vi "Run.vi"(8 "error in (no error)":errorcluster, 11 "Channel in":refnum<class "Channel.lvclass">) -> (0 "error out":errorcluster, 3 "Channel out":refnum<class "Channel.lvclass">)   [LabVIEW 2018, in "Channel.lvclass"]
uses:
  Channel.lvclass
  C:/Users/devstaff/sparc4/s4gui/Versao ZeroMQ REQ-REP/SPARC4_GUI -v1.0.0/Device/Device.lvclass
  Channel.lvclass/Channel.ctl
  Interface/Interface.lvclass/Interface.ctl
  Device/Device.lvclass/Device.ctl
  StateMachine/State Machine.lvclass
  Interface/Interface.lvclass
  Device/Device.lvclass
panel:
  out "resp RESUME":string
  out "resp PAUSE":string
  out "x = y?":T1
  out "resp ABORT":string
  out "resp STOP":string
  out "resposta do STATUS":string
  out "resp INIT":string
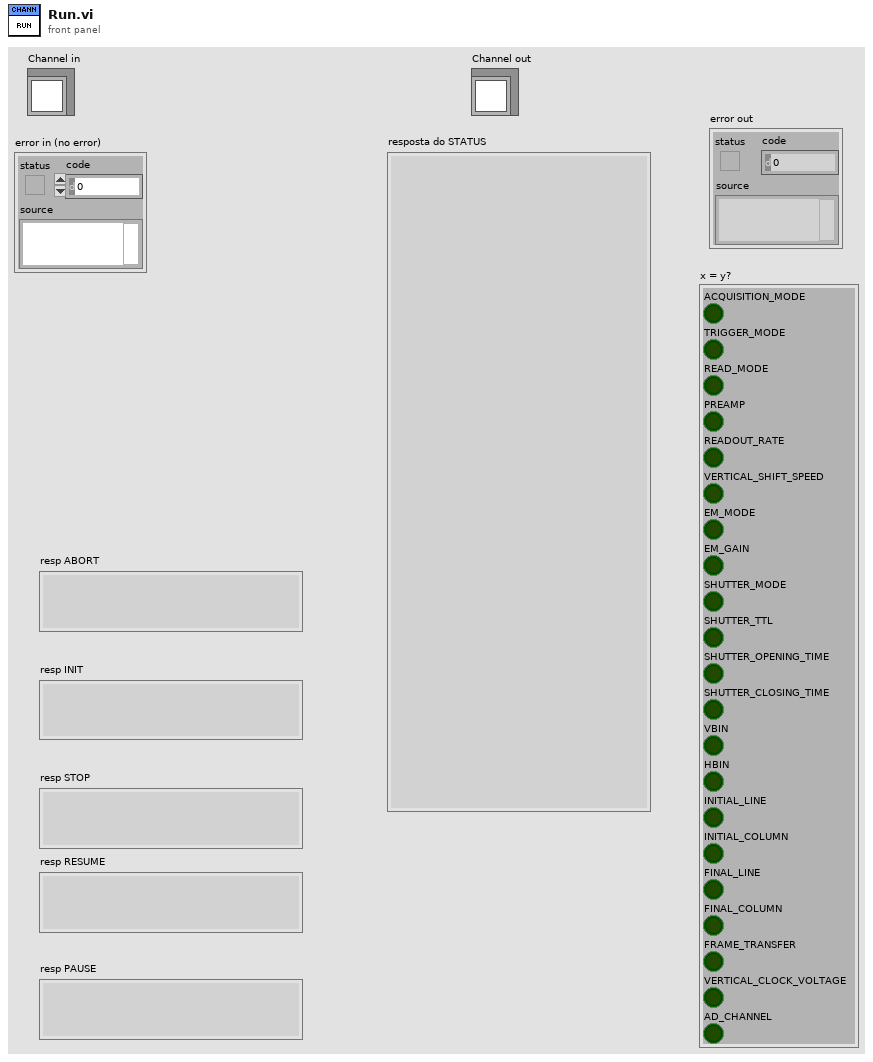
[diagram p1: front panel]
types:
  T1 = cluster{"ACQUISITION_MODE":bool, "TRIGGER_MODE":bool, "READ_MODE":bool, "PREAMP":bool, "READOUT_RATE":bool, "VERTICAL_SHIFT_SPEED":bool, "EM_MODE":bool, "EM_GAIN":bool, "SHUTTER_MODE":bool, "SHUTTER_TTL":bool, "SHUTTER_OPENING_TIME":bool, "SHUTTER_CLOSING_TIME":bool, "VBIN":bool, "HBIN":bool, "INITIAL_LINE":bool, "INITIAL_COLUMN":bool, "FINAL_LINE":bool, "FINAL_COLUMN":bool, "FRAME_TRANSFER":bool, "VERTICAL_CLOCK_VOLTAGE":bool, "AD_CHANNEL":bool}
  T2 = cluster{"TEMP":dbl, "EXPTIME":dbl, "#FRAMES":u32, "#CYCLES":u32, "#SEQS":u32, "WAVEPLATE_POS":u32, "COOLER_POWER_STATUS":dbl, "suffix":string}
  T3 = cluster{"ACQUISITION_MODE":u8, "TRIGGER_MODE":u8, "READ_MODE":u8, "PREAMP":u8, "READOUT_RATE":u8, "VERTICAL_SHIFT_SPEED":u8, "EM_MODE":u8, "EM_GAIN":u16, "SHUTTER_MODE":u8, "SHUTTER_TTL":u8, "SHUTTER_OPENING_TIME":u16, "SHUTTER_CLOSING_TIME":u16, "VBIN":u16, "HBIN":u16, "INITIAL_LINE":u16, "INITIAL_COLUMN":u16, "FINAL_LINE":u16, "FINAL_COLUMN":u16, "FRAME_TRANSFER":bool, "VERTICAL_CLOCK_VOLTAGE":u8, "AD_CHANNEL":u32}
  T4 = cluster{"Image Name":string, "Image Path":string, "#FRAMES":u32, "EXPTIME":dbl, "PREAMP":u8, "READOUT_RATE":u8, "VERTICAL_SHIFT_SPEED":u8, "ACQUISITION_MODE":u8, "READ_MODE":u8, "EM_MODE":u8, "EM_GAIN":u16, "SHUTTER_MODE":u8, "SHUTTER_TTL":u8, "SHUTTER_OPENNING_TIME":u16, "SHUTTER_CLOSING_TIME":u16, "VBIN":u16, "HBIN":u16, "INITIAL_LINE":u16, "INITIAL_COLUMN":u16, "FINAL_LINE":u16, "FINAL_COLUMN":u16, "Cooler ON/OFF":u16, "Set temperature":i8, "Exposições realizadas":u16, "Kinetic Serie Length":u32, "Number of Accumulations":u32, "Kinetic Cycle Time":u32, "FRAME_TRANSFER":bool, "VERTICAL_CLOCK_VOLTAGE":u8, "TRIGGER_MODE":u8, "Number of exp":u32, "AD_CHANNEL":u32}
  T5 = cluster{"OBSERVER":string, "OBJECT":string, "CTRLINTE":string, "PROJID":string, "SYNCMODE":string, "INSTMODE":string, "FILTER":string, "OBSTYPE":string, "CHANNEL 1":bool, "CHANNEL 2":bool, "CHANNEL 3":bool, "CHANNEL 4":bool, "TCSMODE":bool, "COMMENT":string, "broker":string, "GUIVRSN":string, "timestamp":string}
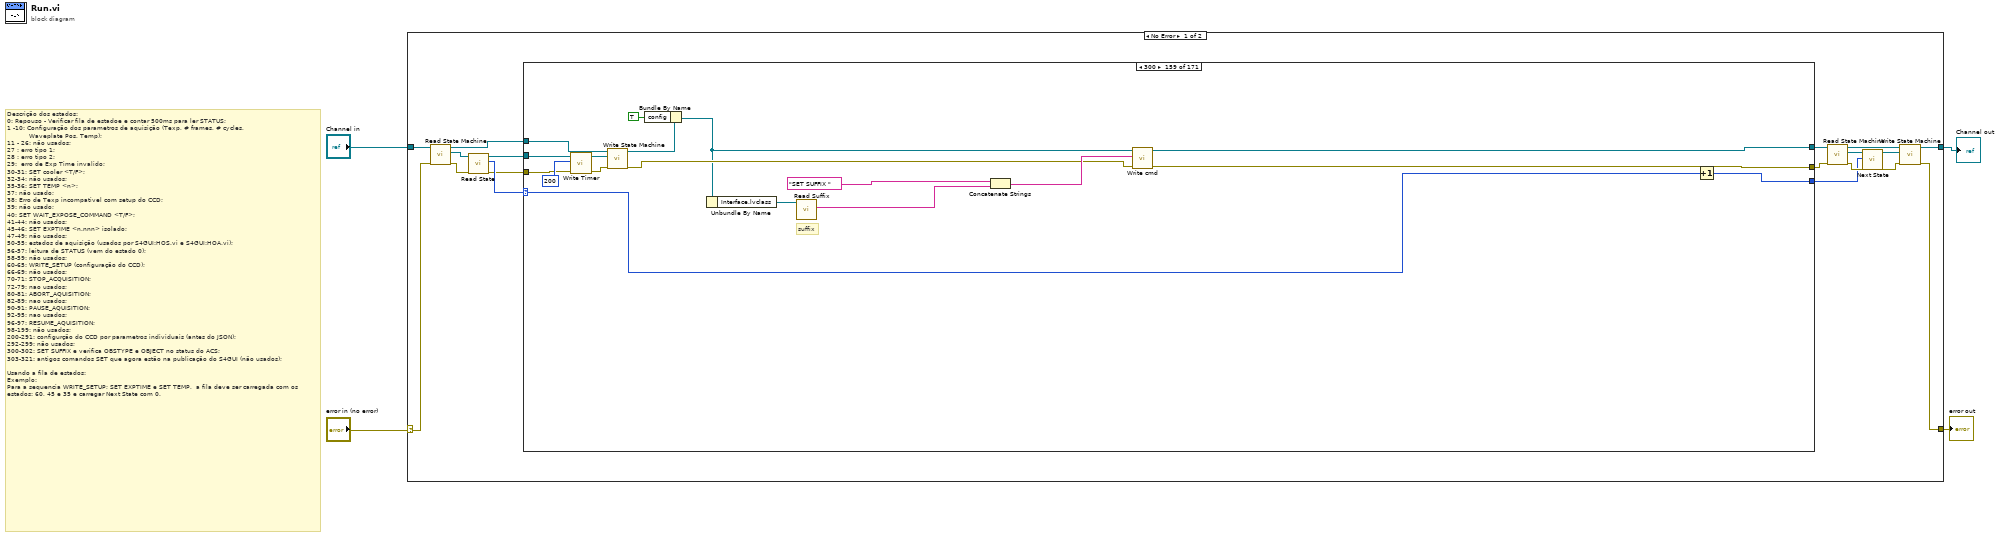
[diagram p0: block diagram]
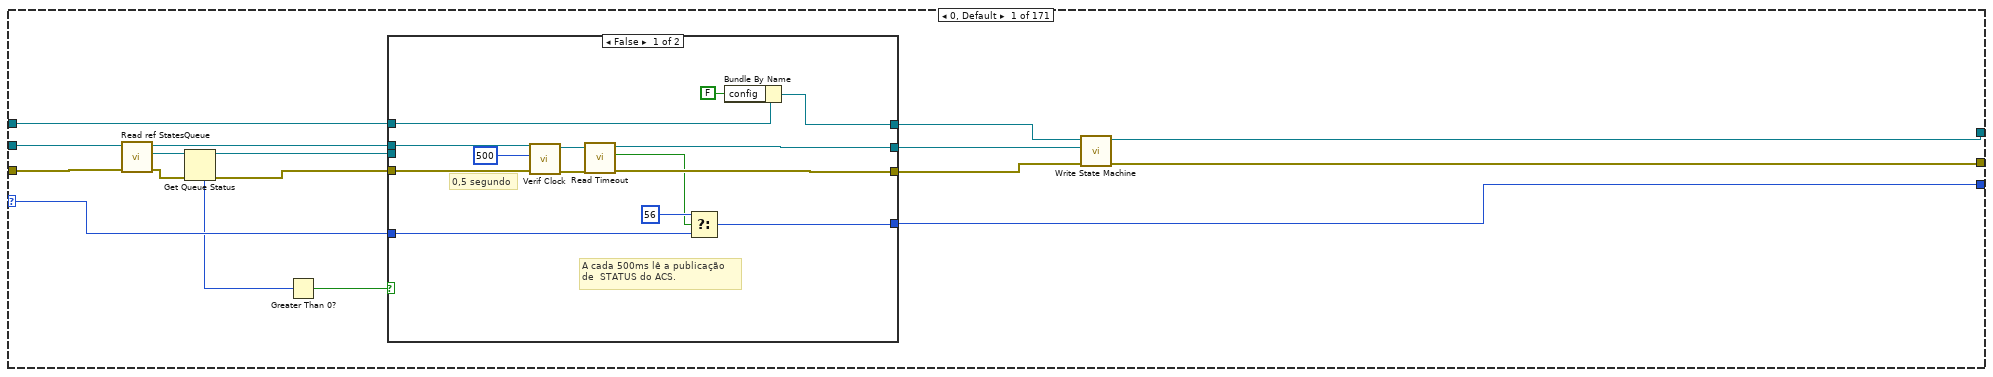
[diagram p2: hidden frame]
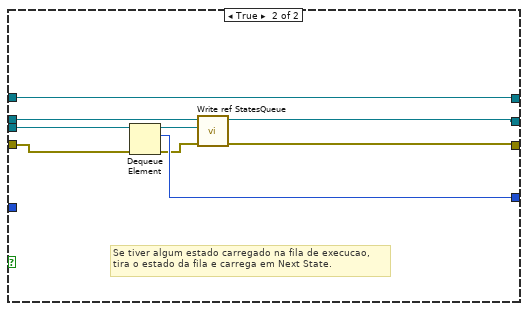
[diagram p3: hidden frame]
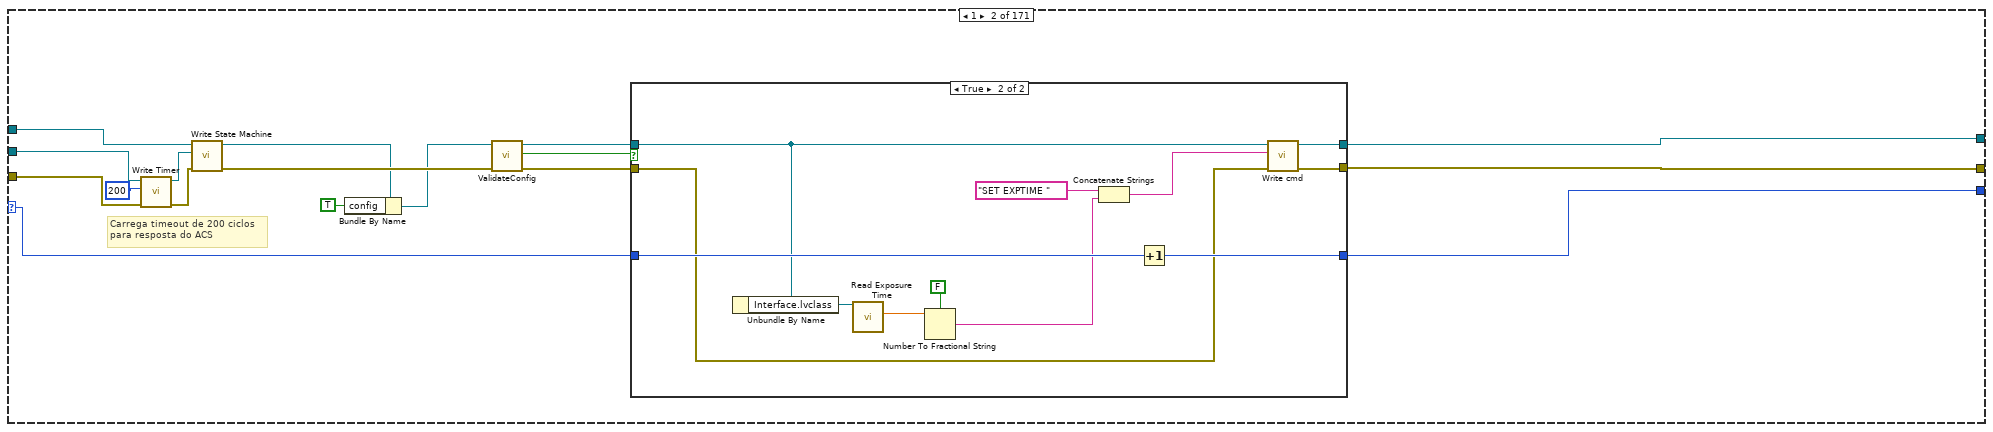
[diagram p4: hidden frame]
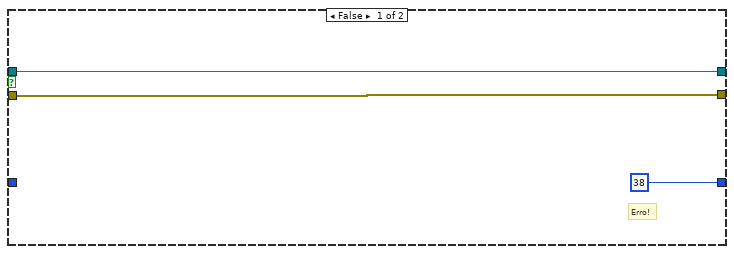
[diagram p5: hidden frame]
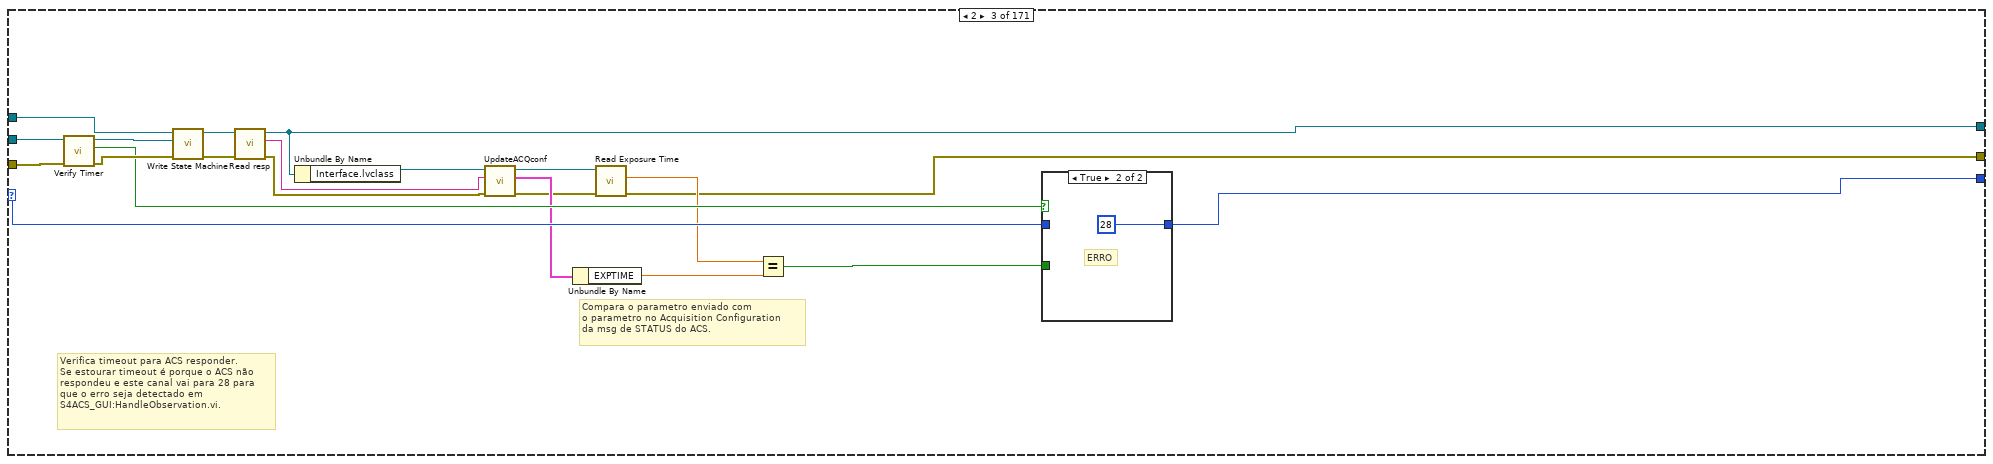
[diagram p6: hidden frame]
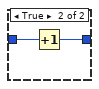
[diagram p8: hidden frame]
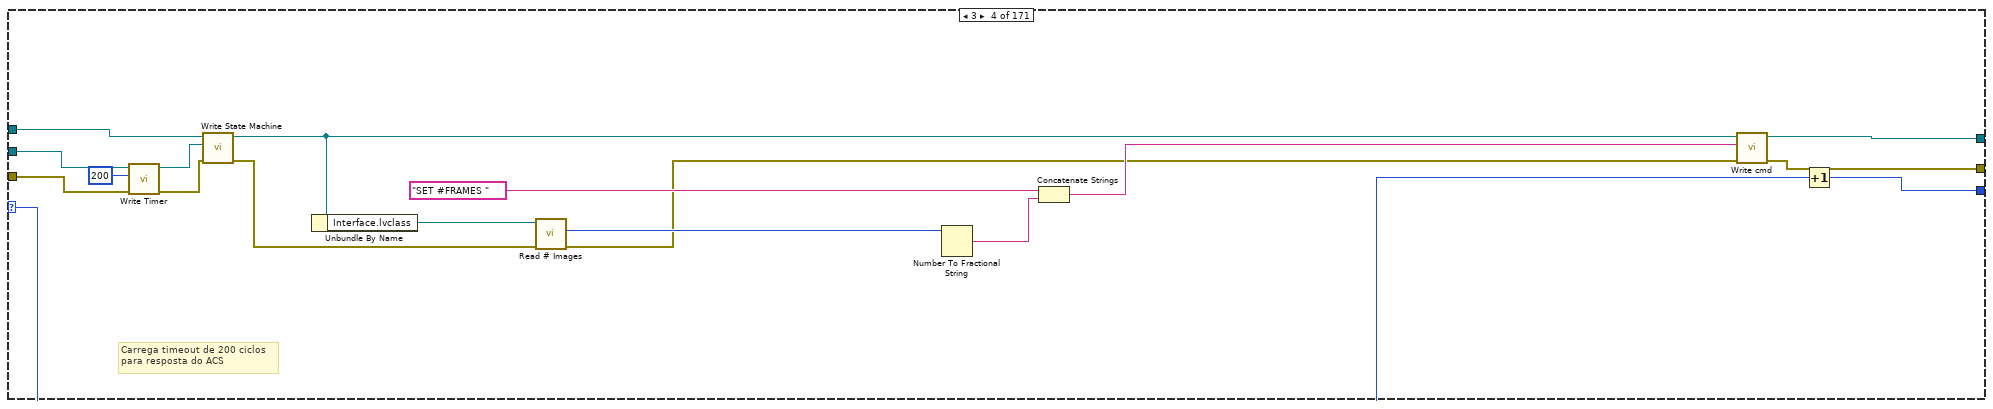
[diagram p9: hidden frame]
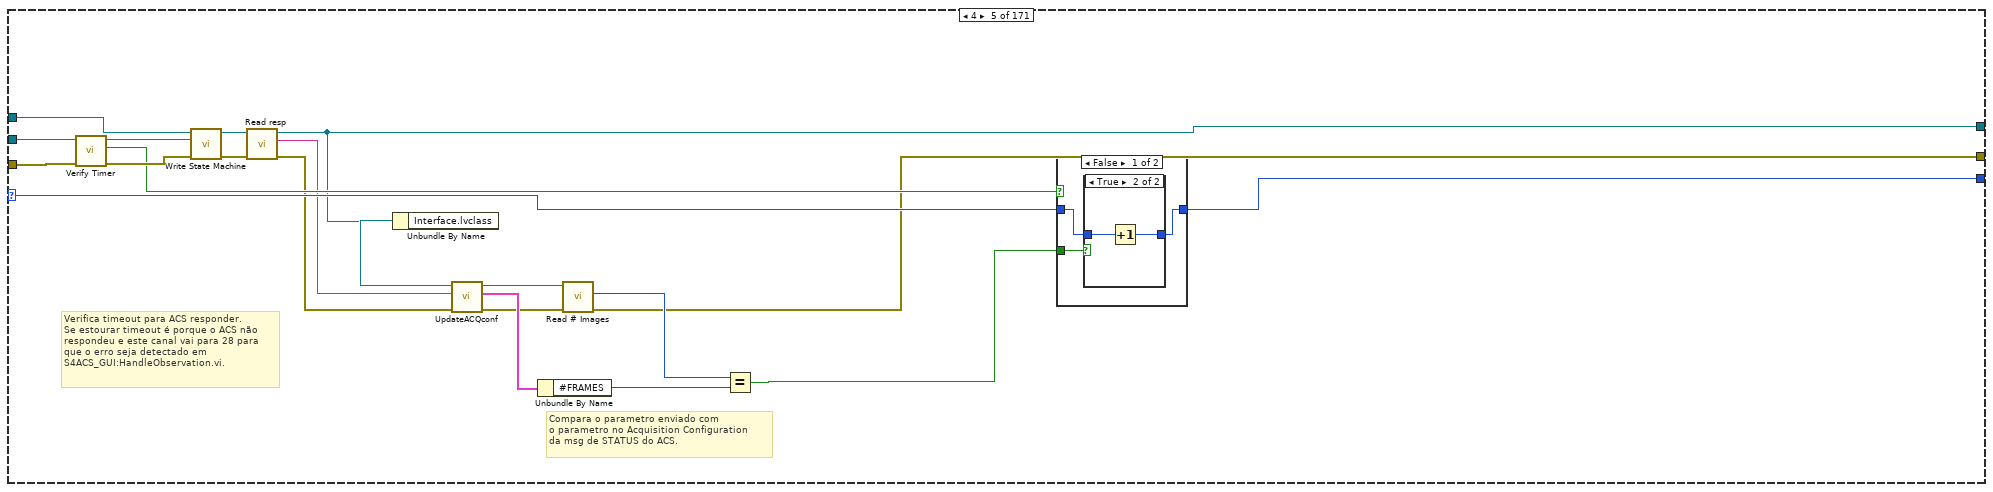
[diagram p10: hidden frame]
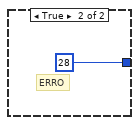
[diagram p12: hidden frame]
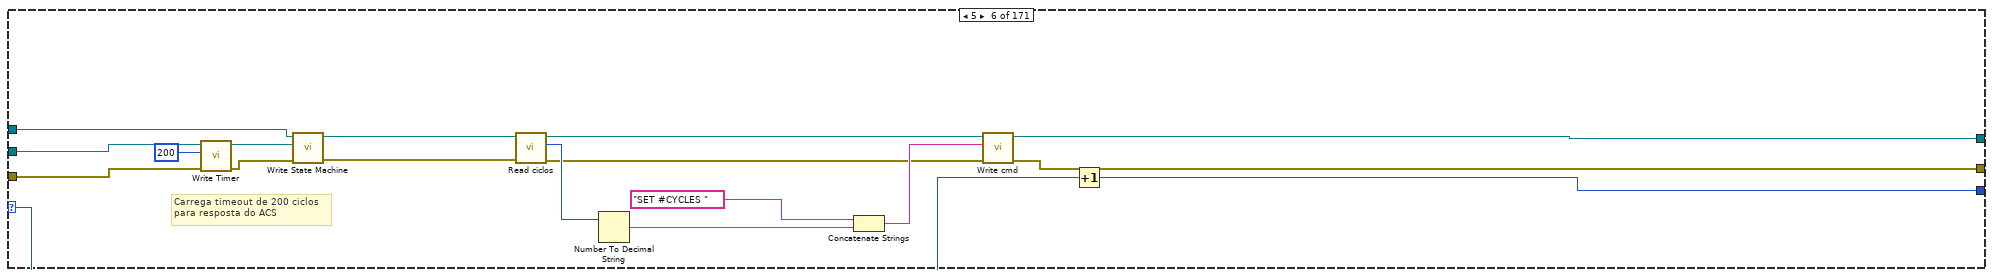
[diagram p13: hidden frame]
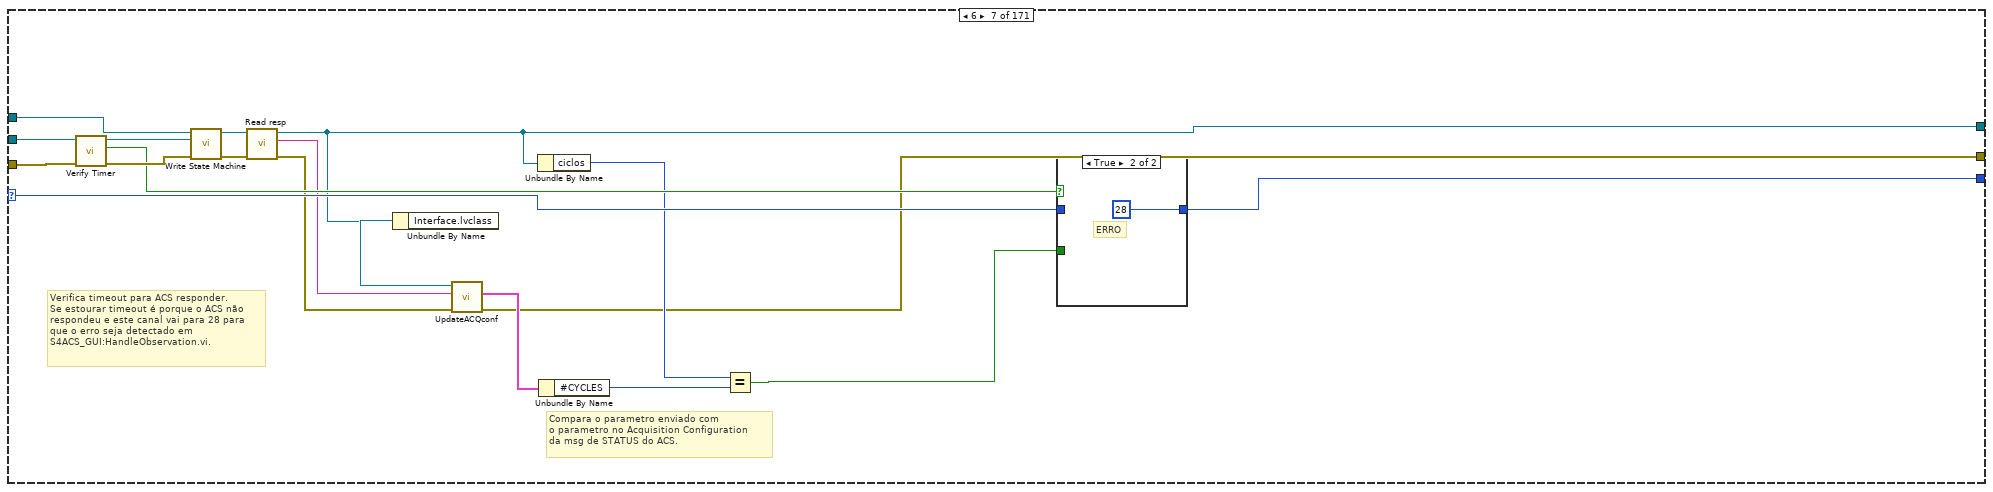
[diagram p14: hidden frame]
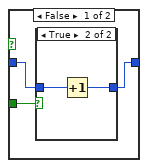
[diagram p15: hidden frame]
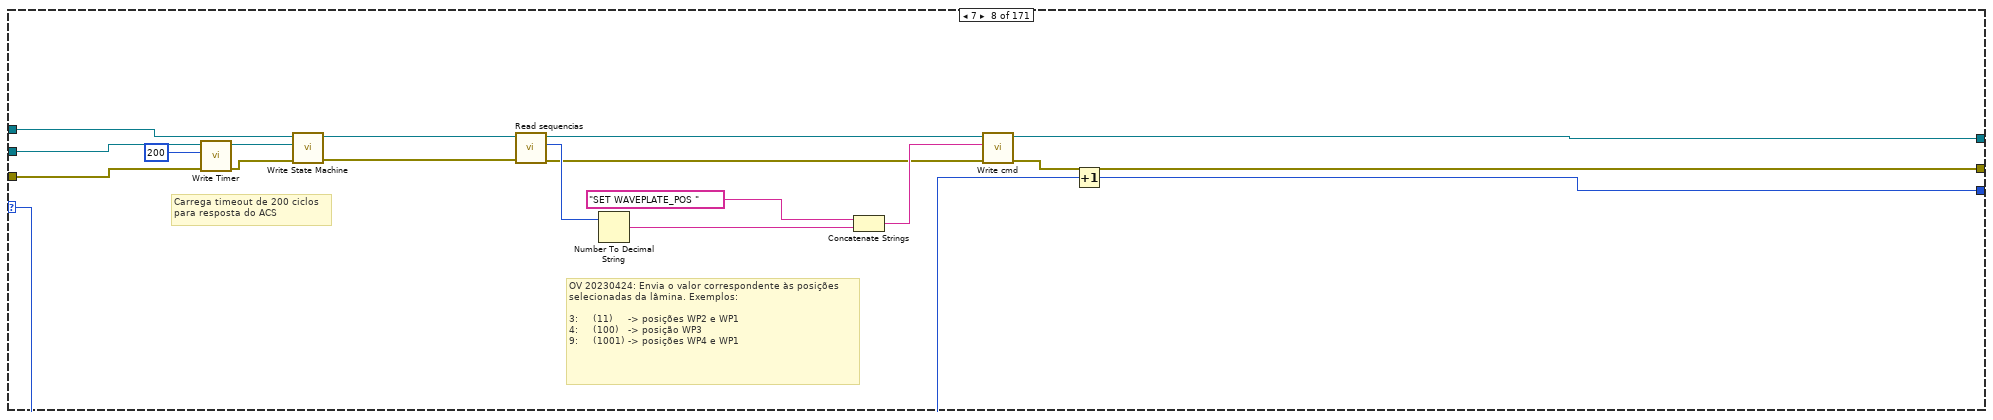
[diagram p17: hidden frame]
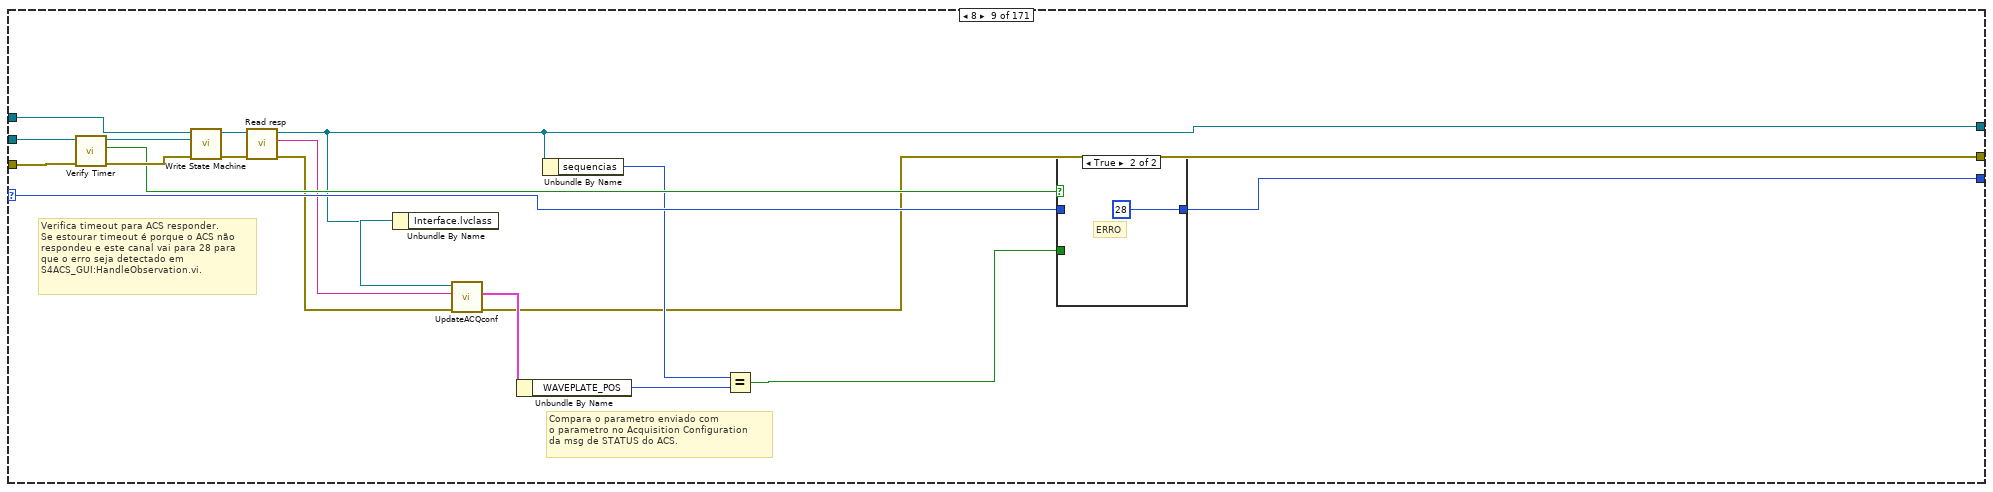
[diagram p18: hidden frame]
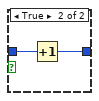
[diagram p20: hidden frame]
diagram:
  # "Descrição dos estados:\n0: Repouso - Verificar fila de estadoe e contar 500ms para ler STATUS;\n1 -10: Configuração dos parametros de aquisição (Texp, # frames, # cycles,\n           Waveplate Pos, Temp);\n11 - 26: não usados;\n27 : erro tipo 1;\n28 : erro tipo 2;\n29:  erro de Exp Time invalido;\n30-31: SET cooler <T/F>;\n32-34: não usados;\n35-36: SET TEMP <n>;\n37: não usado;\n38: Erro de Texp incompativel com setup do CCD;\n39: não usado;\n40: SET WAIT_EXPOSE_COMMAND <T/F>;\n41-44: não usados;\n45-46: SET EXPTIME <n.nnn> isolado;\n47-49: não usados;\n50-55: estados de aquisição (usados por S4GUI:HOS.vi e S4GUI:HOA.vi);\n56-57: leitura de STATUS (vem do estado 0);\n58-59: não usados;\n60-65: WRITE_SETUP (configuração do CCD);\n66-69: não usados;\n70-71: STOP_ACQUISITION;\n72-79: nao usados;\n80-81: ABORT_AQUISITION;\n82-89: nao usados;\n90-91: PAUSE_AQUISITION;\n92-95: nao usados;\n96-97: RESUME_AQUISITION;\n98-199: não usados;\n200-291: configurção do CCD por parametros individuais (antes do JSON);\n292-299: não usados;\n300-302: SET SUFFIX e verifica OBSTYPE e OBJECT no status do ACS;\n303-321: antigos comandos SET que agora estão na publicação do S4GUI (não usados);\n\nUsando a fila de estados:\nExemplo:\nPara a sequencia WRITE_SETUP; SET EXPTIME e SET TEMP,  a fila deve ser carregada com os \nestados: 60, 45 e 35 e carregar Next State com 0."
  n1 = case shown="No Error" "error in (no error)" {
    selector: "error in (no error)" -> [w21 w2964]
    tunnel: [w6 w2964] -> w3
    tunnel: [w11 w2963] -> w1
    tunnel: "Channel in" -> [w22 w2963]
    frame No Error {
      n2 = call-dynamic "Read State Machine.vi"("error in (no error)"=w21, "Device in"=w22) -> ("error out"=w18:errorcluster, "State Machine.lvclass"=w20:refnum<class "State Machine.lvclass">, "Device out"=w16:refnum<class "Channel.lvclass">)  [unwired: 7 in]
      n3 = call-dynamic "Read State.vi"("error in (no error)"=w18, "State Machine in"=w20) -> ("error out"=w17:errorcluster, "State"=w19:i32, "State Machine out"=w5:refnum<class "State Machine.lvclass">)  [unwired: 7 in]
      n4 = case shown="300" w19 {
        selector: w19 -> [w39 w76 w108 w125 w153 w177 w197 w221 w241 w265 w294 w308 w320 w350 w364 w389 w392 w395 w412 w440 w459 w472 w518 w547 _ w578 _ w619 w653 w679 w708 w719 w780 w801 w875 w915 w983 _ _ w1091 w1122 w1143 w1181 w1194 w1210 w1276 w1310 w1343 w1349 w1363 w1371 w1386 _ w1411 _ w1430 w1441 w1461 w1481 w1501 w1521 w1541 w1561 w1581 w1601 _ w1621 w1629 w1642 w1655 w1671 w1679 w1692 w1706 w1718 w1726 w1739 w1752 w1764 w1772 w1785 w1798 w1810 w1818 w1831 w1844 w1856 w1864 w1877 w1890 w1902 w1910 w1923 w1936 w1948 w1956 w1969 w1982 w1994 w2002 w2015 w2028 w2044 w2052 w2065 w2078 w2090 w2098 w2111 w2124 w2136 w2144 w2157 w2170 w2182 w2190 w2203 w2216 w2228 w2236 w2249 w2262 w2274 w2282 w2295 w2308 w2320 w2328 w2341 w2354 w2366 w2374 w2387 w2400 w2412 w2420 w2433 w2446 w2458 w2466 w2479 w2492 w2504 w2512 w2525 w2538 w2554 w2562 w2575 w2588 w2600 w2610 w2623 w2636 w2650 w2658 w2671 w2684 w2704 w2737 w2758 w2780 w2793 w2822 w2828 w2854 w2866 w2891 w2903 w2928 w2940]
        tunnel: w17 -> [w32 w75 w112 w127 w156 w179 w200 w223 w244 w262 w293 w310 w322 w352 w366 w391 w394 w397 w404 w439 w454 w466 w516 w546 w571 w580 w594 w618 w657 w676 w701 w717 w741 w798 w840 w908 w957 w1017 w1056 w1098 w1110 w1139 w1176 w1188 w1224 w1273 w1305 w1336 w1353 w1366 w1375 w1388 w1402 w1413 w1427 w1434 w1445 w1456 w1476 w1496 w1516 w1536 w1556 w1576 w1596 w1614 w1627 w1636 w1646 w1658 w1677 w1686 w1696 w1709 w1724 w1733 w1743 w1755 w1770 w1779 w1789 w1801 w1816 w1825 w1835 w1847 w1862 w1871 w1881 w1893 w1908 w1917 w1927 w1939 w1954 w1963 w1973 w1985 w2000 w2009 w2019 w2031 w2050 w2059 w2069 w2081 w2096 w2105 w2115 w2127 w2142 w2151 w2161 w2173 w2188 w2197 w2207 w2219 w2234 w2243 w2253 w2265 w2280 w2289 w2299 w2311 w2326 w2335 w2345 w2357 w2372 w2381 w2391 w2403 w2418 w2427 w2437 w2449 w2464 w2473 w2483 w2495 w2510 w2519 w2529 w2541 w2560 w2569 w2579 w2591 w2606 w2617 w2627 w2639 w2656 w2665 w2675 w2687 w2697 w2741 w2765 w2774 w2799 w2816 w2834 w2856 w2868 w2893 w2905 w2930 w2942]
        tunnel: [w35 w78 w95 w139 w141 w185 w187 w229 w231 w273 w276 w316 w329 w358 w373 w391 w394 w397 w416 w420 w461 w474 w526 w529 w576 w580 w598 w621 w640 w671 w695 w721 w772 w786 w850 w903 w958 w1029 w1067 w1097 w1123 w1144 w1173 w1196 w1211 w1278 w1292 w1324 w1350 w1359 w1372 w1383 w1400 w1408 w1422 w1433 w1442 w1456 w1476 w1496 w1516 w1536 w1556 w1576 w1596 w1614 w1626 w1630 w1645 w1656 w1676 w1680 w1695 w1707 w1723 w1727 w1742 w1753 w1769 w1773 w1788 w1799 w1815 w1819 w1834 w1845 w1861 w1865 w1880 w1891 w1907 w1911 w1926 w1937 w1953 w1957 w1972 w1983 w1999 w2003 w2018 w2029 w2049 w2053 w2068 w2079 w2095 w2099 w2114 w2125 w2141 w2145 w2160 w2171 w2187 w2191 w2206 w2217 w2233 w2237 w2252 w2263 w2279 w2283 w2298 w2309 w2325 w2329 w2344 w2355 w2371 w2375 w2390 w2401 w2417 w2421 w2436 w2447 w2463 w2467 w2482 w2493 w2509 w2513 w2528 w2539 w2559 w2563 w2578 w2589 w2605 w2611 w2626 w2637 w2655 w2659 w2674 w2685 w2708 w2723 w2761 w2783 w2802 w2824 w2837 w2862 w2875 w2899 w2912 w2936 w2949] -> w7
        tunnel: w16 -> [w24 w73 w115 w128 w160 w180 w204 w224 w248 w261 w292 w311 w326 w353 w370 w390 w393 w396 w407 w438 w456 w469 w515 w545 w574 w579 w595 w616 w660 w670 w707 w718 w754 w794 w849 w910 w951 w1028 w1066 w1092 w1114 w1137 w1177 w1189 w1225 w1272 w1308 w1337 w1354 w1365 w1376 w1380 w1403 w1405 w1428 w1432 w1446 w1454 w1474 w1494 w1514 w1534 w1554 w1574 w1594 w1616 w1625 w1637 w1644 w1659 w1675 w1687 w1694 w1710 w1722 w1734 w1741 w1756 w1768 w1780 w1787 w1802 w1814 w1826 w1833 w1848 w1860 w1872 w1879 w1894 w1906 w1918 w1925 w1940 w1952 w1964 w1971 w1986 w1998 w2010 w2017 w2032 w2048 w2060 w2067 w2082 w2094 w2106 w2113 w2128 w2140 w2152 w2159 w2174 w2186 w2198 w2205 w2220 w2232 w2244 w2251 w2266 w2278 w2290 w2297 w2312 w2324 w2336 w2343 w2358 w2370 w2382 w2389 w2404 w2416 w2428 w2435 w2450 w2462 w2474 w2481 w2496 w2508 w2520 w2527 w2542 w2558 w2570 w2577 w2592 w2604 w2618 w2625 w2640 w2654 w2666 w2673 w2688 w2698 w2744 w2764 w2776 w2800 w2818 w2835 w2857 w2872 w2894 w2909 w2931 w2946]
        tunnel: [w38 w79 w104 w140 w144 w186 w189 w230 w233 w266 w278 w317 w330 w359 w374 w390 w393 w396 w417 w421 w462 w477 w519 w531 w577 w579 w584 w622 w649 w672 w696 w722 w779 w787 w874 w904 w982 w1030 w1068 w1099 w1124 w1145 w1174 w1197 w1221 w1279 w1290 w1330 w1351 w1358 w1373 w1382 w1401 w1407 w1426 w1435 w1438 w1458 w1478 w1498 w1518 w1538 w1558 w1578 w1598 w1616 w1628 w1631 w1647 w1654 w1678 w1681 w1697 w1705 w1725 w1728 w1744 w1751 w1771 w1774 w1790 w1797 w1817 w1820 w1836 w1843 w1863 w1866 w1882 w1889 w1909 w1912 w1928 w1935 w1955 w1958 w1974 w1981 w2001 w2004 w2020 w2027 w2051 w2054 w2070 w2077 w2097 w2100 w2116 w2123 w2143 w2146 w2162 w2169 w2189 w2192 w2208 w2215 w2235 w2238 w2254 w2261 w2281 w2284 w2300 w2307 w2327 w2330 w2346 w2353 w2373 w2376 w2392 w2399 w2419 w2422 w2438 w2445 w2465 w2468 w2484 w2491 w2511 w2514 w2530 w2537 w2561 w2564 w2580 w2587 w2607 w2612 w2628 w2635 w2657 w2660 w2676 w2683 w2709 w2734 w2760 w2784 w2803 w2825 w2838 w2863 w2876 w2900 w2913 w2937 w2950] -> w14
        tunnel: [w34 w77 w107 w134 w152 w184 w196 w228 w240 w267 w295 w315 w321 w357 w362 w389 w392 w395 w413 w441 w460 w473 w520 w548 31 ("State") w578 w591 w620 w652 w677 w709 w720 w781 w802 w876 w916 w984 0 ("State") 54 ("State") w1090 w1125 w1142 w1182 w1195 w1209 w1277 w1311 w1344 w1352 w1364 w1374 w1387 0 ("State") w1412 0 ("State") w1431 w1443 w1453 w1473 w1493 w1513 w1533 w1553 w1573 w1593 u8 0 ("State") w1622 w1632 w1643 w1657 w1672 w1682 w1693 w1708 w1719 w1729 w1740 w1754 w1765 w1775 w1786 w1800 w1811 w1821 w1832 w1846 w1857 w1867 w1878 w1892 w1903 w1913 w1924 w1938 w1949 w1959 w1970 w1984 w1995 w2005 w2016 w2030 w2045 w2055 w2066 w2080 w2091 w2101 w2112 w2126 w2137 w2147 w2158 w2172 w2183 w2193 w2204 w2218 w2229 w2239 w2250 w2264 w2275 w2285 w2296 w2310 w2321 w2331 w2342 w2356 w2367 w2377 w2388 w2402 w2413 w2423 w2434 w2448 w2459 w2469 w2480 w2494 w2505 w2515 w2526 w2540 w2555 w2565 w2576 w2590 w2601 w2613 w2624 w2638 w2651 w2661 w2672 w2686 w2705 w2736 w2759 w2781 w2791 w2823 w2826 w2861 w2867 w2898 w2904 w2935 w2938] -> w8
        tunnel: w5 -> [w33 w74 w114 w129 w161 w178 w205 w222 w249 w263 w290 w309 w323 w351 w367 _ _ _ w406 w436 w455 w470 w514 w543 w573 _ w596 w617 w659 w675 w705 _ w744 w799 w842 w912 w956 w1018 w1057 w1094 w1115 w1140 w1178 w1191 w1226 w1274 w1309 w1338 _ _ _ _ _ _ _ _ _ _ _ _ _ _ _ _ _ _ _ _ _ _ _ _ _ _ _ _ _ _ _ _ _ _ _ _ _ _ _ _ _ _ _ _ _ _ _ _ _ _ _ _ _ _ _ _ _ _ _ _ _ _ _ _ _ _ _ _ _ _ _ _ _ _ _ _ _ _ _ _ _ _ _ _ _ _ _ _ _ _ _ _ _ _ _ _ _ _ _ _ _ _ _ _ _ _ _ _ _ _ w2700 w2743 w2766 w2772 w2797 w2815 w2832 w2855 w2869 w2892 w2906 w2929 w2943]
        frame 0, Default {
          n5 = call-dynamic "Read ref StatesQueue.vi"("error in (no error)"=w32, "State Machine in"=w33) -> ("error out"=w27:errorcluster, "ref StatesQueue"=w30:refnum<queue>, "State Machine out"=w31:refnum<class "State Machine.lvclass">)  [unwired: 7 in]
          n6 = Get Queue Status(queue=w30, error in (no error)=w27) -> (queue out=w25:refnum<queue>, error out=w26:errorcluster, # elements in queue=w29:i32)  [unwired: 1 in, 5 out]
          n7 = Greater Than 0?(x=w29) -> (x > 0?=w28:bool)
          n8 = case shown="False" w28 {
            tunnel: w39 -> [w49 _]
            tunnel: w31 -> [w48 w59]
            tunnel: w26 -> [w47 w61]
            tunnel: [w46 w55] -> w37
            tunnel: [w45 w56] -> w36
            tunnel: [w43 w60] -> w34
            tunnel: w25 -> [_ w62]
            tunnel: [w41 w54] -> w23
            tunnel: w24 -> [w42 w54]
            frame False {
              # "A cada 500ms lê a publicação \nde  STATUS do ACS."
              # "0,5 segundo"
              n9 = call-dynamic "Verif Clock.vi"("error in (no error)"=w47, "period (ms)"=u32 500 ("period"), "State Machine in"=w48) -> ("error out"=w52:errorcluster, "State Machine out"=w51:refnum<class "State Machine.lvclass">)  [unwired: 6 in, 1 out]
              n10 = call-dynamic "Read Timeout.vi"("error in (no error)"=w52, "State Machine in"=w51) -> ("error out"=w46:errorcluster, "Timeout"=w44:bool, "State Machine out"=w45:refnum<class "State Machine.lvclass">)  [unwired: 7 in]
              n11 = Select(t=56 ("State"), s=w44, f=w49) -> (s? t:f=w43:i32)
              n12 = Bundle By Name(cluster=w42, "config"=FALSE) -> (w41:refnum<class "Channel.lvclass">)
            }
            frame True {
              # "Se tiver algum estado carregado na fila de execucao,\ntira o estado da fila e carrega em Next State."
              n13 = Dequeue Element(queue=w62, error in (no error)=w61) -> (queue out=w58:refnum<queue>, element=w60:u32, error out=w57:errorcluster)  [unwired: 1 in, 1 out]
              n14 = call-dynamic "Write ref StatesQueue.vi"("error in (no error)"=w57, "ref StatesQueue"=w58, "State Machine in"=w59) -> ("error out"=w55:errorcluster, "State Machine out"=w56:refnum<class "State Machine.lvclass">)  [unwired: 7 in]
            }
          }
          n15 = call-dynamic "Write State Machine.vi"("error in (no error)"=w37, "State Machine.lvclass"=w36, "Device in"=w23) -> ("error out"=w35:errorcluster, "Device out"=w38:refnum<class "Channel.lvclass">)  [unwired: 7 in]
        }
        frame 1 {
          # "Carrega timeout de 200 ciclos\npara resposta do ACS"
          n16 = call-dynamic "Write Timer.vi"("error in (no error)"=w75, "Timer"=u32 200, "State Machine in"=w74) -> ("error out"=w70:errorcluster, "State Machine out"=w72:refnum<class "State Machine.lvclass">)  [unwired: 7 in]
          n17 = call-dynamic "Write State Machine.vi"("error in (no error)"=w70, "State Machine.lvclass"=w72, "Device in"=w73) -> ("error out"=w69:errorcluster, "Device out"=w65:refnum<class "Channel.lvclass">)  [unwired: 7 in]
          n18 = Bundle By Name(cluster=w65, "config"=TRUE) -> (w64:refnum<class "Channel.lvclass">)
          n19 = call-dynamic "ValidateConfig.vi"("error in (no error)"=w69, "Channel in"=w64) -> ("error out"=w67:errorcluster, "valid?"=w66:bool, "Channel out"=w68:refnum<class "Channel.lvclass">)  [unwired: 7 in]
          n20 = case shown="True" w66 {
            tunnel: [w82 w94] -> w79
            tunnel: [w81 w93] -> w78
            tunnel: [38 w92] -> w77
            tunnel: w76 -> [_ w91]
            tunnel: w68 -> [w82 w84]
            tunnel: w67 -> [w81 w83]
            frame False {
              # "Erro!"
            }
            frame True {
              n21 = Unbundle By Name(w84) -> ("Interface.lvclass"=w90:refnum<class "Interface.lvclass">)
              n22 = call "Read Exposure Time.vi"("Interface in"=w90) -> ("Exposure Time"=w89:dbl)  [unwired: 8 in, 2 out]
              n23 = Number To Fractional String(use system decimal point (T)=FALSE, number=w89) -> (F-format string=w88:string)  [unwired: 2 in]
              n24 = Concatenate Strings("SET EXPTIME " ("cmd"), w88) -> (w87:string)
              n25 = Increment(x=w91) -> (x+1=w92:i32)
              n26 = call-dynamic "Write cmd.vi"("error in (no error)"=w83, "cmd"=w87, "Device in"=w84) -> ("error out"=w93:errorcluster, "Device out"=w94:refnum<class "Channel.lvclass">)  [unwired: 7 in]
            }
          }
        }
        frame 2 {
          # "Compara o parametro enviado com\no parametro no Acquisition Configuration\nda msg de STATUS do ACS."
          # "Verifica timeout para ACS responder.\nSe estourar timeout é porque o ACS não \nrespondeu e este canal vai para 28 para \nque o erro seja detectado em\nS4ACS_GUI:HandleObservation.vi."
          n27 = call "Verify Timer.vi"("error in (no error)"=w112, "State Machine in"=w114) -> ("error out"=w111:errorcluster, "timeout"=w109:bool, "State Machine out"=w113:refnum<class "State Machine.lvclass">)  [unwired: 7 in]
          n28 = call-dynamic "Write State Machine.vi"("error in (no error)"=w111, "State Machine.lvclass"=w113, "Device in"=w115) -> ("error out"=w110:errorcluster, "Device out"=w106:refnum<class "Channel.lvclass">)  [unwired: 7 in]
          n29 = call-dynamic "Read resp.vi"("error in (no error)"=w110, "Device in"=w106) -> ("error out"=w97:errorcluster, "resp"=w105:string, "Device out"=w104:refnum<class "Channel.lvclass">)  [unwired: 7 in]
          n30 = Unbundle By Name(w104) -> ("Interface.lvclass"=w103:refnum<class "Interface.lvclass">)
          n31 = call-dynamic "UpdateACQconf.vi"("error in (no error)"=w97, "status"=w105, "Interface in"=w103) -> ("error out"=w96:errorcluster, "ACQ conf rx"=w101:T2, "Interface out"=w102:refnum<class "Interface.lvclass">)  [unwired: 6 in]
          n32 = Unbundle By Name(w101) -> ("EXPTIME"=w99:dbl)
          n33 = call "Read Exposure Time.vi"("error in (no error)"=w96, "Interface in"=w102) -> ("error out"=w95:errorcluster, "Exposure Time"=w100:dbl)  [unwired: 7 in, 1 out]
          n34 = Equal?(x=w100, y=w99) -> (x = y?=w98:bool)
          n35 = case shown="True" w109 {
            tunnel: [w117 28] -> w107
            tunnel: w108 -> [w118 _]
            tunnel: w98 -> [w116 _]
            frame False {
              n36 = case shown="False" w116 {
                tunnel: [w119 w120] -> w117
                tunnel: w118 -> [w119 w121]
                frame False {
                }
                frame True {
                  n37 = Increment(x=w121) -> (x+1=w120:i32)
                }
              }
            }
            frame True {
              # "ERRO"
            }
          }
        }
        frame 3 {
          # "Carrega timeout de 200 ciclos\npara resposta do ACS"
          n38 = call-dynamic "Write Timer.vi"("error in (no error)"=w127, "Timer"=u32 200, "State Machine in"=w129) -> ("error out"=w130:errorcluster, "State Machine out"=w132:refnum<class "State Machine.lvclass">)  [unwired: 7 in]
          n39 = call-dynamic "Write State Machine.vi"("error in (no error)"=w130, "State Machine.lvclass"=w132, "Device in"=w128) -> ("error out"=w124:errorcluster, "Device out"=w126:refnum<class "Channel.lvclass">)  [unwired: 7 in]
          n40 = Unbundle By Name(w126) -> ("Interface.lvclass"=w138:refnum<class "Interface.lvclass">)
          n41 = call-dynamic "Read # Images.vi"("error in (no error)"=w124, "Interface in"=w138) -> ("error out"=w123:errorcluster, "# Images"=w137:u32)  [unwired: 7 in, 1 out]
          n42 = Number To Fractional String(number=w137) -> (F-format string=w136:string)  [unwired: 3 in]
          n43 = Concatenate Strings("SET #FRAMES " ("cmd"), w136) -> (w135:string)
          n44 = call-dynamic "Write cmd.vi"("error in (no error)"=w123, "cmd"=w135, "Device in"=w126) -> ("error out"=w139:errorcluster, "Device out"=w140:refnum<class "Channel.lvclass">)  [unwired: 7 in]
          n45 = Increment(x=w125) -> (x+1=w134:i32)
        }
        frame 4 {
          # "Verifica timeout para ACS responder.\nSe estourar timeout é porque o ACS não \nrespondeu e este canal vai para 28 para \nque o erro seja detectado em\nS4ACS_GUI:HandleObservation.vi."
          # "Compara o parametro enviado com\no parametro no Acquisition Configuration\nda msg de STATUS do ACS."
          n46 = call "Verify Timer.vi"("error in (no error)"=w156, "State Machine in"=w161) -> ("error out"=w155:errorcluster, "timeout"=w154:bool, "State Machine out"=w157:refnum<class "State Machine.lvclass">)  [unwired: 7 in]
          n47 = call-dynamic "Write State Machine.vi"("error in (no error)"=w155, "State Machine.lvclass"=w157, "Device in"=w160) -> ("error out"=w158:errorcluster, "Device out"=w159:refnum<class "Channel.lvclass">)  [unwired: 7 in]
          n48 = call-dynamic "Read resp.vi"("error in (no error)"=w158, "Device in"=w159) -> ("error out"=w142:errorcluster, "resp"=w143:string, "Device out"=w144:refnum<class "Channel.lvclass">)  [unwired: 7 in]
          n49 = Unbundle By Name(w144) -> ("Interface.lvclass"=w151:refnum<class "Interface.lvclass">)
          n50 = call-dynamic "UpdateACQconf.vi"("error in (no error)"=w142, "status"=w143, "Interface in"=w151) -> ("error out"=w146:errorcluster, "ACQ conf rx"=w149:T2, "Interface out"=w150:refnum<class "Interface.lvclass">)  [unwired: 6 in]
          n51 = Unbundle By Name(w149) -> ("#FRAMES"=w147:u32)
          n52 = call-dynamic "Read # Images.vi"("error in (no error)"=w146, "Interface in"=w150) -> ("error out"=w141:errorcluster, "# Images"=w148:u32)  [unwired: 7 in, 1 out]
          n53 = Equal?(x=w148, y=w147) -> (x = y?=w145:bool)
          n54 = case shown="False" w154 {
            tunnel: [w163 28] -> w152
            tunnel: w153 -> [w164 _]
            tunnel: w145 -> [w162 _]
            frame False {
              n55 = case shown="True" w162 {
                tunnel: [w165 w166] -> w163
                tunnel: w164 -> [w165 w167]
                frame False {
                }
                frame True {
                  n56 = Increment(x=w167) -> (x+1=w166:i32)
                }
              }
            }
            frame True {
              # "ERRO"
            }
          }
        }
        frame 5 {
          # "Carrega timeout de 200 ciclos\npara resposta do ACS"
          n57 = call-dynamic "Write Timer.vi"("error in (no error)"=w179, "Timer"=u32 200, "State Machine in"=w178) -> ("error out"=w181:errorcluster, "State Machine out"=w183:refnum<class "State Machine.lvclass">)  [unwired: 7 in]
          n58 = call-dynamic "Write State Machine.vi"("error in (no error)"=w181, "State Machine.lvclass"=w183, "Device in"=w180) -> ("error out"=w175:errorcluster, "Device out"=w176:refnum<class "Channel.lvclass">)  [unwired: 7 in]
          n59 = call-dynamic "Read ciclos.vi"("error in (no error)"=w175, "Channel in"=w176) -> ("error out"=w169:errorcluster, "ciclos"=w173:u32, "Channel out"=w174:refnum<class "Channel.lvclass">)  [unwired: 7 in]
          n60 = Number To Decimal String(number=w173) -> (decimal integer string=w171:string)  [unwired: 1 in]
          n61 = Concatenate Strings("SET #CYCLES " ("cmd"), w171) -> (w170:string)
          n62 = call-dynamic "Write cmd.vi"("error in (no error)"=w169, "cmd"=w170, "Device in"=w174) -> ("error out"=w185:errorcluster, "Device out"=w186:refnum<class "Channel.lvclass">)  [unwired: 7 in]
          n63 = Increment(x=w177) -> (x+1=w184:i32)
        }
        frame 6 {
          # "Verifica timeout para ACS responder.\nSe estourar timeout é porque o ACS não \nrespondeu e este canal vai para 28 para \nque o erro seja detectado em\nS4ACS_GUI:HandleObservation.vi."
          # "Compara o parametro enviado com\no parametro no Acquisition Configuration\nda msg de STATUS do ACS."
          n64 = call "Verify Timer.vi"("error in (no error)"=w200, "State Machine in"=w205) -> ("error out"=w199:errorcluster, "timeout"=w198:bool, "State Machine out"=w201:refnum<class "State Machine.lvclass">)  [unwired: 7 in]
          n65 = call-dynamic "Write State Machine.vi"("error in (no error)"=w199, "State Machine.lvclass"=w201, "Device in"=w204) -> ("error out"=w202:errorcluster, "Device out"=w203:refnum<class "Channel.lvclass">)  [unwired: 7 in]
          n66 = call-dynamic "Read resp.vi"("error in (no error)"=w202, "Device in"=w203) -> ("error out"=w190:errorcluster, "resp"=w191:string, "Device out"=w189:refnum<class "Channel.lvclass">)  [unwired: 7 in]
          n67 = Unbundle By Name(w189) -> ("Interface.lvclass"=w195:refnum<class "Interface.lvclass">)
          n68 = call-dynamic "UpdateACQconf.vi"("error in (no error)"=w190, "status"=w191, "Interface in"=w195) -> ("error out"=w187:errorcluster, "ACQ conf rx"=w194:T2)  [unwired: 6 in, 1 out]
          n69 = Unbundle By Name(w189) -> ("ciclos"=w188:u32)
          n70 = Unbundle By Name(w194) -> ("#CYCLES"=w193:u32)
          n71 = Equal?(x=w188, y=w193) -> (x = y?=w192:bool)
          n72 = case shown="True" w198 {
            tunnel: [w207 28] -> w196
            tunnel: w197 -> [w208 _]
            tunnel: w192 -> [w206 _]
            frame False {
              n73 = case shown="True" w206 {
                tunnel: [w209 w210] -> w207
                tunnel: w208 -> [w209 w211]
                frame False {
                }
                frame True {
                  n74 = Increment(x=w211) -> (x+1=w210:i32)
                }
              }
            }
            frame True {
              # "ERRO"
            }
          }
        }
        frame 7 {
          # "OV 20230424: Envia o valor correspondente às posições\nselecionadas da lâmina. Exemplos:\n\n3:     (11)     -> posições WP2 e WP1\n4:     (100)   -> posição WP3\n9:     (1001) -> posições WP4 e WP1"
          # "Carrega timeout de 200 ciclos\npara resposta do ACS"
          n75 = call-dynamic "Write Timer.vi"("error in (no error)"=w223, "Timer"=u32 200, "State Machine in"=w222) -> ("error out"=w225:errorcluster, "State Machine out"=w227:refnum<class "State Machine.lvclass">)  [unwired: 7 in]
          n76 = call-dynamic "Write State Machine.vi"("error in (no error)"=w225, "State Machine.lvclass"=w227, "Device in"=w224) -> ("error out"=w219:errorcluster, "Device out"=w220:refnum<class "Channel.lvclass">)  [unwired: 7 in]
          n77 = call-dynamic "Read sequencias.vi"("error in (no error)"=w219, "Channel in"=w220) -> ("error out"=w213:errorcluster, "sequencias"=w217:u32, "Channel out"=w218:refnum<class "Channel.lvclass">)  [unwired: 7 in]
          n78 = Number To Decimal String(number=w217) -> (decimal integer string=w215:string)  [unwired: 1 in]
          n79 = Concatenate Strings("SET WAVEPLATE_POS " ("cmd"), w215) -> (w214:string)
          n80 = call-dynamic "Write cmd.vi"("error in (no error)"=w213, "cmd"=w214, "Device in"=w218) -> ("error out"=w229:errorcluster, "Device out"=w230:refnum<class "Channel.lvclass">)  [unwired: 7 in]
          n81 = Increment(x=w221) -> (x+1=w228:i32)
        }
        frame 8 {
          # "Verifica timeout para ACS responder.\nSe estourar timeout é porque o ACS não \nrespondeu e este canal vai para 28 para \nque o erro seja detectado em\nS4ACS_GUI:HandleObservation.vi."
          # "Compara o parametro enviado com\no parametro no Acquisition Configuration\nda msg de STATUS do ACS."
          n82 = call "Verify Timer.vi"("error in (no error)"=w244, "State Machine in"=w249) -> ("error out"=w243:errorcluster, "timeout"=w242:bool, "State Machine out"=w245:refnum<class "State Machine.lvclass">)  [unwired: 7 in]
          n83 = call-dynamic "Write State Machine.vi"("error in (no error)"=w243, "State Machine.lvclass"=w245, "Device in"=w248) -> ("error out"=w246:errorcluster, "Device out"=w247:refnum<class "Channel.lvclass">)  [unwired: 7 in]
          n84 = call-dynamic "Read resp.vi"("error in (no error)"=w246, "Device in"=w247) -> ("error out"=w234:errorcluster, "resp"=w235:string, "Device out"=w233:refnum<class "Channel.lvclass">)  [unwired: 7 in]
          n85 = Unbundle By Name(w233) -> ("Interface.lvclass"=w239:refnum<class "Interface.lvclass">)
          n86 = call-dynamic "UpdateACQconf.vi"("error in (no error)"=w234, "status"=w235, "Interface in"=w239) -> ("error out"=w231:errorcluster, "ACQ conf rx"=w238:T2)  [unwired: 6 in, 1 out]
          n87 = Unbundle By Name(w238) -> ("WAVEPLATE_POS"=w237:u32)
          n88 = Unbundle By Name(w233) -> ("sequencias"=w232:u32)
          n89 = Equal?(x=w232, y=w237) -> (x = y?=w236:bool)
          n90 = case shown="True" w242 {
            tunnel: [w251 28] -> w240
            tunnel: w241 -> [w252 _]
            tunnel: w236 -> [w250 _]
            frame False {
              n91 = case shown="False" w250 {
                tunnel: [w253 w254] -> w251
                tunnel: w252 -> [w253 w255]
                frame False {
                }
                frame True {
                  n92 = Increment(x=w255) -> (x+1=w254:i32)
                }
              }
            }
            frame True {
              # "ERRO"
            }
          }
        }
        frame 9 {
          # "Carrega timeout de 200 ciclos\npara resposta do ACS"
          n93 = call-dynamic "Write Timer.vi"("error in (no error)"=w262, "Timer"=u32 200, "State Machine in"=w263) -> ("error out"=w259:errorcluster, "State Machine out"=w260:refnum<class "State Machine.lvclass">)  [unwired: 7 in]
          n94 = call-dynamic "Write State Machine.vi"("error in (no error)"=w259, "State Machine.lvclass"=w260, "Device in"=w261) -> ("error out"=w257:errorcluster, "Device out"=w258:refnum<class "Channel.lvclass">)  [unwired: 7 in]
          n95 = Unbundle By Name(w258) -> ("Interface.lvclass"=w272:refnum<class "Interface.lvclass">)
          n96 = call-dynamic "Read Temperature.vi"("Interface in"=w272) -> ("Temperature"=w269:i8)  [unwired: 8 in, 2 out]
          n97 = Number To Decimal String(number=w269) -> (decimal integer string=w268:string)  [unwired: 1 in]
          n98 = Concatenate Strings("SET TEMP " ("cmd"), w268) -> (w271:string)
          n99 = call-dynamic "Write cmd.vi"("error in (no error)"=w257, "cmd"=w271, "Device in"=w258) -> ("error out"=w273:errorcluster, "Device out"=w266:refnum<class "Channel.lvclass">)  [unwired: 7 in]
          n100 = Increment(x=w265) -> (x+1=w267:i32)
        }
        frame 10 {
          # "Verifica timeout para ACS responder.\nSe estourar timeout é porque o ACS não \nrespondeu e este canal vai para 28 para \nque o erro seja detectado em\nS4ACS_GUI:HandleObservation.vi."
          n101 = call "Verify Timer.vi"("error in (no error)"=w293, "State Machine in"=w290) -> ("error out"=w288:errorcluster, "timeout"=w286:bool, "State Machine out"=w289:refnum<class "State Machine.lvclass">)  [unwired: 7 in]
          n102 = call-dynamic "Write State Machine.vi"("error in (no error)"=w288, "State Machine.lvclass"=w289, "Device in"=w292) -> ("error out"=w287:errorcluster, "Device out"=w291:refnum<class "Channel.lvclass">)  [unwired: 7 in]
          n103 = call-dynamic "Read resp.vi"("error in (no error)"=w287, "Device in"=w291) -> ("error out"=w277:errorcluster, "resp"=w279:string, "Device out"=w278:refnum<class "Channel.lvclass">)  [unwired: 7 in]
          n104 = Unbundle By Name(w278) -> ("Interface.lvclass"=w285:refnum<class "Interface.lvclass">)
          n105 = call-dynamic "UpdateACQconf.vi"("error in (no error)"=w277, "status"=w279, "Interface in"=w285) -> ("error out"=w281:errorcluster, "ACQ conf rx"=w284:T2, "Interface out"=w282:refnum<class "Interface.lvclass">)  [unwired: 6 in]
          n106 = Unbundle By Name(w284) -> ("TEMP"=w275:dbl)
          n107 = call-dynamic "Read Temperature.vi"("error in (no error)"=w281, "Interface in"=w282) -> ("error out"=w276:errorcluster, "Temperature"=w280:i8)  [unwired: 7 in, 1 out]
          n108 = To Byte Integer(number=w275) -> (8bit integer=w274:i8)
          n109 = Equal?(x=w280, y=w274) -> (x = y?=w283:bool)
          n110 = case shown="False" w286 {
            tunnel: w283 -> [w298 _]
            tunnel: [w297 28 ("State")] -> w295
            tunnel: w294 -> [w296 _]
            frame False {
              n111 = case shown="True" w298 {
                tunnel: [w299 0 ("State")] -> w297
                tunnel: w296 -> [w299 _]
                frame False {
                }
                frame True {
                  # "OV 2024-04-2: Apenas seta a temperatura, pois \ncooler já está ligado. Fim do setup inicial para aquisição."
                }
              }
            }
            frame True {
              # "ERRO"
              # "Estourou timeour e ACS não recebeu\no valor da temperatura desejada.\nAborta o processo com erro de \nconfiguração"
            }
          }
        }
        frame 11 {
          # "Carrega timeout de 50 ciclos\npara resposta do ACS"
          n112 = call-dynamic "Write Timer.vi"("error in (no error)"=w310, "Timer"=u32 50, "State Machine in"=w309) -> ("error out"=w312:errorcluster, "State Machine out"=w314:refnum<class "State Machine.lvclass">)  [unwired: 7 in]
          n113 = call-dynamic "Write State Machine.vi"("error in (no error)"=w312, "State Machine.lvclass"=w314, "Device in"=w311) -> ("error out"=w305:errorcluster, "Device out"=w304:refnum<class "Channel.lvclass">)  [unwired: 7 in]
          n114 = Unbundle By Name(w304) -> ("Channel Status"=w303:u32)
          n115 = Number To Decimal String(number=w303) -> (decimal integer string=w302:string)  [unwired: 1 in]
          n116 = Concatenate Strings("SET CHANNELSST " ("cmd"), w302) -> (w306:string)
          n117 = call-dynamic "Write cmd.vi"("error in (no error)"=w305, "cmd"=w306, "Device in"=w304) -> ("error out"=w316:errorcluster, "Device out"=w317:refnum<class "Channel.lvclass">)  [unwired: 7 in]
          n118 = Increment(x=w308) -> (x+1=w315:i32)
        }
        frame 12 {
          n119 = call "Verify Timer.vi"("error in (no error)"=w322, "State Machine in"=w323) -> ("error out"=w327:errorcluster, "timeout"=w319:bool, "State Machine out"=w328:refnum<class "State Machine.lvclass">)  [unwired: 7 in]
          n120 = call-dynamic "Write State Machine.vi"("error in (no error)"=w327, "State Machine.lvclass"=w328, "Device in"=w326) -> ("error out"=w324:errorcluster, "Device out"=w325:refnum<class "Channel.lvclass">)  [unwired: 7 in]
          n121 = call-dynamic "Read resp.vi"("error in (no error)"=w324, "Device in"=w325) -> ("error out"=w329:errorcluster, "resp"=w332:string, "Device out"=w330:refnum<class "Channel.lvclass">)  [unwired: 7 in]
          n122 = Equal?(x=w332, y="DONE") -> (x = y?=w318:bool)
          n123 = case shown="True" w319 {
            tunnel: [w334 w340] -> w321
            tunnel: w320 -> [w335 w339]
            tunnel: w318 -> [w333 _]
            frame False {
              n124 = case shown="True" w333 {
                tunnel: [w336 w337] -> w334
                tunnel: w335 -> [w336 w338]
                frame False {
                }
                frame True {
                  n125 = Increment(x=w338) -> (x+1=w337:i32)
                }
              }
            }
            frame True {
              n126 = disable-structure shown="Enabled" {
                disable-tunnel: [28 w342] -> w340
                disable-tunnel: w339 -> [_ w343]
                frame Enabled {
                  # "ERRO"
                }
                frame Disabled {
                  # "Por enquanto, prossegue\nmesmo sem receber DONE."
                  n127 = Increment(x=w343) -> (x+1=w342:i32)
                }
              }
            }
          }
        }
        frame 13 {
          # "Carrega timeout de 50 ciclos\npara resposta do ACS"
          n128 = call-dynamic "Write Timer.vi"("error in (no error)"=w352, "Timer"=u32 50, "State Machine in"=w351) -> ("error out"=w354:errorcluster, "State Machine out"=w356:refnum<class "State Machine.lvclass">)  [unwired: 7 in]
          n129 = call-dynamic "Write State Machine.vi"("error in (no error)"=w354, "State Machine.lvclass"=w356, "Device in"=w353) -> ("error out"=w347:errorcluster, "Device out"=w346:refnum<class "Channel.lvclass">)  [unwired: 7 in]
          n130 = Unbundle By Name(w346) -> ("syncmode"=w345:bool)
          n131 = case shown="False" w345 {
            tunnel: ["ASYNC" "SYNC"] -> w344
            frame False {
            }
            frame True {
            }
          }
          n132 = Concatenate Strings("SET SYNCMODE " ("cmd"), w344) -> (w348:string)
          n133 = call-dynamic "Write cmd.vi"("error in (no error)"=w347, "cmd"=w348, "Device in"=w346) -> ("error out"=w358:errorcluster, "Device out"=w359:refnum<class "Channel.lvclass">)  [unwired: 7 in]
          n134 = Increment(x=w350) -> (x+1=w357:i32)
        }
        frame 14 {
          n135 = call "Verify Timer.vi"("error in (no error)"=w366, "State Machine in"=w367) -> ("error out"=w371:errorcluster, "timeout"=w365:bool, "State Machine out"=w372:refnum<class "State Machine.lvclass">)  [unwired: 7 in]
          n136 = call-dynamic "Write State Machine.vi"("error in (no error)"=w371, "State Machine.lvclass"=w372, "Device in"=w370) -> ("error out"=w368:errorcluster, "Device out"=w369:refnum<class "Channel.lvclass">)  [unwired: 7 in]
          n137 = call-dynamic "Read resp.vi"("error in (no error)"=w368, "Device in"=w369) -> ("error out"=w373:errorcluster, "resp"=w376:string, "Device out"=w374:refnum<class "Channel.lvclass">)  [unwired: 7 in]
          n138 = Equal?(x=w376, y="DONE") -> (x = y?=w363:bool)
          n139 = case shown="True" w365 {
            tunnel: [w378 w386] -> w362
            tunnel: w364 -> [w379 _]
            tunnel: w363 -> [w377 _]
            frame False {
              n140 = case shown="True" w377 {
                tunnel: [w380 w381] -> w378
                tunnel: w379 -> [w380 w382]
                frame False {
                }
                frame True {
                  n141 = disable-structure shown="Enabled" {
                    disable-tunnel: w382 -> [w384 _]
                    disable-tunnel: [w383 29 ("State")] -> w381
                    frame Disabled {
                      n142 = Increment(x=w384) -> (x+1=w383:i32)
                    }
                    frame Enabled {
                    }
                  }
                }
              }
            }
            frame True {
              n143 = disable-structure shown="Enabled" {
                disable-tunnel: [28 29] -> w386
                frame Enabled {
                  # "ERRO"
                }
                frame Disabled {
                  # "Por enquanto, prossegue\nmesmo sem receber DONE."
                }
              }
            }
          }
        }
        frame 27 {
          # "ESTADO DE ERRO: Falha na configuraçãodo sufixo: vide estados 300 e 301."
        }
        frame 28 {
          # "ESTADO DE ERRO: Fica aqui até que S4GUI:HandleObservationSync.vi ou S4GUI:HandleObservationAsync.vi ou os botões START, STOP, ABORT mandem para outro estado."
        }
        frame 29 {
          # "ESTADO DE ERRO:  Exp Time inválido!"
        }
        frame 30 {
          # "OV20241125: Valor de COOLER é o target:\nSe =1  manda ligar,\nSe =0  manda desligar."
          n144 = call-dynamic "Write Timer.vi"("error in (no error)"=w404, "Timer"=u32 50, "State Machine in"=w406) -> ("error out"=w403:errorcluster, "State Machine out"=w405:refnum<class "State Machine.lvclass">)  [unwired: 7 in]
          n145 = call-dynamic "Write State Machine.vi"("error in (no error)"=w403, "State Machine.lvclass"=w405, "Device in"=w407) -> ("error out"=w402:errorcluster, "Device out"=w400:refnum<class "Channel.lvclass">)  [unwired: 7 in]
          n146 = Bundle By Name(cluster=w400, "config"=TRUE) -> (w399:refnum<class "Channel.lvclass">)
          n147 = Unbundle By Name(w399) -> ("Interface.lvclass"=w415:refnum<class "Interface.lvclass">)
          n148 = call-dynamic "Read Cooler ON_OFF.vi"("error in (no error)"=w402, "Interface in"=w415) -> ("error out"=w401:errorcluster, "Cooler ON/OFF"=w410:i16)  [unwired: 7 in, 1 out]
          n149 = case shown="0" w410 {
            tunnel: ["0" "1"] -> w409
            frame 0 {
              (unwired) "OFF"
            }
            frame 1, Default {
              (unwired) "ON"
            }
          }
          n150 = Concatenate Strings("SET COOLER_POWER_STATUS " ("cmd"), w409) -> (w414:string)
          n151 = call-dynamic "Write cmd.vi"("error in (no error)"=w401, "cmd"=w414, "Device in"=w399) -> ("error out"=w416:errorcluster, "Device out"=w417:refnum<class "Channel.lvclass">)  [unwired: 7 in]
          n152 = Increment(x=w412) -> (x+1=w413:i32)
        }
        frame 31 {
          n153 = call "Verify Timer.vi"("error in (no error)"=w439, "State Machine in"=w436) -> ("error out"=w434:errorcluster, "timeout"=w432:bool, "State Machine out"=w435:refnum<class "State Machine.lvclass">)  [unwired: 7 in]
          n154 = call-dynamic "Write State Machine.vi"("error in (no error)"=w434, "State Machine.lvclass"=w435, "Device in"=w438) -> ("error out"=w433:errorcluster, "Device out"=w437:refnum<class "Channel.lvclass">)  [unwired: 7 in]
          n155 = call-dynamic "Read resp.vi"("error in (no error)"=w433, "Device in"=w437) -> ("error out"=w422:errorcluster, "resp"=w423:string, "Device out"=w421:refnum<class "Channel.lvclass">)  [unwired: 7 in]
          n156 = Unbundle By Name(w421) -> ("Interface.lvclass"=w431:refnum<class "Interface.lvclass">)
          n157 = call-dynamic "UpdateACQconf.vi"("error in (no error)"=w422, "status"=w423, "Interface in"=w431) -> ("error out"=w428:errorcluster, "ACQ conf rx"=w430:T2, "Interface out"=w429:refnum<class "Interface.lvclass">)  [unwired: 6 in]
          n158 = Unbundle By Name(w430) -> ("COOLER_POWER_STATUS"=w426:dbl)
          n159 = call-dynamic "Read Cooler ON_OFF.vi"("error in (no error)"=w428, "Interface in"=w429) -> ("error out"=w420:errorcluster, "Cooler ON/OFF"=w427:i16)  [unwired: 7 in, 1 out]
          n160 = To Word Integer(number=w426) -> (16bit integer=w425:i16)
          n161 = Equal?(x=w427, y=w425) -> (x = y?=w424:bool)
          n162 = case shown="False" w432 {
            tunnel: w424 -> [w444 _]
            tunnel: [w443 w447] -> w441
            tunnel: w440 -> [w442 _]
            frame False {
              n163 = case shown="True" w444 {
                tunnel: [w445 0 ("State")] -> w443
                tunnel: w442 -> [w445 _]
                frame False {
                }
                frame True {
                }
              }
            }
            frame True {
              n164 = disable-structure shown="Enabled" {
                disable-tunnel: [0 ("State") 28 ("State")] -> w447
                frame Disabled {
                }
                frame Enabled {
                  # "erro"
                }
              }
            }
          }
        }
        frame 32 {
          # "Este estado não é mais usado!!"
          n165 = call-dynamic "Write Timer.vi"("error in (no error)"=w454, "Timer"=u32 50, "State Machine in"=w455) -> ("error out"=w457:errorcluster, "State Machine out"=w452:refnum<class "State Machine.lvclass">)  [unwired: 7 in]
          n166 = call-dynamic "Write State Machine.vi"("error in (no error)"=w457, "State Machine.lvclass"=w452, "Device in"=w456) -> ("error out"=w450:errorcluster, "Device out"=w451:refnum<class "Channel.lvclass">)  [unwired: 7 in]
          n167 = call-dynamic "Write cmd.vi"("error in (no error)"=w450, "cmd"="GET COOLER_POWER_STATUS ", "Device in"=w451) -> ("error out"=w461:errorcluster, "Device out"=w462:refnum<class "Channel.lvclass">)  [unwired: 7 in]
          n168 = Increment(x=w459) -> (x+1=w460:i32)
        }
        frame 33 {
          # "Este estado não é mais usado!!"
          n169 = call "Verify Timer.vi"("error in (no error)"=w466, "State Machine in"=w470) -> ("error out"=w465:errorcluster, "timeout"=w464:bool, "State Machine out"=w467:refnum<class "State Machine.lvclass">)  [unwired: 7 in]
          n170 = call-dynamic "Write State Machine.vi"("error in (no error)"=w465, "State Machine.lvclass"=w467, "Device in"=w469) -> ("error out"=w463:errorcluster, "Device out"=w468:refnum<class "Channel.lvclass">)  [unwired: 7 in]
          n171 = call-dynamic "Read resp.vi"("error in (no error)"=w463, "Device in"=w468) -> ("error out"=w475:errorcluster, "resp"=w471:string, "Device out"=w476:refnum<class "Channel.lvclass">)  [unwired: 7 in]
          n172 = case shown="False" w464 {
            tunnel: [w484 w505] -> w477
            tunnel: w476 -> [w483 w505]
            tunnel: w475 -> [w482 w504]
            tunnel: [w481 w504] -> w474
            tunnel: [w480 w503] -> w473
            tunnel: w472 -> [w479 _]
            tunnel: w471 -> [w478 _]
            frame False {
              n173 = case shown="\"0\", \"1\"" w478 {
                selector: w478 -> [_ w496]
                tunnel: [w487 w492] -> w484
                tunnel: w483 -> [w487 w500]
                tunnel: w482 -> [w486 w498]
                tunnel: [w486 w490] -> w481
                tunnel: [w485 w497] -> w480
                tunnel: w479 -> [w485 _]
                frame Default {
                }
                frame "0", "1" {
                  n174 = Decimal String To Number(string=w496) -> (number=w495:i32)  [unwired: 2 in, 1 out]
                  n175 = Unbundle By Name(w500) -> ("Interface.lvclass"=w499:refnum<class "Interface.lvclass">)
                  n176 = To Word Integer(number=w495) -> (16bit integer=w494:i16)
                  n177 = call-dynamic "Write Cooler ON_OFF.vi"("error in (no error)"=w498, "Cooler ON/OFF"=w494, "Interface in"=w499) -> ("error out"=w491:errorcluster, "Interface out"=w489:refnum<class "Interface.lvclass">)  [unwired: 7 in]
                  n178 = Bundle By Name(cluster=w500, "Interface.lvclass"=w489) -> (w493:refnum<class "Channel.lvclass">)
                  n179 = disable-structure shown="Enabled" {
                    disable-tunnel: [0 ("State") 45 ("State")] -> w497
                    frame Disabled {
                    }
                    frame Enabled {
                      (unwired) 300 ("State")
                      # "40: configura os\nparametros por comando\nSET TEXP e WAIT EXPOSE"
                    }
                  }
                  n180 = call-dynamic "Save Temp.vi"("error in (no error)"=w491, "temp file"="lasttemp.cfg", "Channel in"=w493) -> ("error out"=w490:errorcluster, "Channel out"=w492:refnum<class "Channel.lvclass">)  [unwired: 7 in]
                }
              }
            }
            frame True {
              n181 = disable-structure shown="Enabled" {
                disable-tunnel: [0 ("State") 45 ("State")] -> w503
                frame Disabled {
                }
                frame Enabled {
                  (unwired) 300 ("State")
                  # "45: configura os\nparametros por comando\nSET TEXP e WAIT EXPOSE"
                }
              }
            }
          }
        }
        frame 35 {
          # "Carrega timeout de 50 ciclos\n50 x 20ms = 1s\npara resposta do ACS"
          n182 = call-dynamic "Write Timer.vi"("error in (no error)"=w516, "Timer"=u32 50, "State Machine in"=w514) -> ("error out"=w512:errorcluster, "State Machine out"=w513:refnum<class "State Machine.lvclass">)  [unwired: 7 in]
          n183 = call-dynamic "Write State Machine.vi"("error in (no error)"=w512, "State Machine.lvclass"=w513, "Device in"=w515) -> ("error out"=w511:errorcluster, "Device out"=w510:refnum<class "Channel.lvclass">)  [unwired: 7 in]
          n184 = Bundle By Name(cluster=w510, "config"=TRUE) -> (w509:refnum<class "Channel.lvclass">)
          n185 = Unbundle By Name(w509) -> ("Interface.lvclass"=w525:refnum<class "Interface.lvclass">)
          n186 = call-dynamic "Read Temperature.vi"("Interface in"=w525) -> ("Temperature"=w522:i8)  [unwired: 8 in, 2 out]
          n187 = Number To Decimal String(number=w522) -> (decimal integer string=w521:string)  [unwired: 1 in]
          n188 = Concatenate Strings("SET TEMP " ("cmd"), w521) -> (w524:string)
          n189 = call-dynamic "Write cmd.vi"("error in (no error)"=w511, "cmd"=w524, "Device in"=w509) -> ("error out"=w526:errorcluster, "Device out"=w519:refnum<class "Channel.lvclass">)  [unwired: 7 in]
          n190 = Increment(x=w518) -> (x+1=w520:i32)
        }
        frame 36 {
          n191 = call "Verify Timer.vi"("error in (no error)"=w546, "State Machine in"=w543) -> ("error out"=w541:errorcluster, "timeout"=w539:bool, "State Machine out"=w542:refnum<class "State Machine.lvclass">)  [unwired: 7 in]
          n192 = call-dynamic "Write State Machine.vi"("error in (no error)"=w541, "State Machine.lvclass"=w542, "Device in"=w545) -> ("error out"=w540:errorcluster, "Device out"=w544:refnum<class "Channel.lvclass">)  [unwired: 7 in]
          n193 = call-dynamic "Read resp.vi"("error in (no error)"=w540, "Device in"=w544) -> ("error out"=w530:errorcluster, "resp"=w532:string, "Device out"=w531:refnum<class "Channel.lvclass">)  [unwired: 7 in]
          n194 = Unbundle By Name(w531) -> ("Interface.lvclass"=w538:refnum<class "Interface.lvclass">)
          n195 = call-dynamic "UpdateACQconf.vi"("error in (no error)"=w530, "status"=w532, "Interface in"=w538) -> ("error out"=w534:errorcluster, "ACQ conf rx"=w537:T2, "Interface out"=w535:refnum<class "Interface.lvclass">)  [unwired: 6 in]
          n196 = Unbundle By Name(w537) -> ("TEMP"=w528:dbl)
          n197 = call-dynamic "Read Temperature.vi"("error in (no error)"=w534, "Interface in"=w535) -> ("error out"=w529:errorcluster, "Temperature"=w533:i8)  [unwired: 7 in, 1 out]
          n198 = To Byte Integer(number=w528) -> (8bit integer=w527:i8)
          n199 = Equal?(x=w533, y=w527) -> (x = y?=w536:bool)
          n200 = case shown="False" w539 {
            tunnel: w536 -> [w551 _]
            tunnel: [w550 w558] -> w548
            tunnel: w547 -> [w549 _]
            frame False {
              n201 = case shown="True" w551 {
                tunnel: [w552 w553] -> w550
                tunnel: w549 -> [w552 w554]
                frame False {
                }
                frame True {
                  # "OV 2022-11-16: Ao setar a temperatura, liga \nautomaticamente o COLLER."
                  n202 = disable-structure shown="Enabled" {
                    disable-tunnel: w554 -> [w556 _]
                    disable-tunnel: [w555 0] -> w553
                    frame Disabled {
                      n203 = Increment(x=w556) -> (x+1=w555:i32)
                    }
                    frame Enabled {
                    }
                  }
                }
              }
            }
            frame True {
              n204 = disable-structure shown="Enabled" {
                disable-tunnel: [0 ("State") 28 ("State")] -> w558
                frame Disabled {
                }
                frame Enabled {
                  (unwired) 300 ("State")
                  (unwired) 45 ("State")
                  # "erro"
                  # "45: configura os\nparametros por comando\nSET SUFFIX e\nWAIT_EXPOSE_COMMAND"
                }
              }
            }
          }
        }
        frame 37 {
          w565 = i16 1 items=["Cooler OFF", "Cooler ON"] ("Cooler ON/OFF")
          # "Liga COOLER"
          n205 = call-dynamic "Write Timer.vi"("error in (no error)"=w571, "Timer"=u32 50, "State Machine in"=w573) -> ("error out"=w570:errorcluster, "State Machine out"=w572:refnum<class "State Machine.lvclass">)  [unwired: 7 in]
          n206 = call-dynamic "Write State Machine.vi"("error in (no error)"=w570, "State Machine.lvclass"=w572, "Device in"=w574) -> ("error out"=w566:errorcluster, "Device out"=w563:refnum<class "Channel.lvclass">)  [unwired: 7 in]
          n207 = Unbundle By Name(w563) -> ("Interface.lvclass"=w567:refnum<class "Interface.lvclass">)
          n208 = call-dynamic "Write Cooler ON_OFF.vi"("error in (no error)"=w566, "Cooler ON/OFF"=w565, "Interface in"=w567) -> ("error out"=w564:errorcluster, "Interface out"=w562:refnum<class "Interface.lvclass">)  [unwired: 7 in]
          n209 = Bundle By Name(cluster=w563, "Interface.lvclass"=w562) -> (w561:refnum<class "Channel.lvclass">)
          n210 = call-dynamic "Write cmd.vi"("error in (no error)"=w564, "cmd"="SET COOLER_POWER_STATUS 1", "Device in"=w561) -> ("error out"=w576:errorcluster, "Device out"=w577:refnum<class "Channel.lvclass">)  [unwired: 7 in]
        }
        frame 38 {
          # "ESTADO DE ERRO: Texp incompativel com a configuração do CCD;\nFica aqui até que S4GUI:HandleObservationSync.vi ou S4GUI:HandleObservationAsync.vi ou os botões START, STOP, ABORT mandem para outro estado."
        }
        frame 40 {
          n211 = disable-structure shown="Disabled" {
            disable-tunnel: [w605 w607] -> w597
            disable-tunnel: w596 -> [w603 w607]
            disable-tunnel: w594 -> [w602 w606]
            disable-tunnel: [w601 w606] -> w593
            frame Disabled {
              # "Carrega timeout de 10 ciclos\npara resposta do ACS"
              n212 = call-dynamic "Write Timer.vi"("error in (no error)"=w602, "Timer"=u32 10, "State Machine in"=w603) -> ("error out"=w601:errorcluster, "State Machine out"=w605:refnum<class "State Machine.lvclass">)  [unwired: 7 in]
            }
            frame Enabled {
            }
          }
          n213 = call-dynamic "Write State Machine.vi"("error in (no error)"=w593, "State Machine.lvclass"=w597, "Device in"=w595) -> ("error out"=w592:errorcluster, "Device out"=w583:refnum<class "Channel.lvclass">)  [unwired: 7 in]
          n214 = Bundle By Name(cluster=w583, "config"=TRUE) -> (w582:refnum<class "Channel.lvclass">)
          n215 = Unbundle By Name(w582) -> ("wait_expose"=w589:bool)
          n216 = Select(t="ON", s=w589, f="OFF") -> (s? t:f=w586:string)
          n217 = Concatenate Strings("WAIT_EXPOSE_COMMAND " ("cmd"), w586) -> (w585:string)
          n218 = call-dynamic "Write cmd.vi"("error in (no error)"=w592, "cmd"=w585, "Device in"=w582) -> ("error out"=w598:errorcluster, "Device out"=w584:refnum<class "Channel.lvclass">)  [unwired: 7 in]
          n219 = disable-structure shown="Enabled" {
            disable-tunnel: [0 ("State") 45 ("State")] -> w591
            frame Enabled {
            }
            frame Disabled {
              # "Termina o processo, \nconfigurando a Texp \ndos canais."
            }
          }
        }
        frame 45 {
          # "Carrega timeout de 200 ciclos\npara resposta do ACS"
          n220 = call-dynamic "Write Timer.vi"("error in (no error)"=w618, "Timer"=u32 200, "State Machine in"=w617) -> ("error out"=w613:errorcluster, "State Machine out"=w615:refnum<class "State Machine.lvclass">)  [unwired: 7 in]
          n221 = call-dynamic "Write State Machine.vi"("error in (no error)"=w613, "State Machine.lvclass"=w615, "Device in"=w616) -> ("error out"=w611:errorcluster, "Device out"=w612:refnum<class "Channel.lvclass">)  [unwired: 7 in]
          n222 = call-dynamic "ValidateConfig.vi"("error in (no error)"=w611, "Channel in"=w612) -> ("error out"=w609:errorcluster, "valid?"=w608:bool, "Channel out"=w610:refnum<class "Channel.lvclass">)  [unwired: 7 in]
          n223 = case shown="True" w608 {
            tunnel: [w625 w639] -> w622
            tunnel: [w624 w638] -> w621
            tunnel: [29 w637] -> w620
            tunnel: w619 -> [_ w636]
            tunnel: w610 -> [w625 w628]
            tunnel: w609 -> [w624 w629]
            frame False {
              # "Erro!"
            }
            frame True {
              n224 = Bundle By Name(cluster=w628, "config"=TRUE) -> (w627:refnum<class "Channel.lvclass">)
              n225 = Unbundle By Name(w627) -> ("Interface.lvclass"=w635:refnum<class "Interface.lvclass">)
              n226 = call "Read Exposure Time.vi"("Interface in"=w635) -> ("Exposure Time"=w634:dbl)  [unwired: 8 in, 2 out]
              n227 = Number To Fractional String(use system decimal point (T)=FALSE, number=w634) -> (F-format string=w633:string)  [unwired: 2 in]
              n228 = Concatenate Strings("SET EXPTIME " ("cmd"), w633) -> (w632:string)
              n229 = Increment(x=w636) -> (x+1=w637:i32)
              n230 = call-dynamic "Write cmd.vi"("error in (no error)"=w629, "cmd"=w632, "Device in"=w627) -> ("error out"=w638:errorcluster, "Device out"=w639:refnum<class "Channel.lvclass">)  [unwired: 7 in]
            }
          }
        }
        frame 46 {
          # "Compara o parametro enviado com\no parametro no Acquisition Configuration\nda msg de STATUS do ACS."
          # "Verifica timeout para ACS responder.\nSe estourar timeout é porque o ACS não \nrespondeu e este canal vai para 28 para \nque o erro seja detectado em\nS4ACS_GUI:HandleObservation.vi."
          n231 = call "Verify Timer.vi"("error in (no error)"=w657, "State Machine in"=w659) -> ("error out"=w656:errorcluster, "timeout"=w654:bool, "State Machine out"=w658:refnum<class "State Machine.lvclass">)  [unwired: 7 in]
          n232 = call-dynamic "Write State Machine.vi"("error in (no error)"=w656, "State Machine.lvclass"=w658, "Device in"=w660) -> ("error out"=w655:errorcluster, "Device out"=w651:refnum<class "Channel.lvclass">)  [unwired: 7 in]
          n233 = call-dynamic "Read resp.vi"("error in (no error)"=w655, "Device in"=w651) -> ("error out"=w642:errorcluster, "resp"=w650:string, "Device out"=w649:refnum<class "Channel.lvclass">)  [unwired: 7 in]
          n234 = Unbundle By Name(w649) -> ("Interface.lvclass"=w648:refnum<class "Interface.lvclass">)
          n235 = call-dynamic "UpdateACQconf.vi"("error in (no error)"=w642, "status"=w650, "Interface in"=w648) -> ("error out"=w641:errorcluster, "ACQ conf rx"=w646:T2, "Interface out"=w647:refnum<class "Interface.lvclass">)  [unwired: 6 in]
          n236 = Unbundle By Name(w646) -> ("EXPTIME"=w644:dbl)
          n237 = call "Read Exposure Time.vi"("error in (no error)"=w641, "Interface in"=w647) -> ("error out"=w640:errorcluster, "Exposure Time"=w645:dbl)  [unwired: 7 in, 1 out]
          n238 = Equal?(x=w645, y=w644) -> (x = y?=w643:bool)
          n239 = case shown="True" w654 {
            tunnel: [w662 29] -> w652
            tunnel: w653 -> [w663 _]
            tunnel: w643 -> [w661 _]
            frame False {
              n240 = case shown="True" w661 {
                tunnel: [w664 0 ("State")] -> w662
                tunnel: w663 -> [w664 _]
                frame False {
                }
                frame True {
                  (unwired) 40 ("State")
                  # "Ajusta WAIT_\nEXPOSE_\nCOMMAND"
                }
              }
            }
            frame True {
              # "ERRO"
            }
          }
        }
        frame 50 {
          # "Durante a exposição, garantir config=F"
          n241 = Bundle By Name(cluster=w670, "stopping"=FALSE, "config"=FALSE) -> (w669:refnum<class "Channel.lvclass">)
          n242 = call-dynamic "Write cmd.vi"("error in (no error)"=w676, "cmd"="EXPOSE", "Device in"=w669) -> ("error out"=w673:errorcluster, "Device out"=w674:refnum<class "Channel.lvclass">)  [unwired: 7 in]
          n243 = disable-structure shown="Enabled" {
            disable-tunnel: w679 -> [w683 w686]
            disable-tunnel: [w680 w684] -> w677
            disable-tunnel: w675 -> [_ w693]
            disable-tunnel: w674 -> [w682 w691]
            disable-tunnel: w673 -> [w681 w689]
            disable-tunnel: [w682 w690] -> w672
            disable-tunnel: [w681 w687] -> w671
            frame Disabled {
              # "OV 2024-03-12:\nVai para a pausa antes\ndo pedido de STATUS"
              n244 = Increment(x=w683) -> (x+1=w680:i32)
            }
            frame Enabled {
              # "Força a recarga do Ticks com\no valor do relógio do PC.\n\n2024-03-20: Nao precisa mais \npedir STATUS, pois ACS o publica\na cada 1s."
              n245 = call-dynamic "Verif Clock.vi"("error in (no error)"=w689, "period (ms)"=u32 1 ("period"), "State Machine in"=w693) -> ("error out"=w688:errorcluster, "State Machine out"=w692:refnum<class "State Machine.lvclass">)  [unwired: 6 in, 1 out]
              n246 = Add(x=w686, y=3) -> (x+y=w684:i32)
              n247 = call-dynamic "Write State Machine.vi"("error in (no error)"=w688, "State Machine.lvclass"=w692, "Device in"=w691) -> ("error out"=w687:errorcluster, "Device out"=w690:refnum<class "Channel.lvclass">)  [unwired: 7 in]
            }
          }
        }
        frame 51 {
          # "ESTADO OPCIONAL:\nEspera estourar o timeout (200ms).\nApós o timeout vai para o próximo estado enviar STATUS para confirmar\nse o ACS  foi para ACTIVE."
          n248 = call-dynamic "Verif Clock.vi"("error in (no error)"=w701, "period (ms)"=u32 200 ("period"), "State Machine in"=w705) -> ("error out"=w700:errorcluster, "State Machine out"=w704:refnum<class "State Machine.lvclass">)  [unwired: 6 in, 1 out]
          n249 = call-dynamic "Read Timeout.vi"("error in (no error)"=w700, "State Machine in"=w704) -> ("error out"=w699:errorcluster, "Timeout"=w702:bool, "State Machine out"=w703:refnum<class "State Machine.lvclass">)  [unwired: 7 in]
          n250 = call-dynamic "Write State Machine.vi"("error in (no error)"=w699, "State Machine.lvclass"=w703, "Device in"=w707) -> ("error out"=w698:errorcluster, "Device out"=w697:refnum<class "Channel.lvclass">)  [unwired: 7 in]
          n251 = case shown="True" w702 {
            tunnel: [w712 w715] -> w709
            tunnel: w708 -> [w712 w716]
            tunnel: w698 -> [w710 w713]
            tunnel: w697 -> [w711 w714]
            tunnel: [w711 w714] -> w696
            tunnel: [w710 w713] -> w695
            frame False {
            }
            frame True {
              n252 = Increment(x=w716) -> (x+1=w715:i32)
            }
          }
        }
        frame 52 {
          n253 = disable-structure shown="Enabled" {
            disable-tunnel: [w727 w729] -> w722
            disable-tunnel: [w726 w728] -> w721
            disable-tunnel: w718 -> [w724 w729]
            disable-tunnel: w717 -> [w723 w728]
            frame Disabled {
              n254 = call-dynamic "Write cmd.vi"("error in (no error)"=w723, "cmd"="STATUS", "Device in"=w724) -> ("error out"=w726:errorcluster, "Device out"=w727:refnum<class "Channel.lvclass">)  [unwired: 7 in]
            }
            frame Enabled {
              # "ACS publica STATUS"
            }
          }
          n255 = Increment(x=w719) -> (x+1=w720:i32)
        }
        frame 53 {
          # "OV 2024.11.04: \nSe detectou ACTIVE, vai direto para estado 55, \npois o estado 54 foi eliminado.\nSe o ACTIVE for muito rápido e STATUS voltar para IDLE ou WAITING..., \nS4GUI:HandleObservationSync.vi detecta o incremento do CyclesDone.\nO mesmo para S4GUI:HandleObservationAsync.vi."
          # "Status.Texp = Current frame exptime\nlastStatus = cam status (acquiring, idle, writing, reading, ...)\nStatus.Nimages = frames done\nStatus.CubesDone = ciclos realizados pelo ACS\nStatus.SequesDone = sequencias realizadas pelo ACS.\nStatus.UsedDiskSpace = espaco usado no disco.\nStatus.Error = Se TRUE, houve erro na aquisição do canal."
          # "Verifica timeout para ACS iniciar exposição.\nSe estourar timeout é porque o ACS não \nrecebeu o EXPOSE e então volta para 50\npara enviar novo EXPOSE."
          # "Extrair todos os parametros da respsota de STATUS e\natualizar a informação na classe Channel."
          n256 = call-dynamic "Verif Clock.vi"("error in (no error)"=w741, "period (ms)"=u32 500 ("period"), "State Machine in"=w744) -> ("error out"=w742:errorcluster, "State Machine out"=w743:refnum<class "State Machine.lvclass">)  [unwired: 6 in, 1 out]
          n257 = call-dynamic "Read Timeout.vi"("error in (no error)"=w742, "State Machine in"=w743) -> ("error out"=w755:errorcluster, "Timeout"=w745:bool, "State Machine out"=w756:refnum<class "State Machine.lvclass">)  [unwired: 7 in]
          n258 = call-dynamic "Write State Machine.vi"("error in (no error)"=w755, "State Machine.lvclass"=w756, "Device in"=w754) -> ("error out"=w752:errorcluster, "Device out"=w753:refnum<class "Channel.lvclass">)  [unwired: 7 in]
          n259 = call-dynamic "Read resp.vi"("error in (no error)"=w752, "Device in"=w753) -> ("error out"=w774:errorcluster, "resp"=w775:string, "Device out"=w778:refnum<class "Channel.lvclass">)  [unwired: 7 in]
          "resposta do STATUS" <- w775
          n260 = call-dynamic "Read Interface.vi"("error in (no error)"=w774, "Channel in"=w778) -> ("error out"=w773:errorcluster, "Interface.lvclass"=w776:refnum<class "Interface.lvclass">, "Channel out"=w777:refnum<class "Channel.lvclass">)  [unwired: 7 in]
          n261 = call-dynamic "UpdateStatus.vi"("error in (no error)"=w773, "status"=w775, "Interface in"=w776) -> ("error out"=w732:errorcluster, "Interface out"=w734:refnum<class "Interface.lvclass">)  [unwired: 7 in]
          n262 = call-dynamic "Read Error.vi"("error in (no error)"=w732, "Interface in"=w734) -> ("error out"=w731:errorcluster, "Error"=w730:bool, "Interface out"=w733:refnum<class "Interface.lvclass">)  [unwired: 7 in]
          n263 = call-dynamic "Read Exposições realizadas.vi"("error in (no error)"=w731, "Interface in"=w733) -> ("error out"=w761:errorcluster, "Exposições realizadas"=w762:dbl, "Interface out"=w763:refnum<class "Interface.lvclass">)  [unwired: 7 in]
          n264 = call-dynamic "Read Cam_Status.vi"("error in (no error)"=w761, "Interface in"=w763) -> ("error out"=w769:errorcluster, "Cam_Status"=w757:string, "Interface out"=w770:refnum<class "Interface.lvclass">)  [unwired: 7 in]
          n265 = call-dynamic "Read %Acquired.vi"("error in (no error)"=w769, "Interface in"=w770) -> ("error out"=w750:errorcluster, "% Acquired"=w766:dbl, "Interface out"=w751:refnum<class "Interface.lvclass">)  [unwired: 7 in]
          n266 = call-dynamic "Read Number of Cycles.vi"("error in (no error)"=w750, "Interface in"=w751) -> ("error out"=w747:errorcluster, "Number of Cycles"=w749:u32, "Interface out"=w748:refnum<class "Interface.lvclass">)  [unwired: 7 in]
          n267 = call-dynamic "Read Number of Sequences.vi"("error in (no error)"=w747, "Interface in"=w748) -> ("error out"=w737:errorcluster, "Number of Sequences"=w746:u32, "Interface out"=w739:refnum<class "Interface.lvclass">)  [unwired: 7 in]
          n268 = call-dynamic "Read Ocupacao do disco.vi"("error in (no error)"=w737, "Interface in"=w739) -> ("error out"=w736:errorcluster, "Ocupacao do disco"=w735:u16, "Interface out"=w738:refnum<class "Interface.lvclass">)  [unwired: 7 in]
          n269 = call "Read Exposure Time.vi"("error in (no error)"=w736, "Interface in"=w738) -> ("error out"=w759:errorcluster, "Exposure Time"=w768:dbl, "Interface out"=w758:refnum<class "Interface.lvclass">)  [unwired: 7 in]
          n270 = call-dynamic "Write Interface.vi"("error in (no error)"=w759, "Interface.lvclass"=w758, "Channel in"=w777) -> ("error out"=w772:errorcluster, "Channel out"=w771:refnum<class "Channel.lvclass">)  [unwired: 7 in]
          n271 = case shown="\"ACTIVE\"" w757 {
            tunnel: [w782 w785] -> w781
            tunnel: w780 -> [w784 w785]
            tunnel: w745 -> [_ _]
            frame "ACTIVE" {
              n272 = Increment(x=w784) -> (x+1=w783:i32)
              n273 = Increment(x=w783) -> (x+1=w782:i32)
            }
            frame Default {
              # "Não usa o timeout. Deixa o \nS4GUI:HandleObservationSync.vi  e ..Async.vi\ndetectarem o timeout no estado 53 ou incremento de CyclesDone."
            }
          }
          n274 = To Unsigned Long Integer(number=w762) -> (unsigned 32bit integer=w760:u32)
          n275 = Divide(x=w766, y=100.0) -> (x/y=w764:dbl)
          n276 = Multiply(x=w768, y=w764) -> (x*y=w767:dbl)
          n277 = Bundle By Name(cluster=w771, "Texp"=w767, "lastStatus"=w757, "Nimages"=w760, "CyclesDone"=w749, "SequesDone"=w746, "UsedDiskSpace"=w735, "Error"=w730) -> (w779:refnum<class "Channel.lvclass">)
        }
        frame 54 {
          # "OV 2024.11.04: Este estado não é mais utilizado."
          # "Verifica o timeout de 5s para enviar\ntelemetria para o ACS."
          n278 = call-dynamic "Verif Clock 2.vi"("error in (no error)"=w798, "period (ms)"=u32 5000 ("period"), "State Machine in"=w799) -> ("error out"=w796:errorcluster, "State Machine out"=w797:refnum<class "State Machine.lvclass">)  [unwired: 6 in, 1 out]
          n279 = call-dynamic "Read Timeout 2.vi"("error in (no error)"=w796, "State Machine in"=w797) -> ("error out"=w792:errorcluster, "Timeout 2"=w795:bool, "State Machine out"=w793:refnum<class "State Machine.lvclass">)  [unwired: 7 in]
          n280 = call-dynamic "Write State Machine.vi"("error in (no error)"=w792, "State Machine.lvclass"=w793, "Device in"=w794) -> ("error out"=w791:errorcluster, "Device out"=w790:refnum<class "Channel.lvclass">)  [unwired: 7 in]
          n281 = case shown="True" w795 {
            tunnel: [w815 w824] -> w789
            tunnel: [w814 w825] -> w788
            tunnel: [w813 w826] -> w802
            tunnel: w801 -> [w812 w823]
            tunnel: w790 -> [w811 w824]
            tunnel: w791 -> [w810 w825]
            frame False {
              n282 = disable-structure shown="Enabled" {
                disable-tunnel: [w820 w822] -> w815
                disable-tunnel: [w819 w821] -> w814
                disable-tunnel: w811 -> [w817 w822]
                disable-tunnel: w810 -> [w816 w821]
                frame Disabled {
                  n283 = call-dynamic "Write cmd.vi"("error in (no error)"=w816, "cmd"="STATUS", "Device in"=w817) -> ("error out"=w819:errorcluster, "Device out"=w820:refnum<class "Channel.lvclass">)  [unwired: 7 in]
                }
                frame Enabled {
                  # "2024_03_20: Nao pede mais STATUS,\npois ACS o publica a cada 1s."
                }
              }
              n284 = Increment(x=w812) -> (x+1=w813:i32)
            }
            frame True {
              n285 = disable-structure shown="Enabled" {
                disable-tunnel: [59 w828] -> w826
                disable-tunnel: w823 -> [_ w828]
                frame Disabled {
                  # "Estourou timeout de 5s:\nDesvia para enviar dados de \nTELEMETRIA a cada 5s (estado 59)"
                }
                frame Enabled {
                  # "2024-03020: Não evia mais dados\nda TELEMETRIA, pois ACS assina\nas publicacoes do S4GUI, TCS, etc."
                }
              }
            }
          }
          n286 = disable-structure shown="Disabled" {
            disable-tunnel: w789 -> [w806 w809]
            disable-tunnel: w788 -> [w805 w808]
            disable-tunnel: [w804 w809] -> w787
            disable-tunnel: [w803 w808] -> w786
            frame Disabled {
              n287 = call "Write connected.vi"("error in (no error)"=w805, "connected"=FALSE, "Device in"=w806) -> ("error out"=w803:errorcluster, "Device out"=w804:refnum<class "Channel.lvclass">)  [unwired: 7 in]
            }
            frame Enabled {
            }
          }
        }
        frame 55 {
          # "OV 2024.11.04: Não há mais Timeout neste estado.\nFica em 55 até ocorrer um Abort do usuário ou um status desconhecido."
          # "Status.Texp = Current frame exptime\nlastStatus = cam status (acquiring, idle, writing, reading, ...)\nStatus.Nimages = frames done\nStatus.CubesDone = ciclos realizados pelo ACS\nStatus.SequesDone = sequencias realizadas pelo ACS.\nStatus.UsedDiskSpace = espaco usado no disco.\nStatus.Error = Se TRUE, houve erro na aquisição do canal."
          # "Extrair todos os parametros da respsota de STATUS e\natualizar a informação na classe Channel."
          n288 = disable-structure shown="Enabled" {
            disable-tunnel: w842 -> [w884 w887]
            disable-tunnel: [w882 w887] -> w841
            disable-tunnel: w840 -> [w881 w886]
            disable-tunnel: [w879 FALSE ("Timeout")] -> _
            disable-tunnel: [w878 w886] -> w839
            frame Disabled {
              n289 = call-dynamic "Verif Clock.vi"("error in (no error)"=w881, "period (ms)"=u32 500 ("period"), "State Machine in"=w884) -> ("error out"=w880:errorcluster, "State Machine out"=w883:refnum<class "State Machine.lvclass">)  [unwired: 6 in, 1 out]
              n290 = call-dynamic "Read Timeout.vi"("error in (no error)"=w880, "State Machine in"=w883) -> ("error out"=w878:errorcluster, "Timeout"=w879:bool, "State Machine out"=w882:refnum<class "State Machine.lvclass">)  [unwired: 7 in]
            }
            frame Enabled {
            }
          }
          n291 = call-dynamic "Read resp.vi"("error in (no error)"=w839, "Device in"=w849) -> ("error out"=w869:errorcluster, "resp"=w870:string, "Device out"=w873:refnum<class "Channel.lvclass">)  [unwired: 7 in]
          n292 = call-dynamic "Read Interface.vi"("error in (no error)"=w869, "Channel in"=w873) -> ("error out"=w868:errorcluster, "Interface.lvclass"=w871:refnum<class "Interface.lvclass">, "Channel out"=w872:refnum<class "Channel.lvclass">)  [unwired: 7 in]
          n293 = call-dynamic "UpdateStatus.vi"("error in (no error)"=w868, "status"=w870, "Interface in"=w871) -> ("error out"=w831:errorcluster, "Interface out"=w833:refnum<class "Interface.lvclass">)  [unwired: 7 in]
          n294 = call-dynamic "Read Error.vi"("error in (no error)"=w831, "Interface in"=w833) -> ("error out"=w830:errorcluster, "Error"=w829:bool, "Interface out"=w832:refnum<class "Interface.lvclass">)  [unwired: 7 in]
          n295 = call-dynamic "Read Exposições realizadas.vi"("error in (no error)"=w830, "Interface in"=w832) -> ("error out"=w856:errorcluster, "Exposições realizadas"=w857:dbl, "Interface out"=w858:refnum<class "Interface.lvclass">)  [unwired: 7 in]
          n296 = call-dynamic "Read Cam_Status.vi"("error in (no error)"=w856, "Interface in"=w858) -> ("error out"=w865:errorcluster, "Cam_Status"=w854:string, "Interface out"=w867:refnum<class "Interface.lvclass">)  [unwired: 7 in]
          n297 = call-dynamic "Read %Acquired.vi"("error in (no error)"=w865, "Interface in"=w867) -> ("error out"=w864:errorcluster, "% Acquired"=w861:dbl, "Interface out"=w866:refnum<class "Interface.lvclass">)  [unwired: 7 in]
          n298 = call "Read Exposure Time.vi"("error in (no error)"=w864, "Interface in"=w866) -> ("error out"=w847:errorcluster, "Exposure Time"=w863:dbl, "Interface out"=w848:refnum<class "Interface.lvclass">)  [unwired: 7 in]
          n299 = call-dynamic "Read Number of Cycles.vi"("error in (no error)"=w847, "Interface in"=w848) -> ("error out"=w844:errorcluster, "Number of Cycles"=w846:u32, "Interface out"=w845:refnum<class "Interface.lvclass">)  [unwired: 7 in]
          n300 = call-dynamic "Read Number of Sequences.vi"("error in (no error)"=w844, "Interface in"=w845) -> ("error out"=w837:errorcluster, "Number of Sequences"=w843:u32, "Interface out"=w838:refnum<class "Interface.lvclass">)  [unwired: 7 in]
          n301 = call-dynamic "Read Ocupacao do disco.vi"("error in (no error)"=w837, "Interface in"=w838) -> ("error out"=w836:errorcluster, "Ocupacao do disco"=w834:u16, "Interface out"=w835:refnum<class "Interface.lvclass">)  [unwired: 7 in]
          n302 = call-dynamic "Write Interface.vi"("error in (no error)"=w836, "Interface.lvclass"=w835, "Channel in"=w872) -> ("error out"=w853:errorcluster, "Channel out"=w852:refnum<class "Channel.lvclass">)  [unwired: 7 in]
          n303 = case shown="\"ACQUISITION_ABORTED\", Default" w854 {
            tunnel: [0 ("State") w902] -> w876
            tunnel: w875 -> [_ w902]
            tunnel: w853 -> [w894 w898]
            tunnel: [w891 w900] -> w851
            tunnel: w852 -> [w892 w901]
            tunnel: [w888 w897] -> w850
            tunnel: w841 -> [w895 w899]
            frame "ACQUISITION_ABORTED", Default {
              # "OVJ 20230704"
              # "ABORTED ou STATUS desconhecido."
              # "250x20ms=5s"
              n304 = call-dynamic "Write Timer.vi"("error in (no error)"=w894, "Timer"=u32 250, "State Machine in"=w895) -> ("error out"=w889:errorcluster, "State Machine out"=w890:refnum<class "State Machine.lvclass">)  [unwired: 7 in]
              n305 = call-dynamic "Write State Machine.vi"("error in (no error)"=w889, "State Machine.lvclass"=w890, "Device in"=w892) -> ("error out"=w888:errorcluster, "Device out"=w891:refnum<class "Channel.lvclass">)  [unwired: 7 in]
            }
            frame "ACTIVE", "IDLE", "WAITING_EXPOSE_COMMAND" {
              # "STATUS DETECTOR = ACTIVE or WAITING EXPOSE COMMAND"
              n306 = call-dynamic "Write State Machine.vi"("error in (no error)"=w898, "State Machine.lvclass"=w899, "Device in"=w901) -> ("error out"=w897:errorcluster, "Device out"=w900:refnum<class "Channel.lvclass">)  [unwired: 7 in]
            }
          }
          n307 = To Unsigned Long Integer(number=w857) -> (unsigned 32bit integer=w855:u32)
          n308 = Divide(x=w861, y=100.0) -> (x/y=w859:dbl)
          n309 = Multiply(x=w863, y=w859) -> (x*y=w862:dbl)
          n310 = Bundle By Name(cluster=w851, "Texp"=w862, "lastStatus"=w854, "Nimages"=w855, "CyclesDone"=w846, "SequesDone"=w843, "UsedDiskSpace"=w834, "Error"=w829) -> (w874:refnum<class "Channel.lvclass">)
        }
        frame 56 {
          # "Pedido de STATUS para verificar conexão com ACS"
          # "Carrega timeout de 10 ciclos \n(20 x 20ms = 0.4s) \npara resposta do ACS"
          n311 = call-dynamic "Write Timer.vi"("error in (no error)"=w908, "Timer"=u32 20, "State Machine in"=w912) -> ("error out"=w913:errorcluster, "State Machine out"=w914:refnum<class "State Machine.lvclass">)  [unwired: 7 in]
          n312 = call-dynamic "Write State Machine.vi"("error in (no error)"=w913, "State Machine.lvclass"=w914, "Device in"=w910) -> ("error out"=w907:errorcluster, "Device out"=w909:refnum<class "Channel.lvclass">)  [unwired: 7 in]
          n313 = disable-structure shown="Enabled" {
            disable-tunnel: w909 -> [w927 w930]
            disable-tunnel: w907 -> [w926 w929]
            disable-tunnel: [w925 w930] -> w906
            disable-tunnel: [w924 w929] -> w905
            frame Disabled {
              n314 = call-dynamic "Write cmd.vi"("error in (no error)"=w926, "cmd"="STATUS", "Device in"=w927) -> ("error out"=w924:errorcluster, "Device out"=w925:refnum<class "Channel.lvclass">)  [unwired: 7 in]
            }
            frame Enabled {
              # "2024-03-20: Não envia mais pedido\nde STATUS, pois o ACS publica seu\nSTATUS a cada 1s."
            }
          }
          n315 = Increment(x=w915) -> (x+1=w916:i32)
          n316 = disable-structure shown="Disabled" {
            disable-tunnel: w906 -> [w921 w923]
            disable-tunnel: w905 -> [w920 w922]
            disable-tunnel: [w919 w923] -> w904
            disable-tunnel: [w918 w922] -> w903
            frame Disabled {
              # "2024.05.16\ncausa bug de\nfalsa queda na\ncomunicação \ncom ACS"
              n317 = call "Write connected.vi"("error in (no error)"=w920, "connected"=FALSE, "Device in"=w921) -> ("error out"=w918:errorcluster, "Device out"=w919:refnum<class "Channel.lvclass">)  [unwired: 7 in]
            }
            frame Enabled {
            }
          }
        }
        frame 57 {
          # "Status.Texp = Current frame exptime\nlastStatus = cam status (acquiring, idle, writing, reading, ...)\nStatus.Nimages = frames done\nStatus.CubesDone = ciclos realizados pelo ACS\nStatus.SequesDone = sequencias realizadas pelo ACS.\nStatus.UsedDiskSpace = espaco usado no disco.\nStatus.Error = Se TRUE, houve erro na aquisção do canal."
          # "Extrair todos os parametros da respsota de STATUS e\natualizar a informação na classe Channel."
          n318 = call "Verify Timer.vi"("error in (no error)"=w957, "State Machine in"=w956) -> ("error out"=w953:errorcluster, "State Machine out"=w955:refnum<class "State Machine.lvclass">)  [unwired: 7 in, 1 out]
          n319 = call-dynamic "Read Timeout.vi"("error in (no error)"=w953, "State Machine in"=w955) -> ("error out"=w948:errorcluster, "Timeout"=w952:bool, "State Machine out"=w954:refnum<class "State Machine.lvclass">)  [unwired: 7 in]
          n320 = call "Read connected.vi"("error in (no error)"=w948, "Device in"=w951) -> ("error out"=w949:errorcluster, "connected"=w947:bool, "Device out"=w950:refnum<class "Channel.lvclass">)  [unwired: 7 in]
          n321 = call-dynamic "Read resp.vi"("error in (no error)"=w949, "Device in"=w950) -> ("error out"=w977:errorcluster, "resp"=w978:string, "Device out"=w981:refnum<class "Channel.lvclass">)  [unwired: 7 in]
          n322 = call-dynamic "Read Interface.vi"("error in (no error)"=w977, "Channel in"=w981) -> ("error out"=w976:errorcluster, "Interface.lvclass"=w979:refnum<class "Interface.lvclass">, "Channel out"=w980:refnum<class "Channel.lvclass">)  [unwired: 7 in]
          n323 = call-dynamic "UpdateStatus.vi"("error in (no error)"=w976, "status"=w978, "Interface in"=w979) -> ("error out"=w933:errorcluster, "Interface out"=w935:refnum<class "Interface.lvclass">)  [unwired: 7 in]
          n324 = call-dynamic "Read Error.vi"("error in (no error)"=w933, "Interface in"=w935) -> ("error out"=w932:errorcluster, "Error"=w931:bool, "Interface out"=w934:refnum<class "Interface.lvclass">)  [unwired: 7 in]
          n325 = call-dynamic "Read Exposições realizadas.vi"("error in (no error)"=w932, "Interface in"=w934) -> ("error out"=w964:errorcluster, "Exposições realizadas"=w965:dbl, "Interface out"=w966:refnum<class "Interface.lvclass">)  [unwired: 7 in]
          n326 = call-dynamic "Read Cam_Status.vi"("error in (no error)"=w964, "Interface in"=w966) -> ("error out"=w973:errorcluster, "Cam_Status"=w962:string, "Interface out"=w975:refnum<class "Interface.lvclass">)  [unwired: 7 in]
          n327 = call-dynamic "Read %Acquired.vi"("error in (no error)"=w973, "Interface in"=w975) -> ("error out"=w972:errorcluster, "% Acquired"=w969:dbl, "Interface out"=w974:refnum<class "Interface.lvclass">)  [unwired: 7 in]
          n328 = call "Read Exposure Time.vi"("error in (no error)"=w972, "Interface in"=w974) -> ("error out"=w945:errorcluster, "Exposure Time"=w971:dbl, "Interface out"=w946:refnum<class "Interface.lvclass">)  [unwired: 7 in]
          n329 = call-dynamic "Read Number of Cycles.vi"("error in (no error)"=w945, "Interface in"=w946) -> ("error out"=w942:errorcluster, "Number of Cycles"=w944:u32, "Interface out"=w943:refnum<class "Interface.lvclass">)  [unwired: 7 in]
          n330 = call-dynamic "Read Number of Sequences.vi"("error in (no error)"=w942, "Interface in"=w943) -> ("error out"=w938:errorcluster, "Number of Sequences"=w941:u32, "Interface out"=w940:refnum<class "Interface.lvclass">)  [unwired: 7 in]
          n331 = call-dynamic "Read Ocupacao do disco.vi"("error in (no error)"=w938, "Interface in"=w940) -> ("error out"=w937:errorcluster, "Ocupacao do disco"=w936:u16, "Interface out"=w939:refnum<class "Interface.lvclass">)  [unwired: 7 in]
          n332 = call-dynamic "Write Interface.vi"("error in (no error)"=w937, "Interface.lvclass"=w939, "Channel in"=w980) -> ("error out"=w961:errorcluster, "Channel out"=w960:refnum<class "Channel.lvclass">)  [unwired: 7 in]
          n333 = case shown="False" w947 {
            tunnel: [w987 w1004] -> w984
            tunnel: w983 -> [w988 w1005]
            tunnel: w961 -> [w985 w1002]
            tunnel: [w990 w999] -> w959
            tunnel: w960 -> [w991 w1003]
            tunnel: [w989 w996] -> w958
            tunnel: w954 -> [w986 w1001]
            tunnel: w952 -> [_ w995]
            frame True {
              # "Conneted=T\nACS respondeu"
              n334 = disable-structure shown="Enabled" {
                disable-tunnel: w988 -> [w993 _]
                disable-tunnel: [w992 0] -> w987
                frame Disabled {
                  n335 = Increment(x=w993) -> (x+1=w992:i32)
                }
                frame Enabled {
                }
              }
              n336 = call-dynamic "Write State Machine.vi"("error in (no error)"=w985, "State Machine.lvclass"=w986, "Device in"=w991) -> ("error out"=w989:errorcluster, "Device out"=w990:refnum<class "Channel.lvclass">)  [unwired: 7 in]
            }
            frame False {
              # "Conneted=F\nACS não resp."
              n337 = case shown="False" w995 {
                tunnel: w1005 -> [w1006 _]
                tunnel: [w1006 0] -> w1004
                tunnel: w1003 -> [w1009 w1012]
                tunnel: [w1009 w1012] -> w1000
                tunnel: w1002 -> [w1008 w1013]
                tunnel: [w1008 w1010] -> w997
                tunnel: w1001 -> [w1007 w1015]
                tunnel: [w1007 w1011] -> w998
                frame False {
                }
                frame True {
                  n338 = call-dynamic "Write Timer.vi"("error in (no error)"=w1013, "Timer"=u32 250, "State Machine in"=w1015) -> ("error out"=w1010:errorcluster, "State Machine out"=w1011:refnum<class "State Machine.lvclass">)  [unwired: 7 in]
                }
              }
              n339 = call-dynamic "Write State Machine.vi"("error in (no error)"=w997, "State Machine.lvclass"=w998, "Device in"=w1000) -> ("error out"=w996:errorcluster, "Device out"=w999:refnum<class "Channel.lvclass">)  [unwired: 7 in]
            }
          }
          n340 = Divide(x=w969, y=100.0) -> (x/y=w967:dbl)
          n341 = To Unsigned Long Integer(number=w965) -> (unsigned 32bit integer=w963:u32)
          n342 = Multiply(x=w971, y=w967) -> (x*y=w970:dbl)
          n343 = Bundle By Name(cluster=w959, "Texp"=w970, "lastStatus"=w962, "Nimages"=w963, "CyclesDone"=w944, "SequesDone"=w941, "UsedDiskSpace"=w936, "Error"=w931) -> (w982:refnum<class "Channel.lvclass">)
        }
        frame 58 {
          w1021 = "}" ("regular expression")
          # "Passa valores da telemetria adquiridos do TCS"
          n344 = call-dynamic "Write State Machine.vi"("error in (no error)"=w1017, "State Machine.lvclass"=w1018, "Device in"=w1028) -> ("error out"=w1025:errorcluster, "Device out"=w1027:refnum<class "Channel.lvclass">)  [unwired: 7 in]
          n345 = Unbundle By Name(w1027) -> ("TCS telemetry"=w1022:string, "Filter"=w1024:u8)
          n346 = Match Pattern(string=w1022, regular expression=w1021) -> (before substring=w1020:string, match substring=w1019:string)  [unwired: 1 in, 2 out]
          n347 = Equal?(x=w1019, y=w1021) -> (x = y?=w1023:bool)
          n348 = case shown="True" w1023 {
            tunnel: [w1032 w1042] -> w1030
            tunnel: [w1031 w1041] -> w1029
            tunnel: w1027 -> [w1032 w1040]
            tunnel: w1025 -> [w1031 w1037]
            tunnel: w1024 -> [_ w1036]
            tunnel: w1020 -> [_ w1035]
            tunnel: w1019 -> [_ w1034]
            frame False {
            }
            frame True {
              (unwired) "\"CTRLINTE\":\"S4GUI\"}" ("string")
              (unwired) "\"FILTER\":\"" ("string")
              n349 = case shown="5" w1036 {
                tunnel: ["CLEAR\"," ("string") "U\"," ("string") "B\"," ("string") "V\"," ("string") "R\"," ("string") "S\"," ("string")] -> _
                frame 0, Default {
                }
                frame 1 {
                }
                frame 2 {
                }
                frame 3 {
                }
                frame 4 {
                }
                frame 5 {
                }
              }
              n350 = Concatenate Strings(w1035, w1034) -> (w1033:string)
              n351 = Concatenate Strings("WRITE_HEADER_DATA " ("cmd"), w1033) -> (w1038:string)
              n352 = disable-structure shown="Enabled" {
                disable-tunnel: [w1047 w1049] -> w1042
                disable-tunnel: [w1046 w1048] -> w1041
                disable-tunnel: w1040 -> [w1045 w1049]
                disable-tunnel: w1038 -> [w1044 _]
                disable-tunnel: w1037 -> [w1043 w1048]
                frame Disabled {
                  n353 = call-dynamic "Write cmd.vi"("error in (no error)"=w1043, "cmd"=w1044, "Device in"=w1045) -> ("error out"=w1046:errorcluster, "Device out"=w1047:refnum<class "Channel.lvclass">)  [unwired: 7 in]
                }
                frame Enabled {
                  # "Não existe mais\neste comando."
                }
              }
            }
          }
        }
        frame 59 {
          w1060 = "}" ("regular expression")
          # "Passa valores da telemetria adquiridos do TCS durante a aquisição do canal (estados 54 e 55)"
          n354 = call-dynamic "Write State Machine.vi"("error in (no error)"=w1056, "State Machine.lvclass"=w1057, "Device in"=w1066) -> ("error out"=w1063:errorcluster, "Device out"=w1065:refnum<class "Channel.lvclass">)  [unwired: 7 in]
          n355 = Unbundle By Name(w1065) -> ("TCS telemetry"=w1061:string)
          n356 = Match Pattern(string=w1061, regular expression=w1060) -> (before substring=w1059:string, match substring=w1058:string)  [unwired: 1 in, 2 out]
          n357 = Equal?(x=w1058, y=w1060) -> (x = y?=w1062:bool)
          n358 = case shown="True" w1062 {
            tunnel: [w1070 w1079] -> w1068
            tunnel: [w1069 w1078] -> w1067
            tunnel: w1065 -> [w1070 w1077]
            tunnel: w1063 -> [w1069 w1074]
            tunnel: w1059 -> [_ w1073]
            tunnel: w1058 -> [_ w1072]
            frame False {
            }
            frame True {
              n359 = Concatenate Strings(w1073, w1072) -> (w1071:string)
              n360 = Concatenate Strings("WRITE_HEADER_DATA " ("cmd"), w1071) -> (w1075:string)
              n361 = disable-structure shown="Enabled" {
                disable-tunnel: [w1084 w1086] -> w1079
                disable-tunnel: [w1083 w1085] -> w1078
                disable-tunnel: w1077 -> [w1082 w1086]
                disable-tunnel: w1075 -> [w1081 _]
                disable-tunnel: w1074 -> [w1080 w1085]
                frame Disabled {
                  n362 = call-dynamic "Write cmd.vi"("error in (no error)"=w1080, "cmd"=w1081, "Device in"=w1082) -> ("error out"=w1083:errorcluster, "Device out"=w1084:refnum<class "Channel.lvclass">)  [unwired: 7 in]
                }
                frame Enabled {
                  # "Não existe mais\neste comando."
                }
              }
            }
          }
        }
        frame 60 {
          # "Carrega timeout de 5 ciclos\npara resposta do ACS"
          n363 = call-dynamic "Write Timer.vi"("Timer"=u32 5, "State Machine in"=w1094) -> ("error out"=w1095:errorcluster, "State Machine out"=w1093:refnum<class "State Machine.lvclass">)  [unwired: 8 in]
          n364 = call-dynamic "Write State Machine.vi"("error in (no error)"=w1095, "State Machine.lvclass"=w1093, "Device in"=w1092) -> ("Device out"=w1089:refnum<class "Channel.lvclass">)  [unwired: 7 in, 1 out]
          n365 = Bundle By Name(cluster=w1089, "config"=TRUE) -> (w1088:refnum<class "Channel.lvclass">)
          n366 = disable-structure shown="Enabled" {
            disable-tunnel: [w1106 w1108] -> w1099
            disable-tunnel: w1098 -> [w1105 w1107]
            disable-tunnel: [w1104 w1107] -> w1097
            disable-tunnel: w1088 -> [w1102 w1108]
            disable-tunnel: w1091 -> [w1101 _]
            disable-tunnel: [w1100 62] -> w1090
            frame Disabled {
              n367 = Increment(x=w1101) -> (x+1=w1100:i32)
              n368 = call-dynamic "Write cmd.vi"("error in (no error)"=w1105, "cmd"="INIT", "Device in"=w1102) -> ("error out"=w1104:errorcluster, "Device out"=w1106:refnum<class "Channel.lvclass">)  [unwired: 7 in]
            }
            frame Enabled {
            }
          }
        }
        frame 61 {
          w1119 = "INITIALIZATION"
          # "Verifica timeout para ACS responder.\nSe estourar timeout é porque o ACS não \nrespondeu e este canal volta para o estado 0\npara não \"travar\" os outros canais no \nS4ACS_GUI:HandleObservation.vi."
          n369 = call "Verify Timer.vi"("error in (no error)"=w1110, "State Machine in"=w1115) -> ("error out"=w1116:errorcluster, "timeout"=w1111:bool, "State Machine out"=w1117:refnum<class "State Machine.lvclass">)  [unwired: 7 in]
          n370 = call-dynamic "Write State Machine.vi"("error in (no error)"=w1116, "State Machine.lvclass"=w1117, "Device in"=w1114) -> ("error out"=w1112:errorcluster, "Device out"=w1113:refnum<class "Channel.lvclass">)  [unwired: 7 in]
          n371 = call-dynamic "Read resp.vi"("error in (no error)"=w1112, "Device in"=w1113) -> ("error out"=w1123:errorcluster, "resp"=w1121:string, "Device out"=w1124:refnum<class "Channel.lvclass">)  [unwired: 7 in]
          "resp INIT" <- w1121
          n372 = Match Pattern(string=w1121, regular expression=w1119) -> (match substring=w1120:string)  [unwired: 1 in, 3 out]
          n373 = Equal?(x=w1120, y=w1119) -> (x = y?=w1118:bool)
          n374 = case shown="True" w1118 {
            tunnel: [w1126 w1131] -> w1125
            tunnel: w1122 -> [w1127 w1132]
            tunnel: w1111 -> [w1128 _]
            frame False {
              n375 = case shown="False" w1128 {
                tunnel: [w1129 0 ("State")] -> w1126
                tunnel: w1127 -> [w1129 _]
                frame False {
                }
                frame True {
                }
              }
            }
            frame True {
              n376 = disable-structure shown="Enabled" {
                disable-tunnel: w1132 -> [w1134 _]
                disable-tunnel: [w1133 54] -> w1131
                frame Disabled {
                  n377 = Increment(x=w1134) -> (x+1=w1133:i32)
                }
                frame Enabled {
                  # "debug:\nNão deve enviar\n WRITE_SETUP para o \nACS antigo"
                }
              }
            }
          }
        }
        frame 62 {
          # "Aguarda para reconfigurar.\n(o timer deve ser recarregado \nquando SM:NextState.vi recebe 62).\n\nIsso foi inserido para dar tempo\ndas VIs de ZMQ estarem prontas\npara enviar e receber mensagens \ndos ACS após o S4GUI:Initialize.vi."
          n378 = call "Verify Timer.vi"("error in (no error)"=w1139, "State Machine in"=w1140) -> ("error out"=w1136:errorcluster, "timeout"=w1141:bool, "State Machine out"=w1138:refnum<class "State Machine.lvclass">)  [unwired: 7 in]
          n379 = case shown="True" w1141 {
            tunnel: [w1149 w1172] -> w1145
            tunnel: [w1150 w1171] -> w1144
            tunnel: w1143 -> [w1151 w1169]
            tunnel: [w1151 w1163] -> w1142
            tunnel: w1136 -> [w1146 w1154]
            tunnel: w1138 -> [w1148 w1156]
            tunnel: w1137 -> [w1147 w1158]
            frame False {
              n380 = call-dynamic "Write State Machine.vi"("error in (no error)"=w1146, "State Machine.lvclass"=w1148, "Device in"=w1147) -> ("error out"=w1150:errorcluster, "Device out"=w1149:refnum<class "Channel.lvclass">)  [unwired: 7 in]
            }
            frame True {
              # "Salta para estado 65\npara tratar a próxima\npublicação de STATUS\n do ACS."
              n381 = call-dynamic "Write Timer.vi"("error in (no error)"=w1154, "Timer"=u32 50, "State Machine in"=w1156) -> ("error out"=w1153:errorcluster, "State Machine out"=w1155:refnum<class "State Machine.lvclass">)  [unwired: 7 in]
              n382 = call-dynamic "Write State Machine.vi"("error in (no error)"=w1153, "State Machine.lvclass"=w1155, "Device in"=w1158) -> ("error out"=w1152:errorcluster, "Device out"=w1157:refnum<class "Channel.lvclass">)  [unwired: 7 in]
              n383 = call-dynamic "Read target cluster.vi"("error in (no error)"=w1152, "Channel in"=w1157) -> ("error out"=w1161:errorcluster, "target cluster"=w1162:T3, "Channel out"=w1160:refnum<class "Channel.lvclass">)  [unwired: 7 in]
              n384 = Increment(x=w1169) -> (x+1=w1170:i32)
              n385 = Flatten To JSON(anything=w1162, error in (no error)=w1161) -> (JSON string=w1166:string, 11:w1165:errorcluster)  [unwired: 1 in]
              n386 = Increment(x=w1170) -> (x+1=w1164:i32)
              n387 = Increment(x=w1164) -> (x+1=w1163:i32)
              n388 = Concatenate Strings("WRITE_SETUP " ("cmd"), w1166) -> (w1167:string)
              n389 = call-dynamic "Write cmd.vi"("error in (no error)"=w1165, "cmd"=w1167, "Device in"=w1160) -> ("error out"=w1171:errorcluster, "Device out"=w1172:refnum<class "Channel.lvclass">)  [unwired: 7 in]
            }
          }
        }
        frame 63 {
          # "Não há resposta para o comando WRTITE_SETUP\nQuando estourar timeout vai para o estado 64 para \nobter o STATUS do ACS."
          n390 = call "Verify Timer.vi"("error in (no error)"=w1176, "State Machine in"=w1178) -> ("error out"=w1179:errorcluster, "timeout"=w1175:bool, "State Machine out"=w1180:refnum<class "State Machine.lvclass">)  [unwired: 7 in]
          n391 = call-dynamic "Write State Machine.vi"("error in (no error)"=w1179, "State Machine.lvclass"=w1180, "Device in"=w1177) -> ("error out"=w1173:errorcluster, "Device out"=w1174:refnum<class "Channel.lvclass">)  [unwired: 7 in]
          n392 = case shown="True" w1175 {
            tunnel: [w1183 w1184] -> w1182
            tunnel: w1181 -> [w1183 w1185]
            frame False {
            }
            frame True {
              n393 = Increment(x=w1185) -> (x+1=w1184:i32)
            }
          }
        }
        frame 64 {
          # "Carrega timeout de 50 ciclos\npara resposta do ACS"
          n394 = call-dynamic "Write Timer.vi"("error in (no error)"=w1188, "Timer"=u32 50, "State Machine in"=w1191) -> ("error out"=w1192:errorcluster, "State Machine out"=w1190:refnum<class "State Machine.lvclass">)  [unwired: 7 in]
          n395 = call-dynamic "Write State Machine.vi"("error in (no error)"=w1192, "State Machine.lvclass"=w1190, "Device in"=w1189) -> ("error out"=w1186:errorcluster, "Device out"=w1187:refnum<class "Channel.lvclass">)  [unwired: 7 in]
          n396 = disable-structure shown="Enabled" {
            disable-tunnel: [w1202 w1204] -> w1197
            disable-tunnel: [w1201 w1203] -> w1196
            disable-tunnel: w1187 -> [w1200 w1204]
            disable-tunnel: w1186 -> [w1198 w1203]
            frame Disabled {
              n397 = call-dynamic "Write cmd.vi"("error in (no error)"=w1198, "cmd"="READ_SETUP ", "Device in"=w1200) -> ("error out"=w1201:errorcluster, "Device out"=w1202:refnum<class "Channel.lvclass">)  [unwired: 7 in]
            }
            frame Enabled {
            }
          }
          n398 = Increment(x=w1194) -> (x+1=w1195:i32)
        }
        frame 65 {
          n399 = call "Verify Timer.vi"("error in (no error)"=w1224, "State Machine in"=w1226) -> ("error out"=w1227:errorcluster, "timeout"=w1213:bool, "State Machine out"=w1228:refnum<class "State Machine.lvclass">)  [unwired: 7 in]
          n400 = call-dynamic "Write State Machine.vi"("error in (no error)"=w1227, "State Machine.lvclass"=w1228, "Device in"=w1225) -> ("error out"=w1222:errorcluster, "Device out"=w1223:refnum<class "Channel.lvclass">)  [unwired: 7 in]
          n401 = call-dynamic "Read resp.vi"("error in (no error)"=w1222, "Device in"=w1223) -> ("error out"=w1218:errorcluster, "resp"=w1208:string, "Device out"=w1205:refnum<class "Channel.lvclass">)  [unwired: 7 in]
          n402 = disable-structure shown="Enabled" {
            disable-tunnel: w1205 -> [w1229 w1244]
            disable-tunnel: [w1236 w1239] -> w1220
            disable-tunnel: [w1235 w1241] -> w1219
            disable-tunnel: w1218 -> [w1233 w1242]
            disable-tunnel: [w1232 w1238] -> w1217
            disable-tunnel: w1208 -> [w1231 w1243]
            disable-tunnel: [w1230 w1237] -> w1207
            disable-tunnel: [w1229 w1240] -> w1206
            frame Disabled {
              n403 = Unbundle By Name(w1229) -> ("Interface.lvclass"=w1234:refnum<class "Interface.lvclass">)
              n404 = call-dynamic "UpdateCCDconf.vi"("error in (no error)"=w1233, "status"=w1231, "Interface in"=w1234) -> ("error out"=w1235:errorcluster, "CCD conf rx"=w1232:T3, "Cluster comparison"=w1230:T1, "Interface out"=w1236:refnum<class "Interface.lvclass">)  [unwired: 5 in]
            }
            frame Enabled {
              n405 = call-dynamic "Check CCD Config.vi"("error in (no error)"=w1242, "Status"=w1243, "Channel in"=w1244) -> ("error out"=w1241:errorcluster, "cluster RX"=w1238:T3, "Cluster COMPARE"=w1237:T1, "Channel out"=w1240:refnum<class "Channel.lvclass">)  [unwired: 5 in]
              n406 = Unbundle By Name(w1240) -> ("Interface.lvclass"=w1239:refnum<class "Interface.lvclass">)
            }
          }
          n407 = case shown="True" w1213 {
            tunnel: w1220 -> [w1247 w1262]
            tunnel: w1219 -> [w1246 w1261]
            tunnel: w1217 -> [_ w1257]
            tunnel: [w1247 w1260] -> w1215
            tunnel: [w1246 w1259] -> w1216
            tunnel: [w1248 w1256] -> w1214
            tunnel: w1210 -> [w1245 w1258]
            tunnel: [w1245 w1253] -> w1209
            tunnel: w1207 -> [_ w1256]
            frame False {
              n408 = disable-structure shown="Enabled" {
                disable-tunnel: [T1 {"ACQUISITION_MODE"=FALSE, "TRIGGER_MODE"=FALSE, "READ_MODE"=FALSE, "PREAMP"=FALSE, "READOUT_RATE"=FALSE, "VERTICAL_SHIFT_SPEED"=FALSE, "EM_MODE"=FALSE, "EM_GAIN"=FALSE, "SHUTTER_MODE"=FALSE, "SHUTTER_TTL"=FALSE, "SHUTTER_OPENING_TIME"=FALSE, "SHUTTER_CLOSING_TIME"=FALSE, "VBIN"=FALSE, "HBIN"=FALSE, "INITIAL_LINE"=FALSE, "INITIAL_COLUMN"=FALSE, "FINAL_LINE"=FALSE, "FINAL_COLUMN"=FALSE, "FRAME_TRANSFER"=FALSE, "VERTICAL_CLOCK_VOLTAGE"=FALSE, "AD_CHANNEL"=FALSE} ("x = y?") T1 {"ACQUISITION_MODE"=TRUE, "TRIGGER_MODE"=TRUE, "READ_MODE"=TRUE, "PREAMP"=TRUE, "READOUT_RATE"=TRUE, "VERTICAL_SHIFT_SPEED"=TRUE, "EM_MODE"=TRUE, "EM_GAIN"=TRUE, "SHUTTER_MODE"=TRUE, "SHUTTER_TTL"=TRUE, "SHUTTER_OPENING_TIME"=TRUE, "SHUTTER_CLOSING_TIME"=TRUE, "VBIN"=TRUE, "HBIN"=TRUE, "INITIAL_LINE"=TRUE, "INITIAL_COLUMN"=TRUE, "FINAL_LINE"=TRUE, "FINAL_COLUMN"=TRUE, "FRAME_TRANSFER"=TRUE, "VERTICAL_CLOCK_VOLTAGE"=TRUE, "AD_CHANNEL"=TRUE} ("x = y?")] -> w1248
                frame Disabled {
                }
                frame Enabled {
                }
              }
            }
            frame True {
              n409 = disable-structure shown="Enabled" {
                disable-tunnel: w1258 -> [w1264 _]
                disable-tunnel: [w1263 0] -> w1251
                frame Disabled {
                  n410 = Increment(x=w1264) -> (x+1=w1263:i32)
                }
                frame Enabled {
                }
              }
              n411 = Not Equal?(x=T1 {"ACQUISITION_MODE"=TRUE, "TRIGGER_MODE"=TRUE, "READ_MODE"=TRUE, "PREAMP"=TRUE, "READOUT_RATE"=TRUE, "VERTICAL_SHIFT_SPEED"=TRUE, "EM_MODE"=TRUE, "EM_GAIN"=TRUE, "SHUTTER_MODE"=TRUE, "SHUTTER_TTL"=TRUE, "SHUTTER_OPENING_TIME"=TRUE, "SHUTTER_CLOSING_TIME"=TRUE, "VBIN"=TRUE, "HBIN"=TRUE, "INITIAL_LINE"=TRUE, "INITIAL_COLUMN"=TRUE, "FINAL_LINE"=TRUE, "FINAL_COLUMN"=TRUE, "FRAME_TRANSFER"=TRUE, "VERTICAL_CLOCK_VOLTAGE"=TRUE, "AD_CHANNEL"=TRUE}, y=w1256) -> (x != y?=w1254:bool)
              n412 = call-dynamic "Set CCD_Config.vi"("error in (no error)"=w1261, "input cluster"=w1257, "Interface in"=w1262) -> ("error out"=w1259:errorcluster, "Interface out"=w1260:refnum<class "Interface.lvclass">)  [unwired: 7 in]
              n413 = Select(t=27 ("f"), s=w1254, f=w1251) -> (s? t:f=w1253:i32)
            }
          }
          "x = y?" <- w1214
          n414 = call "Write Checked Params.vi"("error in (no error)"=w1216, "Checked Params"=w1214, "Interface in"=w1215) -> ("error out"=w1211:errorcluster, "Interface out"=w1212:refnum<class "Interface.lvclass">)  [unwired: 7 in]
          n415 = Bundle By Name(cluster=w1206, "Interface.lvclass"=w1212) -> (w1221:refnum<class "Channel.lvclass">)
        }
        frame 66 {
          # "O valor do COOLER aqui\nfoi carregado no Acquistion:Init.vi"
          # "Se COOLER=0\n        SET COLLERPOWER_STATUS 0\n        AVANÇA ESTADO\n        VAI PRA 0\nSe COOLER=1:\n      DESVIA PARA Estado 35"
          # "Carrega timeout de 50 ciclos\npara resposta do ACS"
          n416 = call-dynamic "Write Timer.vi"("error in (no error)"=w1273, "Timer"=u32 50, "State Machine in"=w1274) -> ("error out"=w1271:errorcluster, "State Machine out"=w1270:refnum<class "State Machine.lvclass">)  [unwired: 7 in]
          n417 = call-dynamic "Write State Machine.vi"("error in (no error)"=w1271, "State Machine.lvclass"=w1270, "Device in"=w1272) -> ("error out"=w1269:errorcluster, "Device out"=w1268:refnum<class "Channel.lvclass">)  [unwired: 7 in]
          n418 = Unbundle By Name(w1268) -> ("Interface.lvclass"=w1267:refnum<class "Interface.lvclass">)
          n419 = call-dynamic "Read Cooler ON_OFF.vi"("Interface in"=w1267) -> ("Cooler ON/OFF"=w1266:i16)  [unwired: 8 in, 2 out]
          n420 = case shown="0, Default" w1266 {
            tunnel: [w1282 w1289] -> w1279
            tunnel: [w1281 w1288] -> w1278
            tunnel: [35 w1287] -> w1277
            tunnel: w1276 -> [_ w1286]
            tunnel: w1269 -> [w1281 w1284]
            tunnel: w1268 -> [w1282 w1283]
            frame 1 {
              # "Se COOLER foi carregado com 1 na inicialização.\ndesvia para 35 para setar a temperatura e ligar o COOLER."
            }
            frame 0, Default {
              n421 = Increment(x=w1286) -> (x+1=w1287:i32)
              n422 = call-dynamic "Write cmd.vi"("error in (no error)"=w1284, "cmd"="SET COOLER_POWER_STATUS 0", "Device in"=w1283) -> ("error out"=w1288:errorcluster, "Device out"=w1289:refnum<class "Channel.lvclass">)  [unwired: 7 in]
            }
          }
        }
        frame 67 {
          # "Compara o parametro enviado com\no parametro no Acquisition Configuration\nda msg de STATUS do ACS."
          n423 = call "Verify Timer.vi"("error in (no error)"=w1305, "State Machine in"=w1309) -> ("error out"=w1304:errorcluster, "timeout"=w1302:bool, "State Machine out"=w1306:refnum<class "State Machine.lvclass">)  [unwired: 7 in]
          n424 = call-dynamic "Write State Machine.vi"("error in (no error)"=w1304, "State Machine.lvclass"=w1306, "Device in"=w1308) -> ("error out"=w1303:errorcluster, "Device out"=w1307:refnum<class "Channel.lvclass">)  [unwired: 7 in]
          n425 = call-dynamic "Read resp.vi"("error in (no error)"=w1303, "Device in"=w1307) -> ("error out"=w1294:errorcluster, "resp"=w1295:string, "Device out"=w1290:refnum<class "Channel.lvclass">)  [unwired: 7 in]
          n426 = Unbundle By Name(w1290) -> ("Interface.lvclass"=w1301:refnum<class "Interface.lvclass">)
          n427 = call-dynamic "UpdateACQconf.vi"("error in (no error)"=w1294, "status"=w1295, "Interface in"=w1301) -> ("error out"=w1296:errorcluster, "ACQ conf rx"=w1299:T2, "Interface out"=w1300:refnum<class "Interface.lvclass">)  [unwired: 6 in]
          n428 = Unbundle By Name(w1299) -> ("COOLER_POWER_STATUS"=w1297:dbl)
          n429 = call-dynamic "Read Cooler ON_OFF.vi"("error in (no error)"=w1296, "Interface in"=w1300) -> ("error out"=w1292:errorcluster, "Cooler ON/OFF"=w1298:i16)  [unwired: 7 in, 1 out]
          n430 = To Word Integer(number=w1297) -> (16bit integer=w1291:i16)
          n431 = Equal?(x=w1298, y=w1291) -> (x = y?=w1293:bool)
          n432 = case shown="True" w1293 {
            tunnel: [w1312 w1317] -> w1311
            tunnel: w1310 -> [w1313 _]
            tunnel: w1302 -> [w1314 _]
            frame False {
              n433 = case shown="True" w1314 {
                tunnel: [w1315 300 ("State")] -> w1312
                tunnel: w1313 -> [w1315 _]
                frame False {
                }
                frame True {
                  (unwired) 40 ("State")
                  # "2024.07.01:\nConfigura\nsuffix e  \nExp mode."
                }
              }
            }
            frame True {
              n434 = disable-structure shown="Enabled" {
                disable-tunnel: [54 ("State") 300 ("State")] -> w1317
                frame Disabled {
                }
                frame Enabled {
                  # "Fim. Vai para 300\nsetar Suffix e\nhabilitar WAIT_\nEXPOSE_COMMAND"
                }
              }
            }
          }
        }
        frame 70 {
          w1323 = "" ("resp")
          # "Carrega timeout de 5 ciclos\npara resposta do ACS"
          n435 = call-dynamic "Write Timer.vi"("error in (no error)"=w1336, "Timer"=u32 5, "State Machine in"=w1338) -> ("error out"=w1340:errorcluster, "State Machine out"=w1339:refnum<class "State Machine.lvclass">)  [unwired: 7 in]
          n436 = call-dynamic "Write State Machine.vi"("error in (no error)"=w1340, "State Machine.lvclass"=w1339, "Device in"=w1337) -> ("error out"=w1335:errorcluster, "Device out"=w1322:refnum<class "Channel.lvclass">)  [unwired: 7 in]
          n437 = Bundle By Name(cluster=w1322, "stopping"=TRUE) -> (w1320:refnum<class "Channel.lvclass">)
          n438 = call-dynamic "Write cmd.vi"("error in (no error)"=w1335, "cmd"="STOP_ACQUISITION", "Device in"=w1320) -> ("error out"=w1333:errorcluster, "Device out"=w1334:refnum<class "Channel.lvclass">)  [unwired: 7 in]
          n439 = call-dynamic "Write resp.vi"("error in (no error)"=w1333, "resp"=w1323, "Device in"=w1334) -> ("error out"=w1329:errorcluster, "Device out"=w1332:refnum<class "Channel.lvclass">)  [unwired: 7 in]
          n440 = call-dynamic "Read Interface.vi"("error in (no error)"=w1329, "Channel in"=w1332) -> ("error out"=w1328:errorcluster, "Interface.lvclass"=w1327:refnum<class "Interface.lvclass">, "Channel out"=w1331:refnum<class "Channel.lvclass">)  [unwired: 7 in]
          n441 = call-dynamic "UpdateStatus.vi"("error in (no error)"=w1328, "status"=w1323, "Interface in"=w1327) -> ("error out"=w1325:errorcluster, "Interface out"=w1326:refnum<class "Interface.lvclass">)  [unwired: 7 in]
          n442 = call-dynamic "Write Interface.vi"("error in (no error)"=w1325, "Interface.lvclass"=w1326, "Channel in"=w1331) -> ("error out"=w1324:errorcluster, "Channel out"=w1330:refnum<class "Channel.lvclass">)  [unwired: 7 in]
          n443 = Increment(x=w1343) -> (x+1=w1344:i32)
        }
        frame 71 {
          w1346 = "DONE"
          n444 = call-dynamic "Read resp.vi"("error in (no error)"=w1353, "Device in"=w1354) -> ("error out"=w1350:errorcluster, "resp"=w1348:string, "Device out"=w1351:refnum<class "Channel.lvclass">)  [unwired: 7 in]
          "resp STOP" <- w1348
          n445 = Match Pattern(string=w1348, regular expression=w1346) -> (match substring=w1347:string)  [unwired: 1 in, 3 out]
          n446 = Equal?(x=w1347, y=w1346) -> ()  [unwired: 1 out]
          n447 = case shown="True" TRUE {
            tunnel: [w1355 0 ("State")] -> w1352
            tunnel: w1349 -> [w1355 _]
            frame False {
            }
            frame True {
            }
          }
        }
        frame 80 {
          n448 = call-dynamic "Write cmd.vi"("error in (no error)"=w1366, "cmd"="ABORT_ACQUISITION", "Device in"=w1365) -> ("error out"=w1360:errorcluster, "Device out"=w1361:refnum<class "Channel.lvclass">)  [unwired: 7 in]
          n449 = call-dynamic "Write resp.vi"("error in (no error)"=w1360, "resp"="", "Device in"=w1361) -> ("error out"=w1359:errorcluster, "Device out"=w1358:refnum<class "Channel.lvclass">)  [unwired: 7 in]
          n450 = Increment(x=w1363) -> (x+1=w1364:i32)
        }
        frame 81 {
          w1368 = "DONE"
          n451 = call-dynamic "Read resp.vi"("error in (no error)"=w1375, "Device in"=w1376) -> ("error out"=w1372:errorcluster, "resp"=w1370:string, "Device out"=w1373:refnum<class "Channel.lvclass">)  [unwired: 7 in]
          "resp ABORT" <- w1370
          n452 = Match Pattern(string=w1370, regular expression=w1368) -> (match substring=w1369:string)  [unwired: 1 in, 3 out]
          n453 = Equal?(x=w1369, y=w1368) -> ()  [unwired: 1 out]
          n454 = case shown="True" TRUE {
            tunnel: [w1377 0 ("State")] -> w1374
            tunnel: w1371 -> [w1377 _]
            frame False {
            }
            frame True {
            }
          }
        }
        frame 90 {
          n455 = Unbundle By Name(w1380) -> ("wait_expose"=w1379:bool)
          n456 = case shown="False" w1379 {
            tunnel: w1388 -> [w1393 w1394]
            tunnel: w1380 -> [w1392 w1395]
            tunnel: [w1391 w1395] -> w1385
            tunnel: [w1390 w1394] -> w1384
            frame False {
              # "20240710: Se o ACS não estiver\nesperando EXPOSE, manda pausar a\naquisição."
              n457 = call-dynamic "Write cmd.vi"("error in (no error)"=w1393, "cmd"="PAUSE_ACQUISITION", "Device in"=w1392) -> ("error out"=w1390:errorcluster, "Device out"=w1391:refnum<class "Channel.lvclass">)  [unwired: 7 in]
            }
            frame True {
            }
          }
          n458 = call-dynamic "Write resp.vi"("error in (no error)"=w1384, "resp"="", "Device in"=w1385) -> ("error out"=w1383:errorcluster, "Device out"=w1382:refnum<class "Channel.lvclass">)  [unwired: 7 in]
          n459 = Increment(x=w1386) -> (x+1=w1387:i32)
        }
        frame 91 {
          w1397 = "DONE"
          # "Volta pra repouso para que os indicadores de progresso da aquisição sejam atualizados na GUI."
          n460 = call-dynamic "Read resp.vi"("error in (no error)"=w1402, "Device in"=w1403) -> ("error out"=w1400:errorcluster, "resp"=w1399:string, "Device out"=w1401:refnum<class "Channel.lvclass">)  [unwired: 7 in]
          "resp PAUSE" <- w1399
          n461 = Match Pattern(string=w1399, regular expression=w1397) -> (match substring=w1398:string)  [unwired: 1 in, 3 out]
          n462 = Equal?(x=w1398, y=w1397) -> ()  [unwired: 1 out]
        }
        frame 96 {
          n463 = Unbundle By Name(w1405) -> ("wait_expose"=w1404:bool)
          n464 = case shown="False" w1404 {
            tunnel: w1413 -> [w1418 w1419]
            tunnel: w1405 -> [w1417 w1420]
            tunnel: [w1416 w1420] -> w1410
            tunnel: [w1415 w1419] -> w1409
            frame False {
              # "20240710: Se o ACS não estiver\nesperando EXPOSE, manda reiniciar\na aquisição."
              n465 = call-dynamic "Write cmd.vi"("error in (no error)"=w1418, "cmd"="RESUME_ACQUISITION", "Device in"=w1417) -> ("error out"=w1415:errorcluster, "Device out"=w1416:refnum<class "Channel.lvclass">)  [unwired: 7 in]
            }
            frame True {
            }
          }
          n466 = call-dynamic "Write resp.vi"("error in (no error)"=w1409, "resp"="", "Device in"=w1410) -> ("error out"=w1408:errorcluster, "Device out"=w1407:refnum<class "Channel.lvclass">)  [unwired: 7 in]
          n467 = Increment(x=w1411) -> (x+1=w1412:i32)
        }
        frame 97 {
          w1423 = "DONE"
          # "No estado 500 de S4GUI:HandleObservationSync.vi e S4GUI:HandleObservationAsync.vi\né feita a verificação se o canal foi pra repouso (estados 0,56,57 de Channel:Run.vi). \nSe foi, o estado de retorno do canal é recarregado e o processo continua de onde parou."
          n468 = call-dynamic "Read resp.vi"("error in (no error)"=w1427, "Device in"=w1428) -> ("error out"=w1422:errorcluster, "resp"=w1425:string, "Device out"=w1426:refnum<class "Channel.lvclass">)  [unwired: 7 in]
          "resp RESUME" <- w1425
          n469 = Match Pattern(string=w1425, regular expression=w1423) -> (match substring=w1424:string)  [unwired: 1 in, 3 out]
          n470 = Equal?(x=w1424, y=w1423) -> ()  [unwired: 1 out]
        }
        frame 100 {
          (unwired) "S4ACS C1/C2/C3/C4 NIMAGES " ("cmd")
          n471 = call-dynamic "Write cmd.vi"("error in (no error)"=w1434, "cmd"="INIT", "Device in"=w1432) -> ("error out"=w1433:errorcluster, "Device out"=w1435:refnum<class "Channel.lvclass">)  [unwired: 7 in]
          n472 = Increment(x=w1430) -> (x+1=w1431:i32)
        }
        frame 101 {
          w1437 = "\r\n"
          n473 = call-dynamic "Read resp.vi"("error in (no error)"=w1445, "Device in"=w1446) -> ("error out"=w1442:errorcluster, "resp"=w1436:string, "Device out"=w1439:refnum<class "Channel.lvclass">)  [unwired: 7 in]
          n474 = Match Pattern(string=w1436, regular expression=w1437) -> (match substring=w1440:string)  [unwired: 1 in, 3 out]
          n475 = Equal?(x=w1440, y=w1437) -> (x = y?=w1444:bool)
          n476 = case shown="False" w1444 {
            tunnel: [w1447 u8 0] -> w1443
            tunnel: w1441 -> [w1447 _]
            tunnel: w1439 -> [w1448 w1452]
            tunnel: [w1448 w1451] -> w1438
            tunnel: w1436 -> [_ w1450]
            frame False {
            }
            frame True {
              n477 = Bundle By Name(cluster=w1452, "lastStatus"=w1450) -> (w1451:refnum<class "Channel.lvclass">)
            }
          }
        }
        frame 102 {
          w1460 = "EXPTIME "
          n478 = Unbundle By Name(w1454) -> ("lastStatus"=w1455:string)
          n479 = Match Pattern(string=w1455, regular expression=w1460) -> (match substring=w1459:string, after substring=w1457:string)  [unwired: 1 in, 2 out]
          n480 = Equal?(x=w1459, y=w1460) -> (x = y?=w1463:bool)
          n481 = case shown="True" w1463 {
            tunnel: [w1464 w1466] -> w1462
            tunnel: w1461 -> [w1464 w1466]
            tunnel: w1454 -> [w1465 w1472]
            tunnel: [w1465 w1470] -> w1458
            tunnel: w1457 -> [_ w1468]
            frame False {
            }
            frame True {
              n482 = call <vilib>:"Space Constant.vi"() -> ("String"=w1469:string)
              n483 = Match Pattern(string=w1468, regular expression=w1469) -> (before substring=w1467:string)  [unwired: 1 in, 3 out]
              n484 = Fract/Exp String To Number(string=w1467) -> (number=w1471:dbl)  [unwired: 3 in, 1 out]
              n485 = Bundle By Name(cluster=w1472, "Texp"=w1471) -> (w1470:refnum<class "Channel.lvclass">)
            }
          }
          n486 = Increment(x=w1462) -> (x+1=w1453:i32)
        }
        frame 103 {
          w1480 = "NIMAGES "
          n487 = Unbundle By Name(w1474) -> ("lastStatus"=w1475:string)
          n488 = Match Pattern(string=w1475, regular expression=w1480) -> (match substring=w1479:string, after substring=w1477:string)  [unwired: 1 in, 2 out]
          n489 = Equal?(x=w1479, y=w1480) -> (x = y?=w1483:bool)
          n490 = case shown="True" w1483 {
            tunnel: [w1484 w1486] -> w1482
            tunnel: w1481 -> [w1484 w1486]
            tunnel: w1474 -> [w1485 w1492]
            tunnel: [w1485 w1490] -> w1478
            tunnel: w1477 -> [_ w1488]
            frame False {
            }
            frame True {
              n491 = call <vilib>:"Space Constant.vi"() -> ("String"=w1489:string)
              n492 = Match Pattern(string=w1488, regular expression=w1489) -> (before substring=w1487:string)  [unwired: 1 in, 3 out]
              n493 = Fract/Exp String To Number(string=w1487) -> (number=w1491:dbl)  [unwired: 3 in, 1 out]
              n494 = Bundle By Name(cluster=w1492, "Nimages"=w1491) -> (w1490:refnum<class "Channel.lvclass">)
            }
          }
          n495 = Increment(x=w1482) -> (x+1=w1473:i32)
        }
        frame 104 {
          w1500 = "INITIAL_LINE "
          n496 = Unbundle By Name(w1494) -> ("lastStatus"=w1495:string)
          n497 = Match Pattern(string=w1495, regular expression=w1500) -> (match substring=w1499:string, after substring=w1497:string)  [unwired: 1 in, 2 out]
          n498 = Equal?(x=w1499, y=w1500) -> (x = y?=w1503:bool)
          n499 = case shown="True" w1503 {
            tunnel: [w1504 w1506] -> w1502
            tunnel: w1501 -> [w1504 w1506]
            tunnel: w1494 -> [w1505 w1512]
            tunnel: [w1505 w1510] -> w1498
            tunnel: w1497 -> [_ w1508]
            frame False {
            }
            frame True {
              n500 = call <vilib>:"Space Constant.vi"() -> ("String"=w1509:string)
              n501 = Match Pattern(string=w1508, regular expression=w1509) -> (before substring=w1507:string)  [unwired: 1 in, 3 out]
              n502 = Fract/Exp String To Number(string=w1507) -> (number=w1511:dbl)  [unwired: 3 in, 1 out]
              n503 = Bundle By Name(cluster=w1512, "InitialLine"=w1511) -> (w1510:refnum<class "Channel.lvclass">)
            }
          }
          n504 = Increment(x=w1502) -> (x+1=w1493:i32)
        }
        frame 105 {
          w1520 = "FINAL_LINE "
          n505 = Unbundle By Name(w1514) -> ("lastStatus"=w1515:string)
          n506 = Match Pattern(string=w1515, regular expression=w1520) -> (match substring=w1519:string, after substring=w1517:string)  [unwired: 1 in, 2 out]
          n507 = Equal?(x=w1519, y=w1520) -> (x = y?=w1523:bool)
          n508 = case shown="True" w1523 {
            tunnel: [w1524 w1526] -> w1522
            tunnel: w1521 -> [w1524 w1526]
            tunnel: w1514 -> [w1525 w1532]
            tunnel: [w1525 w1530] -> w1518
            tunnel: w1517 -> [_ w1528]
            frame False {
            }
            frame True {
              n509 = call <vilib>:"Space Constant.vi"() -> ("String"=w1529:string)
              n510 = Match Pattern(string=w1528, regular expression=w1529) -> (before substring=w1527:string)  [unwired: 1 in, 3 out]
              n511 = Fract/Exp String To Number(string=w1527) -> (number=w1531:dbl)  [unwired: 3 in, 1 out]
              n512 = Bundle By Name(cluster=w1532, "FinalLine"=w1531) -> (w1530:refnum<class "Channel.lvclass">)
            }
          }
          n513 = Increment(x=w1522) -> (x+1=w1513:i32)
        }
        frame 106 {
          w1540 = "INITIAL_COLUMN "
          n514 = Unbundle By Name(w1534) -> ("lastStatus"=w1535:string)
          n515 = Match Pattern(string=w1535, regular expression=w1540) -> (match substring=w1539:string, after substring=w1537:string)  [unwired: 1 in, 2 out]
          n516 = Equal?(x=w1539, y=w1540) -> (x = y?=w1543:bool)
          n517 = case shown="True" w1543 {
            tunnel: [w1544 w1546] -> w1542
            tunnel: w1541 -> [w1544 w1546]
            tunnel: w1534 -> [w1545 w1552]
            tunnel: [w1545 w1550] -> w1538
            tunnel: w1537 -> [_ w1548]
            frame False {
            }
            frame True {
              n518 = call <vilib>:"Space Constant.vi"() -> ("String"=w1549:string)
              n519 = Match Pattern(string=w1548, regular expression=w1549) -> (before substring=w1547:string)  [unwired: 1 in, 3 out]
              n520 = Fract/Exp String To Number(string=w1547) -> (number=w1551:dbl)  [unwired: 3 in, 1 out]
              n521 = Bundle By Name(cluster=w1552, "InitialColumn"=w1551) -> (w1550:refnum<class "Channel.lvclass">)
            }
          }
          n522 = Increment(x=w1542) -> (x+1=w1533:i32)
        }
        frame 107 {
          w1560 = "FINAL_COLUMN "
          n523 = Unbundle By Name(w1554) -> ("lastStatus"=w1555:string)
          n524 = Match Pattern(string=w1555, regular expression=w1560) -> (match substring=w1559:string, after substring=w1557:string)  [unwired: 1 in, 2 out]
          n525 = Equal?(x=w1559, y=w1560) -> (x = y?=w1563:bool)
          n526 = case shown="True" w1563 {
            tunnel: [w1564 w1566] -> w1562
            tunnel: w1561 -> [w1564 w1566]
            tunnel: w1554 -> [w1565 w1572]
            tunnel: [w1565 w1570] -> w1558
            tunnel: w1557 -> [_ w1568]
            frame False {
            }
            frame True {
              n527 = call <vilib>:"Space Constant.vi"() -> ("String"=w1569:string)
              n528 = Match Pattern(string=w1568, regular expression=w1569) -> (before substring=w1567:string)  [unwired: 1 in, 3 out]
              n529 = Fract/Exp String To Number(string=w1567) -> (number=w1571:dbl)  [unwired: 3 in, 1 out]
              n530 = Bundle By Name(cluster=w1572, "FinalColumn"=w1571) -> (w1570:refnum<class "Channel.lvclass">)
            }
          }
          n531 = Increment(x=w1562) -> (x+1=w1553:i32)
        }
        frame 108 {
          w1580 = "EM_GAIN "
          n532 = Unbundle By Name(w1574) -> ("lastStatus"=w1575:string)
          n533 = Match Pattern(string=w1575, regular expression=w1580) -> (match substring=w1579:string, after substring=w1577:string)  [unwired: 1 in, 2 out]
          n534 = Equal?(x=w1579, y=w1580) -> (x = y?=w1583:bool)
          n535 = case shown="True" w1583 {
            tunnel: [w1584 w1586] -> w1582
            tunnel: w1581 -> [w1584 w1586]
            tunnel: w1574 -> [w1585 w1592]
            tunnel: [w1585 w1590] -> w1578
            tunnel: w1577 -> [_ w1588]
            frame False {
            }
            frame True {
              n536 = call <vilib>:"Space Constant.vi"() -> ("String"=w1589:string)
              n537 = Match Pattern(string=w1588, regular expression=w1589) -> (before substring=w1587:string)  [unwired: 1 in, 3 out]
              n538 = Fract/Exp String To Number(string=w1587) -> (number=w1591:dbl)  [unwired: 3 in, 1 out]
              n539 = Bundle By Name(cluster=w1592, "EmGain"=w1591) -> (w1590:refnum<class "Channel.lvclass">)
            }
          }
          n540 = Increment(x=w1582) -> (x+1=w1573:i32)
        }
        frame 109 {
          w1600 = "COOLER "
          n541 = Unbundle By Name(w1594) -> ("lastStatus"=w1595:string)
          n542 = Match Pattern(string=w1595, regular expression=w1600) -> (match substring=w1599:string, after substring=w1597:string)  [unwired: 1 in, 2 out]
          n543 = Equal?(x=w1599, y=w1600) -> (x = y?=w1603:bool)
          n544 = case shown="True" w1603 {
            tunnel: [w1604 w1606] -> w1602
            tunnel: w1601 -> [w1604 w1606]
            tunnel: w1594 -> [w1605 w1613]
            tunnel: [w1605 w1612] -> w1598
            tunnel: w1597 -> [_ w1610]
            frame False {
            }
            frame True {
              n545 = call <vilib>:"Space Constant.vi"() -> ("String"=w1611:string)
              n546 = Match Pattern(string=w1610, regular expression=w1611) -> (before substring=w1609:string)  [unwired: 1 in, 3 out]
              n547 = Equal?(x=w1609, y="ON") -> (x = y?=w1607:bool)
              n548 = Bundle By Name(cluster=w1613, "Cooler Off"=w1607) -> (w1612:refnum<class "Channel.lvclass">)
            }
          }
          n549 = Increment(x=w1602) -> (x+1=w1593:i32)
        }
        frame 110 {
        }
        frame 200 {
          n550 = Unbundle By Name(w1625) -> ("Interface.lvclass"=w1624:refnum<class "Interface.lvclass">)
          n551 = call "Read Camera Setup.vi"("Interface in"=w1624) -> ("Camera Setup"=w1618:T4)  [unwired: 8 in, 2 out]
          n552 = Unbundle By Name(w1618) -> ("EXPTIME"=w1617:dbl)
          n553 = Number To Fractional String(number=w1617) -> (F-format string=w1619:string)  [unwired: 3 in]
          n554 = Concatenate Strings("SET EXPTIME " ("cmd"), w1619) -> (w1623:string)
          n555 = call-dynamic "Write cmd.vi"("error in (no error)"=w1627, "cmd"=w1623, "Device in"=w1625) -> ("error out"=w1626:errorcluster, "Device out"=w1628:refnum<class "Channel.lvclass">)  [unwired: 7 in]
          n556 = Increment(x=w1621) -> (x+1=w1622:i32)
        }
        frame 201 {
          n557 = call-dynamic "Read resp.vi"("error in (no error)"=w1636, "Device in"=w1637) -> ("error out"=w1630:errorcluster, "resp"=w1635:string, "Device out"=w1631:refnum<class "Channel.lvclass">)  [unwired: 7 in]
          n558 = Equal?(x=w1635, y="DONE") -> (x = y?=w1633:bool)
          n559 = case shown="True" w1633 {
            tunnel: [w1638 w1639] -> w1632
            tunnel: w1629 -> [w1638 w1640]
            frame False {
            }
            frame True {
              n560 = Increment(x=w1640) -> (x+1=w1639:i32)
            }
          }
        }
        frame 202 {
          n561 = call-dynamic "Write cmd.vi"("error in (no error)"=w1646, "cmd"="GET EXPTIME", "Device in"=w1644) -> ("error out"=w1645:errorcluster, "Device out"=w1647:refnum<class "Channel.lvclass">)  [unwired: 7 in]
          n562 = Increment(x=w1642) -> (x+1=w1643:i32)
        }
        frame 203 {
          n563 = call-dynamic "Read resp.vi"("error in (no error)"=w1658, "Device in"=w1659) -> ("error out"=w1656:errorcluster, "resp"=w1651:string, "Device out"=w1654:refnum<class "Channel.lvclass">)  [unwired: 7 in]
          n564 = Fract/Exp String To Number(string=w1651) -> (number=w1648:dbl)  [unwired: 3 in, 1 out]
          n565 = Unbundle By Name(w1654) -> ("Interface.lvclass"=w1653:refnum<class "Interface.lvclass">)
          n566 = call "Read Camera Setup.vi"("Interface in"=w1653) -> ("Camera Setup"=w1652:T4)  [unwired: 8 in, 2 out]
          n567 = Unbundle By Name(w1652) -> ("EXPTIME"=w1649:dbl)
          n568 = Equal?(x=w1649, y=w1648) -> (x = y?=w1650:bool)
          n569 = disable-structure shown="Enabled" {
            disable-tunnel: [w1662 224 ("State")] -> w1657
            disable-tunnel: w1655 -> [w1661 _]
            disable-tunnel: w1650 -> [w1660 _]
            frame Disabled {
              n570 = case shown="True" w1660 {
                tunnel: [w1663 w1664] -> w1662
                tunnel: w1661 -> [w1663 w1665]
                frame False {
                }
                frame True {
                  n571 = Increment(x=w1665) -> (x+1=w1664:i32)
                }
              }
            }
            frame Enabled {
            }
          }
        }
        frame 204 {
          n572 = Unbundle By Name(w1675) -> ("Interface.lvclass"=w1674:refnum<class "Interface.lvclass">)
          n573 = call "Read Camera Setup.vi"("Interface in"=w1674) -> ("Camera Setup"=w1668:T4)  [unwired: 8 in, 2 out]
          n574 = Unbundle By Name(w1668) -> ("#FRAMES"=w1667:u32)
          n575 = Number To Fractional String(number=w1667) -> (F-format string=w1669:string)  [unwired: 3 in]
          n576 = Concatenate Strings("SET #FRAMES " ("cmd"), w1669) -> (w1673:string)
          n577 = call-dynamic "Write cmd.vi"("error in (no error)"=w1677, "cmd"=w1673, "Device in"=w1675) -> ("error out"=w1676:errorcluster, "Device out"=w1678:refnum<class "Channel.lvclass">)  [unwired: 7 in]
          n578 = Increment(x=w1671) -> (x+1=w1672:i32)
        }
        frame 205 {
          n579 = call-dynamic "Read resp.vi"("error in (no error)"=w1686, "Device in"=w1687) -> ("error out"=w1680:errorcluster, "resp"=w1685:string, "Device out"=w1681:refnum<class "Channel.lvclass">)  [unwired: 7 in]
          n580 = Equal?(x=w1685, y="DONE") -> (x = y?=w1683:bool)
          n581 = case shown="True" w1683 {
            tunnel: [w1688 w1689] -> w1682
            tunnel: w1679 -> [w1688 w1690]
            frame False {
            }
            frame True {
              n582 = Increment(x=w1690) -> (x+1=w1689:i32)
            }
          }
        }
        frame 206 {
          n583 = call-dynamic "Write cmd.vi"("error in (no error)"=w1696, "cmd"="GET #FRAMES", "Device in"=w1694) -> ("error out"=w1695:errorcluster, "Device out"=w1697:refnum<class "Channel.lvclass">)  [unwired: 7 in]
          n584 = Increment(x=w1692) -> (x+1=w1693:i32)
        }
        frame 207 {
          n585 = call-dynamic "Read resp.vi"("error in (no error)"=w1709, "Device in"=w1710) -> ("error out"=w1707:errorcluster, "resp"=w1702:string, "Device out"=w1705:refnum<class "Channel.lvclass">)  [unwired: 7 in]
          n586 = Decimal String To Number(string=w1702) -> (number=w1700:i32)  [unwired: 2 in, 1 out]
          n587 = Unbundle By Name(w1705) -> ("Interface.lvclass"=w1704:refnum<class "Interface.lvclass">)
          n588 = call "Read Camera Setup.vi"("Interface in"=w1704) -> ("Camera Setup"=w1703:T4)  [unwired: 8 in, 2 out]
          n589 = To Unsigned Long Integer(number=w1700) -> (unsigned 32bit integer=w1698:u32)
          n590 = Unbundle By Name(w1703) -> ("#FRAMES"=w1699:u32)
          n591 = Equal?(x=w1699, y=w1698) -> (x = y?=w1701:bool)
          n592 = case shown="True" w1701 {
            tunnel: [w1711 w1712] -> w1708
            tunnel: w1706 -> [w1711 w1713]
            frame False {
            }
            frame True {
              n593 = Increment(x=w1713) -> (x+1=w1712:i32)
            }
          }
        }
        frame 208 {
          n594 = Unbundle By Name(w1722) -> ("Interface.lvclass"=w1721:refnum<class "Interface.lvclass">)
          n595 = call "Read Camera Setup.vi"("Interface in"=w1721) -> ("Camera Setup"=w1715:T4)  [unwired: 8 in, 2 out]
          n596 = Unbundle By Name(w1715) -> ("TRIGGER_MODE"=w1714:u8)
          n597 = Number To Fractional String(number=w1714) -> (F-format string=w1716:string)  [unwired: 3 in]
          n598 = Concatenate Strings("SET TRIGGER_MODE " ("cmd"), w1716) -> (w1720:string)
          n599 = call-dynamic "Write cmd.vi"("error in (no error)"=w1724, "cmd"=w1720, "Device in"=w1722) -> ("error out"=w1723:errorcluster, "Device out"=w1725:refnum<class "Channel.lvclass">)  [unwired: 7 in]
          n600 = Increment(x=w1718) -> (x+1=w1719:i32)
        }
        frame 209 {
          n601 = call-dynamic "Read resp.vi"("error in (no error)"=w1733, "Device in"=w1734) -> ("error out"=w1727:errorcluster, "resp"=w1732:string, "Device out"=w1728:refnum<class "Channel.lvclass">)  [unwired: 7 in]
          n602 = Equal?(x=w1732, y="DONE") -> (x = y?=w1730:bool)
          n603 = case shown="True" w1730 {
            tunnel: [w1735 w1736] -> w1729
            tunnel: w1726 -> [w1735 w1737]
            frame False {
            }
            frame True {
              n604 = Increment(x=w1737) -> (x+1=w1736:i32)
            }
          }
        }
        frame 210 {
          n605 = call-dynamic "Write cmd.vi"("error in (no error)"=w1743, "cmd"="GET TRIGGER_MODE", "Device in"=w1741) -> ("error out"=w1742:errorcluster, "Device out"=w1744:refnum<class "Channel.lvclass">)  [unwired: 7 in]
          n606 = Increment(x=w1739) -> (x+1=w1740:i32)
        }
        frame 211 {
          n607 = call-dynamic "Read resp.vi"("error in (no error)"=w1755, "Device in"=w1756) -> ("error out"=w1753:errorcluster, "resp"=w1748:string, "Device out"=w1751:refnum<class "Channel.lvclass">)  [unwired: 7 in]
          n608 = Fract/Exp String To Number(string=w1748) -> (number=w1746:dbl)  [unwired: 3 in, 1 out]
          n609 = Unbundle By Name(w1751) -> ("Interface.lvclass"=w1750:refnum<class "Interface.lvclass">)
          n610 = call "Read Camera Setup.vi"("Interface in"=w1750) -> ("Camera Setup"=w1749:T4)  [unwired: 8 in, 2 out]
          n611 = Unbundle By Name(w1749) -> ("TRIGGER_MODE"=w1745:u8)
          n612 = Equal?(x=w1745, y=w1746) -> (x = y?=w1747:bool)
          n613 = case shown="False" w1747 {
            tunnel: [w1757 w1758] -> w1754
            tunnel: w1752 -> [w1757 w1759]
            frame False {
            }
            frame True {
              n614 = Increment(x=w1759) -> (x+1=w1758:i32)
            }
          }
        }
        frame 212 {
          n615 = Unbundle By Name(w1768) -> ("Interface.lvclass"=w1767:refnum<class "Interface.lvclass">)
          n616 = call "Read Camera Setup.vi"("Interface in"=w1767) -> ("Camera Setup"=w1761:T4)  [unwired: 8 in, 2 out]
          n617 = Unbundle By Name(w1761) -> ("READ_MODE"=w1760:u8)
          n618 = Number To Fractional String(number=w1760) -> (F-format string=w1762:string)  [unwired: 3 in]
          n619 = Concatenate Strings("SET READ_MODE " ("cmd"), w1762) -> (w1766:string)
          n620 = call-dynamic "Write cmd.vi"("error in (no error)"=w1770, "cmd"=w1766, "Device in"=w1768) -> ("error out"=w1769:errorcluster, "Device out"=w1771:refnum<class "Channel.lvclass">)  [unwired: 7 in]
          n621 = Increment(x=w1764) -> (x+1=w1765:i32)
        }
        frame 213 {
          n622 = call-dynamic "Read resp.vi"("error in (no error)"=w1779, "Device in"=w1780) -> ("error out"=w1773:errorcluster, "resp"=w1778:string, "Device out"=w1774:refnum<class "Channel.lvclass">)  [unwired: 7 in]
          n623 = Equal?(x=w1778, y="DONE") -> (x = y?=w1776:bool)
          n624 = case shown="True" w1776 {
            tunnel: [w1781 w1782] -> w1775
            tunnel: w1772 -> [w1781 w1783]
            frame False {
            }
            frame True {
              n625 = Increment(x=w1783) -> (x+1=w1782:i32)
            }
          }
        }
        frame 214 {
          n626 = call-dynamic "Write cmd.vi"("error in (no error)"=w1789, "cmd"="GET READ_MODE", "Device in"=w1787) -> ("error out"=w1788:errorcluster, "Device out"=w1790:refnum<class "Channel.lvclass">)  [unwired: 7 in]
          n627 = Increment(x=w1785) -> (x+1=w1786:i32)
        }
        frame 215 {
          n628 = call-dynamic "Read resp.vi"("error in (no error)"=w1801, "Device in"=w1802) -> ("error out"=w1799:errorcluster, "resp"=w1794:string, "Device out"=w1797:refnum<class "Channel.lvclass">)  [unwired: 7 in]
          n629 = Fract/Exp String To Number(string=w1794) -> (number=w1792:dbl)  [unwired: 3 in, 1 out]
          n630 = Unbundle By Name(w1797) -> ("Interface.lvclass"=w1796:refnum<class "Interface.lvclass">)
          n631 = call "Read Camera Setup.vi"("Interface in"=w1796) -> ("Camera Setup"=w1795:T4)  [unwired: 8 in, 2 out]
          n632 = Unbundle By Name(w1795) -> ("READ_MODE"=w1791:u8)
          n633 = Equal?(x=w1791, y=w1792) -> (x = y?=w1793:bool)
          n634 = case shown="True" w1793 {
            tunnel: [w1803 w1804] -> w1800
            tunnel: w1798 -> [w1803 w1805]
            frame False {
            }
            frame True {
              n635 = Increment(x=w1805) -> (x+1=w1804:i32)
            }
          }
        }
        frame 216 {
          n636 = Unbundle By Name(w1814) -> ("Interface.lvclass"=w1813:refnum<class "Interface.lvclass">)
          n637 = call "Read Camera Setup.vi"("Interface in"=w1813) -> ("Camera Setup"=w1807:T4)  [unwired: 8 in, 2 out]
          n638 = Unbundle By Name(w1807) -> ("READOUT_RATE"=w1806:u8)
          n639 = Number To Fractional String(number=w1806) -> (F-format string=w1808:string)  [unwired: 3 in]
          n640 = Concatenate Strings("SET READOUT_RATE " ("cmd"), w1808) -> (w1812:string)
          n641 = call-dynamic "Write cmd.vi"("error in (no error)"=w1816, "cmd"=w1812, "Device in"=w1814) -> ("error out"=w1815:errorcluster, "Device out"=w1817:refnum<class "Channel.lvclass">)  [unwired: 7 in]
          n642 = Increment(x=w1810) -> (x+1=w1811:i32)
        }
        frame 217 {
          n643 = call-dynamic "Read resp.vi"("error in (no error)"=w1825, "Device in"=w1826) -> ("error out"=w1819:errorcluster, "resp"=w1824:string, "Device out"=w1820:refnum<class "Channel.lvclass">)  [unwired: 7 in]
          n644 = Equal?(x=w1824, y="DONE") -> (x = y?=w1822:bool)
          n645 = case shown="True" w1822 {
            tunnel: [w1827 w1828] -> w1821
            tunnel: w1818 -> [w1827 w1829]
            frame False {
            }
            frame True {
              n646 = Increment(x=w1829) -> (x+1=w1828:i32)
            }
          }
        }
        frame 218 {
          n647 = call-dynamic "Write cmd.vi"("error in (no error)"=w1835, "cmd"="GET READOUT_RATE", "Device in"=w1833) -> ("error out"=w1834:errorcluster, "Device out"=w1836:refnum<class "Channel.lvclass">)  [unwired: 7 in]
          n648 = Increment(x=w1831) -> (x+1=w1832:i32)
        }
        frame 219 {
          n649 = call-dynamic "Read resp.vi"("error in (no error)"=w1847, "Device in"=w1848) -> ("error out"=w1845:errorcluster, "resp"=w1840:string, "Device out"=w1843:refnum<class "Channel.lvclass">)  [unwired: 7 in]
          n650 = Fract/Exp String To Number(string=w1840) -> (number=w1838:dbl)  [unwired: 3 in, 1 out]
          n651 = Unbundle By Name(w1843) -> ("Interface.lvclass"=w1842:refnum<class "Interface.lvclass">)
          n652 = call "Read Camera Setup.vi"("Interface in"=w1842) -> ("Camera Setup"=w1841:T4)  [unwired: 8 in, 2 out]
          n653 = Unbundle By Name(w1841) -> ("READOUT_RATE"=w1837:u8)
          n654 = Equal?(x=w1837, y=w1838) -> (x = y?=w1839:bool)
          n655 = case shown="True" w1839 {
            tunnel: [w1849 w1850] -> w1846
            tunnel: w1844 -> [w1849 w1851]
            frame False {
            }
            frame True {
              n656 = Increment(x=w1851) -> (x+1=w1850:i32)
            }
          }
        }
        frame 220 {
          n657 = Unbundle By Name(w1860) -> ("Interface.lvclass"=w1859:refnum<class "Interface.lvclass">)
          n658 = call "Read Camera Setup.vi"("Interface in"=w1859) -> ("Camera Setup"=w1853:T4)  [unwired: 8 in, 2 out]
          n659 = Unbundle By Name(w1853) -> ("VERTICAL_SHIFT_SPEED"=w1852:u8)
          n660 = Number To Fractional String(number=w1852) -> (F-format string=w1854:string)  [unwired: 3 in]
          n661 = Concatenate Strings("SET VERTICAL_SHIFT_SPEED " ("cmd"), w1854) -> (w1858:string)
          n662 = call-dynamic "Write cmd.vi"("error in (no error)"=w1862, "cmd"=w1858, "Device in"=w1860) -> ("error out"=w1861:errorcluster, "Device out"=w1863:refnum<class "Channel.lvclass">)  [unwired: 7 in]
          n663 = Increment(x=w1856) -> (x+1=w1857:i32)
        }
        frame 221 {
          n664 = call-dynamic "Read resp.vi"("error in (no error)"=w1871, "Device in"=w1872) -> ("error out"=w1865:errorcluster, "resp"=w1870:string, "Device out"=w1866:refnum<class "Channel.lvclass">)  [unwired: 7 in]
          n665 = Equal?(x=w1870, y="DONE") -> (x = y?=w1868:bool)
          n666 = case shown="True" w1868 {
            tunnel: [w1873 w1874] -> w1867
            tunnel: w1864 -> [w1873 w1875]
            frame False {
            }
            frame True {
              n667 = Increment(x=w1875) -> (x+1=w1874:i32)
            }
          }
        }
        frame 222 {
          n668 = call-dynamic "Write cmd.vi"("error in (no error)"=w1881, "cmd"="GET VERTICAL_SHIFT_SPEED", "Device in"=w1879) -> ("error out"=w1880:errorcluster, "Device out"=w1882:refnum<class "Channel.lvclass">)  [unwired: 7 in]
          n669 = Increment(x=w1877) -> (x+1=w1878:i32)
        }
        frame 223 {
          n670 = call-dynamic "Read resp.vi"("error in (no error)"=w1893, "Device in"=w1894) -> ("error out"=w1891:errorcluster, "resp"=w1886:string, "Device out"=w1889:refnum<class "Channel.lvclass">)  [unwired: 7 in]
          n671 = Fract/Exp String To Number(string=w1886) -> (number=w1884:dbl)  [unwired: 3 in, 1 out]
          n672 = Unbundle By Name(w1889) -> ("Interface.lvclass"=w1888:refnum<class "Interface.lvclass">)
          n673 = call "Read Camera Setup.vi"("Interface in"=w1888) -> ("Camera Setup"=w1887:T4)  [unwired: 8 in, 2 out]
          n674 = Unbundle By Name(w1887) -> ("VERTICAL_SHIFT_SPEED"=w1883:u8)
          n675 = Equal?(x=w1883, y=w1884) -> (x = y?=w1885:bool)
          n676 = case shown="True" w1885 {
            tunnel: [w1895 w1896] -> w1892
            tunnel: w1890 -> [w1895 w1897]
            frame False {
            }
            frame True {
              n677 = Increment(x=w1897) -> (x+1=w1896:i32)
            }
          }
        }
        frame 224 {
          n678 = Unbundle By Name(w1906) -> ("Interface.lvclass"=w1905:refnum<class "Interface.lvclass">)
          n679 = call "Read Camera Setup.vi"("Interface in"=w1905) -> ("Camera Setup"=w1899:T4)  [unwired: 8 in, 2 out]
          n680 = Unbundle By Name(w1899) -> ("PREAMP"=w1898:u8)
          n681 = Number To Fractional String(number=w1898) -> (F-format string=w1900:string)  [unwired: 3 in]
          n682 = Concatenate Strings("SET PREAMP " ("cmd"), w1900) -> (w1904:string)
          n683 = call-dynamic "Write cmd.vi"("error in (no error)"=w1908, "cmd"=w1904, "Device in"=w1906) -> ("error out"=w1907:errorcluster, "Device out"=w1909:refnum<class "Channel.lvclass">)  [unwired: 7 in]
          n684 = Increment(x=w1902) -> (x+1=w1903:i32)
        }
        frame 225 {
          n685 = call-dynamic "Read resp.vi"("error in (no error)"=w1917, "Device in"=w1918) -> ("error out"=w1911:errorcluster, "resp"=w1916:string, "Device out"=w1912:refnum<class "Channel.lvclass">)  [unwired: 7 in]
          n686 = Equal?(x=w1916, y="DONE") -> (x = y?=w1914:bool)
          n687 = case shown="True" w1914 {
            tunnel: [w1919 w1920] -> w1913
            tunnel: w1910 -> [w1919 w1921]
            frame False {
            }
            frame True {
              n688 = Increment(x=w1921) -> (x+1=w1920:i32)
            }
          }
        }
        frame 226 {
          n689 = call-dynamic "Write cmd.vi"("error in (no error)"=w1927, "cmd"="GET PREAMP", "Device in"=w1925) -> ("error out"=w1926:errorcluster, "Device out"=w1928:refnum<class "Channel.lvclass">)  [unwired: 7 in]
          n690 = Increment(x=w1923) -> (x+1=w1924:i32)
        }
        frame 227 {
          n691 = call-dynamic "Read resp.vi"("error in (no error)"=w1939, "Device in"=w1940) -> ("error out"=w1937:errorcluster, "resp"=w1932:string, "Device out"=w1935:refnum<class "Channel.lvclass">)  [unwired: 7 in]
          n692 = Fract/Exp String To Number(string=w1932) -> (number=w1930:dbl)  [unwired: 3 in, 1 out]
          n693 = Unbundle By Name(w1935) -> ("Interface.lvclass"=w1934:refnum<class "Interface.lvclass">)
          n694 = call "Read Camera Setup.vi"("Interface in"=w1934) -> ("Camera Setup"=w1933:T4)  [unwired: 8 in, 2 out]
          n695 = Unbundle By Name(w1933) -> ("PREAMP"=w1929:u8)
          n696 = Equal?(x=w1929, y=w1930) -> (x = y?=w1931:bool)
          n697 = case shown="True" w1931 {
            tunnel: [w1941 w1942] -> w1938
            tunnel: w1936 -> [w1941 w1943]
            frame False {
            }
            frame True {
              n698 = Increment(x=w1943) -> (x+1=w1942:i32)
            }
          }
        }
        frame 228 {
          n699 = Unbundle By Name(w1952) -> ("Interface.lvclass"=w1951:refnum<class "Interface.lvclass">)
          n700 = call "Read Camera Setup.vi"("Interface in"=w1951) -> ("Camera Setup"=w1945:T4)  [unwired: 8 in, 2 out]
          n701 = Unbundle By Name(w1945) -> ("EM_MODE"=w1944:u8)
          n702 = Number To Fractional String(number=w1944) -> (F-format string=w1946:string)  [unwired: 3 in]
          n703 = Concatenate Strings("SET EM_MODE " ("cmd"), w1946) -> (w1950:string)
          n704 = call-dynamic "Write cmd.vi"("error in (no error)"=w1954, "cmd"=w1950, "Device in"=w1952) -> ("error out"=w1953:errorcluster, "Device out"=w1955:refnum<class "Channel.lvclass">)  [unwired: 7 in]
          n705 = Increment(x=w1948) -> (x+1=w1949:i32)
        }
        frame 229 {
          n706 = call-dynamic "Read resp.vi"("error in (no error)"=w1963, "Device in"=w1964) -> ("error out"=w1957:errorcluster, "resp"=w1962:string, "Device out"=w1958:refnum<class "Channel.lvclass">)  [unwired: 7 in]
          n707 = Equal?(x=w1962, y="DONE") -> (x = y?=w1960:bool)
          n708 = case shown="True" w1960 {
            tunnel: [w1965 w1966] -> w1959
            tunnel: w1956 -> [w1965 w1967]
            frame False {
            }
            frame True {
              n709 = Increment(x=w1967) -> (x+1=w1966:i32)
            }
          }
        }
        frame 230 {
          n710 = call-dynamic "Write cmd.vi"("error in (no error)"=w1973, "cmd"="GET EM_MODE", "Device in"=w1971) -> ("error out"=w1972:errorcluster, "Device out"=w1974:refnum<class "Channel.lvclass">)  [unwired: 7 in]
          n711 = Increment(x=w1969) -> (x+1=w1970:i32)
        }
        frame 231 {
          n712 = call-dynamic "Read resp.vi"("error in (no error)"=w1985, "Device in"=w1986) -> ("error out"=w1983:errorcluster, "resp"=w1978:string, "Device out"=w1981:refnum<class "Channel.lvclass">)  [unwired: 7 in]
          n713 = Fract/Exp String To Number(string=w1978) -> (number=w1976:dbl)  [unwired: 3 in, 1 out]
          n714 = Unbundle By Name(w1981) -> ("Interface.lvclass"=w1980:refnum<class "Interface.lvclass">)
          n715 = call "Read Camera Setup.vi"("Interface in"=w1980) -> ("Camera Setup"=w1979:T4)  [unwired: 8 in, 2 out]
          n716 = Unbundle By Name(w1979) -> ("EM_MODE"=w1975:u8)
          n717 = Equal?(x=w1975, y=w1976) -> (x = y?=w1977:bool)
          n718 = case shown="True" w1977 {
            tunnel: [w1987 w1988] -> w1984
            tunnel: w1982 -> [w1987 w1989]
            frame False {
            }
            frame True {
              n719 = Increment(x=w1989) -> (x+1=w1988:i32)
            }
          }
        }
        frame 232 {
          n720 = Unbundle By Name(w1998) -> ("Interface.lvclass"=w1997:refnum<class "Interface.lvclass">)
          n721 = call "Read Camera Setup.vi"("Interface in"=w1997) -> ("Camera Setup"=w1991:T4)  [unwired: 8 in, 2 out]
          n722 = Unbundle By Name(w1991) -> ("EM_GAIN"=w1990:u16)
          n723 = Number To Fractional String(number=w1990) -> (F-format string=w1992:string)  [unwired: 3 in]
          n724 = Concatenate Strings("SET EM_GAIN " ("cmd"), w1992) -> (w1996:string)
          n725 = call-dynamic "Write cmd.vi"("error in (no error)"=w2000, "cmd"=w1996, "Device in"=w1998) -> ("error out"=w1999:errorcluster, "Device out"=w2001:refnum<class "Channel.lvclass">)  [unwired: 7 in]
          n726 = Increment(x=w1994) -> (x+1=w1995:i32)
        }
        frame 233 {
          n727 = call-dynamic "Read resp.vi"("error in (no error)"=w2009, "Device in"=w2010) -> ("error out"=w2003:errorcluster, "resp"=w2008:string, "Device out"=w2004:refnum<class "Channel.lvclass">)  [unwired: 7 in]
          n728 = Equal?(x=w2008, y="DONE") -> (x = y?=w2006:bool)
          n729 = case shown="True" w2006 {
            tunnel: [w2011 w2012] -> w2005
            tunnel: w2002 -> [w2011 w2013]
            frame False {
            }
            frame True {
              n730 = Increment(x=w2013) -> (x+1=w2012:i32)
            }
          }
        }
        frame 234 {
          n731 = call-dynamic "Write cmd.vi"("error in (no error)"=w2019, "cmd"="GET EM_GAIN", "Device in"=w2017) -> ("error out"=w2018:errorcluster, "Device out"=w2020:refnum<class "Channel.lvclass">)  [unwired: 7 in]
          n732 = Increment(x=w2015) -> (x+1=w2016:i32)
        }
        frame 235 {
          n733 = call-dynamic "Read resp.vi"("error in (no error)"=w2031, "Device in"=w2032) -> ("error out"=w2029:errorcluster, "resp"=w2024:string, "Device out"=w2027:refnum<class "Channel.lvclass">)  [unwired: 7 in]
          n734 = Fract/Exp String To Number(string=w2024) -> (number=w2022:dbl)  [unwired: 3 in, 1 out]
          n735 = Unbundle By Name(w2027) -> ("Interface.lvclass"=w2026:refnum<class "Interface.lvclass">)
          n736 = call "Read Camera Setup.vi"("Interface in"=w2026) -> ("Camera Setup"=w2025:T4)  [unwired: 8 in, 2 out]
          n737 = Unbundle By Name(w2025) -> ("EM_GAIN"=w2021:u16)
          n738 = Equal?(x=w2021, y=w2022) -> (x = y?=w2023:bool)
          n739 = disable-structure shown="Enabled" {
            disable-tunnel: [w2035 264 ("State")] -> w2030
            disable-tunnel: w2028 -> [w2034 _]
            disable-tunnel: w2023 -> [w2033 _]
            frame Disabled {
              n740 = case shown="True" w2033 {
                tunnel: [w2036 w2037] -> w2035
                tunnel: w2034 -> [w2036 w2038]
                frame False {
                }
                frame True {
                  n741 = Increment(x=w2038) -> (x+1=w2037:i32)
                }
              }
            }
            frame Enabled {
            }
          }
        }
        frame 236 {
          n742 = Unbundle By Name(w2048) -> ("Interface.lvclass"=w2047:refnum<class "Interface.lvclass">)
          n743 = call "Read Camera Setup.vi"("Interface in"=w2047) -> ("Camera Setup"=w2041:T4)  [unwired: 8 in, 2 out]
          n744 = Unbundle By Name(w2041) -> ("ACQUISITION_MODE"=w2040:u8)
          n745 = Number To Fractional String(number=w2040) -> (F-format string=w2042:string)  [unwired: 3 in]
          n746 = Concatenate Strings("SET ACQUISITION_MODE " ("cmd"), w2042) -> (w2046:string)
          n747 = call-dynamic "Write cmd.vi"("error in (no error)"=w2050, "cmd"=w2046, "Device in"=w2048) -> ("error out"=w2049:errorcluster, "Device out"=w2051:refnum<class "Channel.lvclass">)  [unwired: 7 in]
          n748 = Increment(x=w2044) -> (x+1=w2045:i32)
        }
        frame 237 {
          n749 = call-dynamic "Read resp.vi"("error in (no error)"=w2059, "Device in"=w2060) -> ("error out"=w2053:errorcluster, "resp"=w2058:string, "Device out"=w2054:refnum<class "Channel.lvclass">)  [unwired: 7 in]
          n750 = Equal?(x=w2058, y="DONE") -> (x = y?=w2056:bool)
          n751 = case shown="True" w2056 {
            tunnel: [w2061 w2062] -> w2055
            tunnel: w2052 -> [w2061 w2063]
            frame False {
            }
            frame True {
              n752 = Increment(x=w2063) -> (x+1=w2062:i32)
            }
          }
        }
        frame 238 {
          n753 = call-dynamic "Write cmd.vi"("error in (no error)"=w2069, "cmd"="GET ACQUISITION_MODE", "Device in"=w2067) -> ("error out"=w2068:errorcluster, "Device out"=w2070:refnum<class "Channel.lvclass">)  [unwired: 7 in]
          n754 = Increment(x=w2065) -> (x+1=w2066:i32)
        }
        frame 239 {
          n755 = call-dynamic "Read resp.vi"("error in (no error)"=w2081, "Device in"=w2082) -> ("error out"=w2079:errorcluster, "resp"=w2074:string, "Device out"=w2077:refnum<class "Channel.lvclass">)  [unwired: 7 in]
          n756 = Fract/Exp String To Number(string=w2074) -> (number=w2072:dbl)  [unwired: 3 in, 1 out]
          n757 = Unbundle By Name(w2077) -> ("Interface.lvclass"=w2076:refnum<class "Interface.lvclass">)
          n758 = call "Read Camera Setup.vi"("Interface in"=w2076) -> ("Camera Setup"=w2075:T4)  [unwired: 8 in, 2 out]
          n759 = Unbundle By Name(w2075) -> ("ACQUISITION_MODE"=w2071:u8)
          n760 = Equal?(x=w2071, y=w2072) -> (x = y?=w2073:bool)
          n761 = case shown="True" w2073 {
            tunnel: [w2083 w2084] -> w2080
            tunnel: w2078 -> [w2083 w2085]
            frame False {
            }
            frame True {
              n762 = Increment(x=w2085) -> (x+1=w2084:i32)
            }
          }
        }
        frame 240 {
          n763 = Unbundle By Name(w2094) -> ("Interface.lvclass"=w2093:refnum<class "Interface.lvclass">)
          n764 = call "Read Camera Setup.vi"("Interface in"=w2093) -> ("Camera Setup"=w2087:T4)  [unwired: 8 in, 2 out]
          n765 = Unbundle By Name(w2087) -> ("SHUTTER_MODE"=w2086:u8)
          n766 = Number To Fractional String(number=w2086) -> (F-format string=w2088:string)  [unwired: 3 in]
          n767 = Concatenate Strings("SET SHUTTER_MODE " ("cmd"), w2088) -> (w2092:string)
          n768 = call-dynamic "Write cmd.vi"("error in (no error)"=w2096, "cmd"=w2092, "Device in"=w2094) -> ("error out"=w2095:errorcluster, "Device out"=w2097:refnum<class "Channel.lvclass">)  [unwired: 7 in]
          n769 = Increment(x=w2090) -> (x+1=w2091:i32)
        }
        frame 241 {
          n770 = call-dynamic "Read resp.vi"("error in (no error)"=w2105, "Device in"=w2106) -> ("error out"=w2099:errorcluster, "resp"=w2104:string, "Device out"=w2100:refnum<class "Channel.lvclass">)  [unwired: 7 in]
          n771 = Equal?(x=w2104, y="DONE") -> (x = y?=w2102:bool)
          n772 = case shown="True" w2102 {
            tunnel: [w2107 w2108] -> w2101
            tunnel: w2098 -> [w2107 w2109]
            frame False {
            }
            frame True {
              n773 = Increment(x=w2109) -> (x+1=w2108:i32)
            }
          }
        }
        frame 242 {
          n774 = call-dynamic "Write cmd.vi"("error in (no error)"=w2115, "cmd"="GET SHUTTER_MODE", "Device in"=w2113) -> ("error out"=w2114:errorcluster, "Device out"=w2116:refnum<class "Channel.lvclass">)  [unwired: 7 in]
          n775 = Increment(x=w2111) -> (x+1=w2112:i32)
        }
        frame 243 {
          n776 = call-dynamic "Read resp.vi"("error in (no error)"=w2127, "Device in"=w2128) -> ("error out"=w2125:errorcluster, "resp"=w2120:string, "Device out"=w2123:refnum<class "Channel.lvclass">)  [unwired: 7 in]
          n777 = Fract/Exp String To Number(string=w2120) -> (number=w2118:dbl)  [unwired: 3 in, 1 out]
          n778 = Unbundle By Name(w2123) -> ("Interface.lvclass"=w2122:refnum<class "Interface.lvclass">)
          n779 = call "Read Camera Setup.vi"("Interface in"=w2122) -> ("Camera Setup"=w2121:T4)  [unwired: 8 in, 2 out]
          n780 = Unbundle By Name(w2121) -> ("SHUTTER_MODE"=w2117:u8)
          n781 = Equal?(x=w2117, y=w2118) -> (x = y?=w2119:bool)
          n782 = case shown="True" w2119 {
            tunnel: [w2129 w2130] -> w2126
            tunnel: w2124 -> [w2129 w2131]
            frame False {
            }
            frame True {
              n783 = Increment(x=w2131) -> (x+1=w2130:i32)
            }
          }
        }
        frame 244 {
          n784 = Unbundle By Name(w2140) -> ("Interface.lvclass"=w2139:refnum<class "Interface.lvclass">)
          n785 = call "Read Camera Setup.vi"("Interface in"=w2139) -> ("Camera Setup"=w2133:T4)  [unwired: 8 in, 2 out]
          n786 = Unbundle By Name(w2133) -> ("SHUTTER_TTL"=w2132:u8)
          n787 = Number To Fractional String(number=w2132) -> (F-format string=w2134:string)  [unwired: 3 in]
          n788 = Concatenate Strings("SET SHUTTER_TTL " ("cmd"), w2134) -> (w2138:string)
          n789 = call-dynamic "Write cmd.vi"("error in (no error)"=w2142, "cmd"=w2138, "Device in"=w2140) -> ("error out"=w2141:errorcluster, "Device out"=w2143:refnum<class "Channel.lvclass">)  [unwired: 7 in]
          n790 = Increment(x=w2136) -> (x+1=w2137:i32)
        }
        frame 245 {
          n791 = call-dynamic "Read resp.vi"("error in (no error)"=w2151, "Device in"=w2152) -> ("error out"=w2145:errorcluster, "resp"=w2150:string, "Device out"=w2146:refnum<class "Channel.lvclass">)  [unwired: 7 in]
          n792 = Equal?(x=w2150, y="DONE") -> (x = y?=w2148:bool)
          n793 = case shown="True" w2148 {
            tunnel: [w2153 w2154] -> w2147
            tunnel: w2144 -> [w2153 w2155]
            frame False {
            }
            frame True {
              n794 = Increment(x=w2155) -> (x+1=w2154:i32)
            }
          }
        }
        frame 246 {
          n795 = call-dynamic "Write cmd.vi"("error in (no error)"=w2161, "cmd"="GET SHUTTER_TTL", "Device in"=w2159) -> ("error out"=w2160:errorcluster, "Device out"=w2162:refnum<class "Channel.lvclass">)  [unwired: 7 in]
          n796 = Increment(x=w2157) -> (x+1=w2158:i32)
        }
        frame 247 {
          n797 = call-dynamic "Read resp.vi"("error in (no error)"=w2173, "Device in"=w2174) -> ("error out"=w2171:errorcluster, "resp"=w2166:string, "Device out"=w2169:refnum<class "Channel.lvclass">)  [unwired: 7 in]
          n798 = Fract/Exp String To Number(string=w2166) -> (number=w2164:dbl)  [unwired: 3 in, 1 out]
          n799 = Unbundle By Name(w2169) -> ("Interface.lvclass"=w2168:refnum<class "Interface.lvclass">)
          n800 = call "Read Camera Setup.vi"("Interface in"=w2168) -> ("Camera Setup"=w2167:T4)  [unwired: 8 in, 2 out]
          n801 = Unbundle By Name(w2167) -> ("SHUTTER_TTL"=w2163:u8)
          n802 = Equal?(x=w2163, y=w2164) -> (x = y?=w2165:bool)
          n803 = case shown="True" w2165 {
            tunnel: [w2175 w2176] -> w2172
            tunnel: w2170 -> [w2175 w2177]
            frame False {
            }
            frame True {
              n804 = Increment(x=w2177) -> (x+1=w2176:i32)
            }
          }
        }
        frame 248 {
          n805 = Unbundle By Name(w2186) -> ("Interface.lvclass"=w2185:refnum<class "Interface.lvclass">)
          n806 = call "Read Camera Setup.vi"("Interface in"=w2185) -> ("Camera Setup"=w2179:T4)  [unwired: 8 in, 2 out]
          n807 = Unbundle By Name(w2179) -> ("SHUTTER_OPENNING_TIME"=w2178:u16)
          n808 = Number To Fractional String(number=w2178) -> (F-format string=w2180:string)  [unwired: 3 in]
          n809 = Concatenate Strings("SET SHUTTER_OPENNING_TIME " ("cmd"), w2180) -> (w2184:string)
          n810 = call-dynamic "Write cmd.vi"("error in (no error)"=w2188, "cmd"=w2184, "Device in"=w2186) -> ("error out"=w2187:errorcluster, "Device out"=w2189:refnum<class "Channel.lvclass">)  [unwired: 7 in]
          n811 = Increment(x=w2182) -> (x+1=w2183:i32)
        }
        frame 249 {
          n812 = call-dynamic "Read resp.vi"("error in (no error)"=w2197, "Device in"=w2198) -> ("error out"=w2191:errorcluster, "resp"=w2196:string, "Device out"=w2192:refnum<class "Channel.lvclass">)  [unwired: 7 in]
          n813 = Equal?(x=w2196, y="DONE") -> (x = y?=w2194:bool)
          n814 = case shown="True" w2194 {
            tunnel: [w2199 w2200] -> w2193
            tunnel: w2190 -> [w2199 w2201]
            frame False {
            }
            frame True {
              n815 = Increment(x=w2201) -> (x+1=w2200:i32)
            }
          }
        }
        frame 250 {
          n816 = call-dynamic "Write cmd.vi"("error in (no error)"=w2207, "cmd"="GET SHUTTER_OPENNING_TIME", "Device in"=w2205) -> ("error out"=w2206:errorcluster, "Device out"=w2208:refnum<class "Channel.lvclass">)  [unwired: 7 in]
          n817 = Increment(x=w2203) -> (x+1=w2204:i32)
        }
        frame 251 {
          n818 = call-dynamic "Read resp.vi"("error in (no error)"=w2219, "Device in"=w2220) -> ("error out"=w2217:errorcluster, "resp"=w2212:string, "Device out"=w2215:refnum<class "Channel.lvclass">)  [unwired: 7 in]
          n819 = Fract/Exp String To Number(string=w2212) -> (number=w2210:dbl)  [unwired: 3 in, 1 out]
          n820 = Unbundle By Name(w2215) -> ("Interface.lvclass"=w2214:refnum<class "Interface.lvclass">)
          n821 = call "Read Camera Setup.vi"("Interface in"=w2214) -> ("Camera Setup"=w2213:T4)  [unwired: 8 in, 2 out]
          n822 = Unbundle By Name(w2213) -> ("SHUTTER_OPENNING_TIME"=w2209:u16)
          n823 = Equal?(x=w2209, y=w2210) -> (x = y?=w2211:bool)
          n824 = case shown="True" w2211 {
            tunnel: [w2221 w2222] -> w2218
            tunnel: w2216 -> [w2221 w2223]
            frame False {
            }
            frame True {
              n825 = Increment(x=w2223) -> (x+1=w2222:i32)
            }
          }
        }
        frame 252 {
          n826 = Unbundle By Name(w2232) -> ("Interface.lvclass"=w2231:refnum<class "Interface.lvclass">)
          n827 = call "Read Camera Setup.vi"("Interface in"=w2231) -> ("Camera Setup"=w2225:T4)  [unwired: 8 in, 2 out]
          n828 = Unbundle By Name(w2225) -> ("SHUTTER_CLOSING_TIME"=w2224:u16)
          n829 = Number To Fractional String(number=w2224) -> (F-format string=w2226:string)  [unwired: 3 in]
          n830 = Concatenate Strings("SET SHUTTER_CLOSING_TIME " ("cmd"), w2226) -> (w2230:string)
          n831 = call-dynamic "Write cmd.vi"("error in (no error)"=w2234, "cmd"=w2230, "Device in"=w2232) -> ("error out"=w2233:errorcluster, "Device out"=w2235:refnum<class "Channel.lvclass">)  [unwired: 7 in]
          n832 = Increment(x=w2228) -> (x+1=w2229:i32)
        }
        frame 253 {
          n833 = call-dynamic "Read resp.vi"("error in (no error)"=w2243, "Device in"=w2244) -> ("error out"=w2237:errorcluster, "resp"=w2242:string, "Device out"=w2238:refnum<class "Channel.lvclass">)  [unwired: 7 in]
          n834 = Equal?(x=w2242, y="DONE") -> (x = y?=w2240:bool)
          n835 = case shown="True" w2240 {
            tunnel: [w2245 w2246] -> w2239
            tunnel: w2236 -> [w2245 w2247]
            frame False {
            }
            frame True {
              n836 = Increment(x=w2247) -> (x+1=w2246:i32)
            }
          }
        }
        frame 254 {
          n837 = call-dynamic "Write cmd.vi"("error in (no error)"=w2253, "cmd"="GET SHUTTER_CLOSING_TIME", "Device in"=w2251) -> ("error out"=w2252:errorcluster, "Device out"=w2254:refnum<class "Channel.lvclass">)  [unwired: 7 in]
          n838 = Increment(x=w2249) -> (x+1=w2250:i32)
        }
        frame 255 {
          n839 = call-dynamic "Read resp.vi"("error in (no error)"=w2265, "Device in"=w2266) -> ("error out"=w2263:errorcluster, "resp"=w2258:string, "Device out"=w2261:refnum<class "Channel.lvclass">)  [unwired: 7 in]
          n840 = Fract/Exp String To Number(string=w2258) -> (number=w2256:dbl)  [unwired: 3 in, 1 out]
          n841 = Unbundle By Name(w2261) -> ("Interface.lvclass"=w2260:refnum<class "Interface.lvclass">)
          n842 = call "Read Camera Setup.vi"("Interface in"=w2260) -> ("Camera Setup"=w2259:T4)  [unwired: 8 in, 2 out]
          n843 = Unbundle By Name(w2259) -> ("SHUTTER_CLOSING_TIME"=w2255:u16)
          n844 = Equal?(x=w2255, y=w2256) -> (x = y?=w2257:bool)
          n845 = case shown="True" w2257 {
            tunnel: [w2267 w2268] -> w2264
            tunnel: w2262 -> [w2267 w2269]
            frame False {
            }
            frame True {
              n846 = Increment(x=w2269) -> (x+1=w2268:i32)
            }
          }
        }
        frame 256 {
          n847 = Unbundle By Name(w2278) -> ("Interface.lvclass"=w2277:refnum<class "Interface.lvclass">)
          n848 = call "Read Camera Setup.vi"("Interface in"=w2277) -> ("Camera Setup"=w2271:T4)  [unwired: 8 in, 2 out]
          n849 = Unbundle By Name(w2271) -> ("HBIN"=w2270:u16)
          n850 = Number To Fractional String(number=w2270) -> (F-format string=w2272:string)  [unwired: 3 in]
          n851 = Concatenate Strings("SET HBIN " ("cmd"), w2272) -> (w2276:string)
          n852 = call-dynamic "Write cmd.vi"("error in (no error)"=w2280, "cmd"=w2276, "Device in"=w2278) -> ("error out"=w2279:errorcluster, "Device out"=w2281:refnum<class "Channel.lvclass">)  [unwired: 7 in]
          n853 = Increment(x=w2274) -> (x+1=w2275:i32)
        }
        frame 257 {
          n854 = call-dynamic "Read resp.vi"("error in (no error)"=w2289, "Device in"=w2290) -> ("error out"=w2283:errorcluster, "resp"=w2288:string, "Device out"=w2284:refnum<class "Channel.lvclass">)  [unwired: 7 in]
          n855 = Equal?(x=w2288, y="DONE") -> (x = y?=w2286:bool)
          n856 = case shown="True" w2286 {
            tunnel: [w2291 w2292] -> w2285
            tunnel: w2282 -> [w2291 w2293]
            frame False {
            }
            frame True {
              n857 = Increment(x=w2293) -> (x+1=w2292:i32)
            }
          }
        }
        frame 258 {
          n858 = call-dynamic "Write cmd.vi"("error in (no error)"=w2299, "cmd"="GET HBIN", "Device in"=w2297) -> ("error out"=w2298:errorcluster, "Device out"=w2300:refnum<class "Channel.lvclass">)  [unwired: 7 in]
          n859 = Increment(x=w2295) -> (x+1=w2296:i32)
        }
        frame 259 {
          n860 = call-dynamic "Read resp.vi"("error in (no error)"=w2311, "Device in"=w2312) -> ("error out"=w2309:errorcluster, "resp"=w2304:string, "Device out"=w2307:refnum<class "Channel.lvclass">)  [unwired: 7 in]
          n861 = Fract/Exp String To Number(string=w2304) -> (number=w2302:dbl)  [unwired: 3 in, 1 out]
          n862 = Unbundle By Name(w2307) -> ("Interface.lvclass"=w2306:refnum<class "Interface.lvclass">)
          n863 = call "Read Camera Setup.vi"("Interface in"=w2306) -> ("Camera Setup"=w2305:T4)  [unwired: 8 in, 2 out]
          n864 = Unbundle By Name(w2305) -> ("HBIN"=w2301:u16)
          n865 = Equal?(x=w2301, y=w2302) -> (x = y?=w2303:bool)
          n866 = case shown="True" w2303 {
            tunnel: [w2313 w2314] -> w2310
            tunnel: w2308 -> [w2313 w2315]
            frame False {
            }
            frame True {
              n867 = Increment(x=w2315) -> (x+1=w2314:i32)
            }
          }
        }
        frame 260 {
          n868 = Unbundle By Name(w2324) -> ("Interface.lvclass"=w2323:refnum<class "Interface.lvclass">)
          n869 = call "Read Camera Setup.vi"("Interface in"=w2323) -> ("Camera Setup"=w2317:T4)  [unwired: 8 in, 2 out]
          n870 = Unbundle By Name(w2317) -> ("VBIN"=w2316:u16)
          n871 = Number To Fractional String(number=w2316) -> (F-format string=w2318:string)  [unwired: 3 in]
          n872 = Concatenate Strings("SET VBIN " ("cmd"), w2318) -> (w2322:string)
          n873 = call-dynamic "Write cmd.vi"("error in (no error)"=w2326, "cmd"=w2322, "Device in"=w2324) -> ("error out"=w2325:errorcluster, "Device out"=w2327:refnum<class "Channel.lvclass">)  [unwired: 7 in]
          n874 = Increment(x=w2320) -> (x+1=w2321:i32)
        }
        frame 261 {
          n875 = call-dynamic "Read resp.vi"("error in (no error)"=w2335, "Device in"=w2336) -> ("error out"=w2329:errorcluster, "resp"=w2334:string, "Device out"=w2330:refnum<class "Channel.lvclass">)  [unwired: 7 in]
          n876 = Equal?(x=w2334, y="DONE") -> (x = y?=w2332:bool)
          n877 = case shown="True" w2332 {
            tunnel: [w2337 w2338] -> w2331
            tunnel: w2328 -> [w2337 w2339]
            frame False {
            }
            frame True {
              n878 = Increment(x=w2339) -> (x+1=w2338:i32)
            }
          }
        }
        frame 262 {
          n879 = call-dynamic "Write cmd.vi"("error in (no error)"=w2345, "cmd"="GET VBIN", "Device in"=w2343) -> ("error out"=w2344:errorcluster, "Device out"=w2346:refnum<class "Channel.lvclass">)  [unwired: 7 in]
          n880 = Increment(x=w2341) -> (x+1=w2342:i32)
        }
        frame 263 {
          n881 = call-dynamic "Read resp.vi"("error in (no error)"=w2357, "Device in"=w2358) -> ("error out"=w2355:errorcluster, "resp"=w2350:string, "Device out"=w2353:refnum<class "Channel.lvclass">)  [unwired: 7 in]
          n882 = Fract/Exp String To Number(string=w2350) -> (number=w2348:dbl)  [unwired: 3 in, 1 out]
          n883 = Unbundle By Name(w2353) -> ("Interface.lvclass"=w2352:refnum<class "Interface.lvclass">)
          n884 = call "Read Camera Setup.vi"("Interface in"=w2352) -> ("Camera Setup"=w2351:T4)  [unwired: 8 in, 2 out]
          n885 = Unbundle By Name(w2351) -> ("VBIN"=w2347:u16)
          n886 = Equal?(x=w2347, y=w2348) -> (x = y?=w2349:bool)
          n887 = case shown="True" w2349 {
            tunnel: [w2359 w2360] -> w2356
            tunnel: w2354 -> [w2359 w2361]
            frame False {
            }
            frame True {
              n888 = Increment(x=w2361) -> (x+1=w2360:i32)
            }
          }
        }
        frame 264 {
          n889 = Unbundle By Name(w2370) -> ("Interface.lvclass"=w2369:refnum<class "Interface.lvclass">)
          n890 = call "Read Camera Setup.vi"("Interface in"=w2369) -> ("Camera Setup"=w2363:T4)  [unwired: 8 in, 2 out]
          n891 = Unbundle By Name(w2363) -> ("INITIAL_LINE"=w2362:u16)
          n892 = Number To Fractional String(number=w2362) -> (F-format string=w2364:string)  [unwired: 3 in]
          n893 = Concatenate Strings("SET INITIAL_LINE " ("cmd"), w2364) -> (w2368:string)
          n894 = call-dynamic "Write cmd.vi"("error in (no error)"=w2372, "cmd"=w2368, "Device in"=w2370) -> ("error out"=w2371:errorcluster, "Device out"=w2373:refnum<class "Channel.lvclass">)  [unwired: 7 in]
          n895 = Increment(x=w2366) -> (x+1=w2367:i32)
        }
        frame 265 {
          n896 = call-dynamic "Read resp.vi"("error in (no error)"=w2381, "Device in"=w2382) -> ("error out"=w2375:errorcluster, "resp"=w2380:string, "Device out"=w2376:refnum<class "Channel.lvclass">)  [unwired: 7 in]
          n897 = Equal?(x=w2380, y="DONE") -> (x = y?=w2378:bool)
          n898 = case shown="True" w2378 {
            tunnel: [w2383 w2384] -> w2377
            tunnel: w2374 -> [w2383 w2385]
            frame False {
            }
            frame True {
              n899 = Increment(x=w2385) -> (x+1=w2384:i32)
            }
          }
        }
        frame 266 {
          n900 = call-dynamic "Write cmd.vi"("error in (no error)"=w2391, "cmd"="GET INITIAL_LINE", "Device in"=w2389) -> ("error out"=w2390:errorcluster, "Device out"=w2392:refnum<class "Channel.lvclass">)  [unwired: 7 in]
          n901 = Increment(x=w2387) -> (x+1=w2388:i32)
        }
        frame 267 {
          n902 = call-dynamic "Read resp.vi"("error in (no error)"=w2403, "Device in"=w2404) -> ("error out"=w2401:errorcluster, "resp"=w2396:string, "Device out"=w2399:refnum<class "Channel.lvclass">)  [unwired: 7 in]
          n903 = Fract/Exp String To Number(string=w2396) -> (number=w2394:dbl)  [unwired: 3 in, 1 out]
          n904 = Unbundle By Name(w2399) -> ("Interface.lvclass"=w2398:refnum<class "Interface.lvclass">)
          n905 = call "Read Camera Setup.vi"("Interface in"=w2398) -> ("Camera Setup"=w2397:T4)  [unwired: 8 in, 2 out]
          n906 = Unbundle By Name(w2397) -> ("INITIAL_LINE"=w2393:u16)
          n907 = Equal?(x=w2393, y=w2394) -> (x = y?=w2395:bool)
          n908 = case shown="True" w2395 {
            tunnel: [w2405 w2406] -> w2402
            tunnel: w2400 -> [w2405 w2407]
            frame False {
            }
            frame True {
              n909 = Increment(x=w2407) -> (x+1=w2406:i32)
            }
          }
        }
        frame 268 {
          n910 = Unbundle By Name(w2416) -> ("Interface.lvclass"=w2415:refnum<class "Interface.lvclass">)
          n911 = call "Read Camera Setup.vi"("Interface in"=w2415) -> ("Camera Setup"=w2409:T4)  [unwired: 8 in, 2 out]
          n912 = Unbundle By Name(w2409) -> ("INITIAL_COLUMN"=w2408:u16)
          n913 = Number To Fractional String(number=w2408) -> (F-format string=w2410:string)  [unwired: 3 in]
          n914 = Concatenate Strings("SET INITIAL_COLUMN " ("cmd"), w2410) -> (w2414:string)
          n915 = call-dynamic "Write cmd.vi"("error in (no error)"=w2418, "cmd"=w2414, "Device in"=w2416) -> ("error out"=w2417:errorcluster, "Device out"=w2419:refnum<class "Channel.lvclass">)  [unwired: 7 in]
          n916 = Increment(x=w2412) -> (x+1=w2413:i32)
        }
        frame 269 {
          n917 = call-dynamic "Read resp.vi"("error in (no error)"=w2427, "Device in"=w2428) -> ("error out"=w2421:errorcluster, "resp"=w2426:string, "Device out"=w2422:refnum<class "Channel.lvclass">)  [unwired: 7 in]
          n918 = Equal?(x=w2426, y="DONE") -> (x = y?=w2424:bool)
          n919 = case shown="True" w2424 {
            tunnel: [w2429 w2430] -> w2423
            tunnel: w2420 -> [w2429 w2431]
            frame False {
            }
            frame True {
              n920 = Increment(x=w2431) -> (x+1=w2430:i32)
            }
          }
        }
        frame 270 {
          n921 = call-dynamic "Write cmd.vi"("error in (no error)"=w2437, "cmd"="GET INITIAL_COLUMN", "Device in"=w2435) -> ("error out"=w2436:errorcluster, "Device out"=w2438:refnum<class "Channel.lvclass">)  [unwired: 7 in]
          n922 = Increment(x=w2433) -> (x+1=w2434:i32)
        }
        frame 271 {
          n923 = call-dynamic "Read resp.vi"("error in (no error)"=w2449, "Device in"=w2450) -> ("error out"=w2447:errorcluster, "resp"=w2442:string, "Device out"=w2445:refnum<class "Channel.lvclass">)  [unwired: 7 in]
          n924 = Fract/Exp String To Number(string=w2442) -> (number=w2440:dbl)  [unwired: 3 in, 1 out]
          n925 = Unbundle By Name(w2445) -> ("Interface.lvclass"=w2444:refnum<class "Interface.lvclass">)
          n926 = call "Read Camera Setup.vi"("Interface in"=w2444) -> ("Camera Setup"=w2443:T4)  [unwired: 8 in, 2 out]
          n927 = Unbundle By Name(w2443) -> ("INITIAL_COLUMN"=w2439:u16)
          n928 = Equal?(x=w2439, y=w2440) -> (x = y?=w2441:bool)
          n929 = case shown="True" w2441 {
            tunnel: [w2451 w2452] -> w2448
            tunnel: w2446 -> [w2451 w2453]
            frame False {
            }
            frame True {
              n930 = Increment(x=w2453) -> (x+1=w2452:i32)
            }
          }
        }
        frame 272 {
          n931 = Unbundle By Name(w2462) -> ("Interface.lvclass"=w2461:refnum<class "Interface.lvclass">)
          n932 = call "Read Camera Setup.vi"("Interface in"=w2461) -> ("Camera Setup"=w2455:T4)  [unwired: 8 in, 2 out]
          n933 = Unbundle By Name(w2455) -> ("FINAL_LINE"=w2454:u16)
          n934 = Number To Fractional String(number=w2454) -> (F-format string=w2456:string)  [unwired: 3 in]
          n935 = Concatenate Strings("SET FINAL_LINE " ("cmd"), w2456) -> (w2460:string)
          n936 = call-dynamic "Write cmd.vi"("error in (no error)"=w2464, "cmd"=w2460, "Device in"=w2462) -> ("error out"=w2463:errorcluster, "Device out"=w2465:refnum<class "Channel.lvclass">)  [unwired: 7 in]
          n937 = Increment(x=w2458) -> (x+1=w2459:i32)
        }
        frame 273 {
          n938 = call-dynamic "Read resp.vi"("error in (no error)"=w2473, "Device in"=w2474) -> ("error out"=w2467:errorcluster, "resp"=w2472:string, "Device out"=w2468:refnum<class "Channel.lvclass">)  [unwired: 7 in]
          n939 = Equal?(x=w2472, y="DONE") -> (x = y?=w2470:bool)
          n940 = case shown="True" w2470 {
            tunnel: [w2475 w2476] -> w2469
            tunnel: w2466 -> [w2475 w2477]
            frame False {
            }
            frame True {
              n941 = Increment(x=w2477) -> (x+1=w2476:i32)
            }
          }
        }
        frame 274 {
          n942 = call-dynamic "Write cmd.vi"("error in (no error)"=w2483, "cmd"="GET FINAL_LINE", "Device in"=w2481) -> ("error out"=w2482:errorcluster, "Device out"=w2484:refnum<class "Channel.lvclass">)  [unwired: 7 in]
          n943 = Increment(x=w2479) -> (x+1=w2480:i32)
        }
        frame 275 {
          n944 = call-dynamic "Read resp.vi"("error in (no error)"=w2495, "Device in"=w2496) -> ("error out"=w2493:errorcluster, "resp"=w2488:string, "Device out"=w2491:refnum<class "Channel.lvclass">)  [unwired: 7 in]
          n945 = Fract/Exp String To Number(string=w2488) -> (number=w2486:dbl)  [unwired: 3 in, 1 out]
          n946 = Unbundle By Name(w2491) -> ("Interface.lvclass"=w2490:refnum<class "Interface.lvclass">)
          n947 = call "Read Camera Setup.vi"("Interface in"=w2490) -> ("Camera Setup"=w2489:T4)  [unwired: 8 in, 2 out]
          n948 = Unbundle By Name(w2489) -> ("FINAL_LINE"=w2485:u16)
          n949 = Equal?(x=w2485, y=w2486) -> (x = y?=w2487:bool)
          n950 = case shown="True" w2487 {
            tunnel: [w2497 w2498] -> w2494
            tunnel: w2492 -> [w2497 w2499]
            frame False {
            }
            frame True {
              n951 = Increment(x=w2499) -> (x+1=w2498:i32)
            }
          }
        }
        frame 276 {
          n952 = Unbundle By Name(w2508) -> ("Interface.lvclass"=w2507:refnum<class "Interface.lvclass">)
          n953 = call "Read Camera Setup.vi"("Interface in"=w2507) -> ("Camera Setup"=w2501:T4)  [unwired: 8 in, 2 out]
          n954 = Unbundle By Name(w2501) -> ("FINAL_COLUMN"=w2500:u16)
          n955 = Number To Fractional String(number=w2500) -> (F-format string=w2502:string)  [unwired: 3 in]
          n956 = Concatenate Strings("SET FINAL_COLUMN " ("cmd"), w2502) -> (w2506:string)
          n957 = call-dynamic "Write cmd.vi"("error in (no error)"=w2510, "cmd"=w2506, "Device in"=w2508) -> ("error out"=w2509:errorcluster, "Device out"=w2511:refnum<class "Channel.lvclass">)  [unwired: 7 in]
          n958 = Increment(x=w2504) -> (x+1=w2505:i32)
        }
        frame 277 {
          n959 = call-dynamic "Read resp.vi"("error in (no error)"=w2519, "Device in"=w2520) -> ("error out"=w2513:errorcluster, "resp"=w2518:string, "Device out"=w2514:refnum<class "Channel.lvclass">)  [unwired: 7 in]
          n960 = Equal?(x=w2518, y="DONE") -> (x = y?=w2516:bool)
          n961 = case shown="True" w2516 {
            tunnel: [w2521 w2522] -> w2515
            tunnel: w2512 -> [w2521 w2523]
            frame False {
            }
            frame True {
              n962 = Increment(x=w2523) -> (x+1=w2522:i32)
            }
          }
        }
        frame 278 {
          n963 = call-dynamic "Write cmd.vi"("error in (no error)"=w2529, "cmd"="GET FINAL_COLUMN", "Device in"=w2527) -> ("error out"=w2528:errorcluster, "Device out"=w2530:refnum<class "Channel.lvclass">)  [unwired: 7 in]
          n964 = Increment(x=w2525) -> (x+1=w2526:i32)
        }
        frame 279 {
          n965 = call-dynamic "Read resp.vi"("error in (no error)"=w2541, "Device in"=w2542) -> ("error out"=w2539:errorcluster, "resp"=w2534:string, "Device out"=w2537:refnum<class "Channel.lvclass">)  [unwired: 7 in]
          n966 = Fract/Exp String To Number(string=w2534) -> (number=w2532:dbl)  [unwired: 3 in, 1 out]
          n967 = Unbundle By Name(w2537) -> ("Interface.lvclass"=w2536:refnum<class "Interface.lvclass">)
          n968 = call "Read Camera Setup.vi"("Interface in"=w2536) -> ("Camera Setup"=w2535:T4)  [unwired: 8 in, 2 out]
          n969 = Unbundle By Name(w2535) -> ("FINAL_COLUMN"=w2531:u16)
          n970 = Equal?(x=w2531, y=w2532) -> (x = y?=w2533:bool)
          n971 = disable-structure shown="Enabled" {
            disable-tunnel: [w2545 0 ("State")] -> w2540
            disable-tunnel: w2538 -> [w2544 _]
            disable-tunnel: w2533 -> [w2543 _]
            frame Disabled {
              n972 = case shown="True" w2543 {
                tunnel: [w2546 w2547] -> w2545
                tunnel: w2544 -> [w2546 w2548]
                frame False {
                }
                frame True {
                  n973 = Increment(x=w2548) -> (x+1=w2547:i32)
                }
              }
            }
            frame Enabled {
            }
          }
        }
        frame 280 {
          n974 = Unbundle By Name(w2558) -> ("Interface.lvclass"=w2557:refnum<class "Interface.lvclass">)
          n975 = call "Read Camera Setup.vi"("Interface in"=w2557) -> ("Camera Setup"=w2551:T4)  [unwired: 8 in, 2 out]
          n976 = Unbundle By Name(w2551) -> ("VERTICAL_CLOCK_VOLTAGE"=w2550:u8)
          n977 = Number To Fractional String(number=w2550) -> (F-format string=w2552:string)  [unwired: 3 in]
          n978 = Concatenate Strings("SET VERTICAL_CLOCK_VOLTAGE " ("cmd"), w2552) -> (w2556:string)
          n979 = call-dynamic "Write cmd.vi"("error in (no error)"=w2560, "cmd"=w2556, "Device in"=w2558) -> ("error out"=w2559:errorcluster, "Device out"=w2561:refnum<class "Channel.lvclass">)  [unwired: 7 in]
          n980 = Increment(x=w2554) -> (x+1=w2555:i32)
        }
        frame 281 {
          n981 = call-dynamic "Read resp.vi"("error in (no error)"=w2569, "Device in"=w2570) -> ("error out"=w2563:errorcluster, "resp"=w2568:string, "Device out"=w2564:refnum<class "Channel.lvclass">)  [unwired: 7 in]
          n982 = Equal?(x=w2568, y="DONE") -> (x = y?=w2566:bool)
          n983 = case shown="True" w2566 {
            tunnel: [w2571 w2572] -> w2565
            tunnel: w2562 -> [w2571 w2573]
            frame False {
            }
            frame True {
              n984 = Increment(x=w2573) -> (x+1=w2572:i32)
            }
          }
        }
        frame 282 {
          n985 = call-dynamic "Write cmd.vi"("error in (no error)"=w2579, "cmd"="GET VERTICAL_CLOCK_VOLTAGE", "Device in"=w2577) -> ("error out"=w2578:errorcluster, "Device out"=w2580:refnum<class "Channel.lvclass">)  [unwired: 7 in]
          n986 = Increment(x=w2575) -> (x+1=w2576:i32)
        }
        frame 283 {
          n987 = call-dynamic "Read resp.vi"("error in (no error)"=w2591, "Device in"=w2592) -> ("error out"=w2589:errorcluster, "resp"=w2584:string, "Device out"=w2587:refnum<class "Channel.lvclass">)  [unwired: 7 in]
          n988 = Fract/Exp String To Number(string=w2584) -> (number=w2582:dbl)  [unwired: 3 in, 1 out]
          n989 = Unbundle By Name(w2587) -> ("Interface.lvclass"=w2586:refnum<class "Interface.lvclass">)
          n990 = call "Read Camera Setup.vi"("Interface in"=w2586) -> ("Camera Setup"=w2585:T4)  [unwired: 8 in, 2 out]
          n991 = Unbundle By Name(w2585) -> ("VERTICAL_CLOCK_VOLTAGE"=w2581:u8)
          n992 = Equal?(x=w2581, y=w2582) -> (x = y?=w2583:bool)
          n993 = case shown="True" w2583 {
            tunnel: [w2593 w2594] -> w2590
            tunnel: w2588 -> [w2593 w2595]
            frame False {
            }
            frame True {
              n994 = Increment(x=w2595) -> (x+1=w2594:i32)
            }
          }
        }
        frame 284 {
          n995 = Unbundle By Name(w2604) -> ("Interface.lvclass"=w2603:refnum<class "Interface.lvclass">)
          n996 = call "Read Camera Setup.vi"("Interface in"=w2603) -> ("Camera Setup"=w2598:T4)  [unwired: 8 in, 2 out]
          n997 = Unbundle By Name(w2598) -> ("FRAME_TRANSFER"=w2597:bool)
          n998 = case shown="True" w2597 {
            tunnel: ["T" ("cmd") "F" ("cmd")] -> w2596
            frame True {
            }
            frame False {
            }
          }
          n999 = Concatenate Strings("SET FRAME_TRANSFER " ("cmd"), w2596) -> (w2602:string)
          n1000 = call-dynamic "Write cmd.vi"("error in (no error)"=w2606, "cmd"=w2602, "Device in"=w2604) -> ("error out"=w2605:errorcluster, "Device out"=w2607:refnum<class "Channel.lvclass">)  [unwired: 7 in]
          n1001 = Increment(x=w2600) -> (x+1=w2601:i32)
        }
        frame 285 {
          n1002 = call-dynamic "Read resp.vi"("error in (no error)"=w2617, "Device in"=w2618) -> ("error out"=w2611:errorcluster, "resp"=w2616:string, "Device out"=w2612:refnum<class "Channel.lvclass">)  [unwired: 7 in]
          n1003 = Equal?(x=w2616, y="DONE") -> (x = y?=w2614:bool)
          n1004 = case shown="True" w2614 {
            tunnel: [w2619 w2620] -> w2613
            tunnel: w2610 -> [w2619 w2621]
            frame False {
            }
            frame True {
              n1005 = Increment(x=w2621) -> (x+1=w2620:i32)
            }
          }
        }
        frame 286 {
          n1006 = call-dynamic "Write cmd.vi"("error in (no error)"=w2627, "cmd"="GET FRAME_TRANSFER", "Device in"=w2625) -> ("error out"=w2626:errorcluster, "Device out"=w2628:refnum<class "Channel.lvclass">)  [unwired: 7 in]
          n1007 = Increment(x=w2623) -> (x+1=w2624:i32)
        }
        frame 287 {
          n1008 = call-dynamic "Read resp.vi"("error in (no error)"=w2639, "Device in"=w2640) -> ("error out"=w2637:errorcluster, "resp"=w2631:string, "Device out"=w2635:refnum<class "Channel.lvclass">)  [unwired: 7 in]
          n1009 = Unbundle By Name(w2635) -> ("Interface.lvclass"=w2634:refnum<class "Interface.lvclass">)
          n1010 = call "Read Camera Setup.vi"("Interface in"=w2634) -> ("Camera Setup"=w2633:T4)  [unwired: 8 in, 2 out]
          n1011 = Unbundle By Name(w2633) -> ("FRAME_TRANSFER"=w2630:bool)
          n1012 = case shown="True" w2630 {
            tunnel: ["T" "F"] -> w2629
            frame True {
            }
            frame False {
            }
          }
          n1013 = Equal?(x=w2629, y=w2631) -> (x = y?=w2632:bool)
          n1014 = case shown="True" w2632 {
            tunnel: [w2643 w2644] -> w2638
            tunnel: w2636 -> [w2643 w2645]
            frame False {
            }
            frame True {
              n1015 = Increment(x=w2645) -> (x+1=w2644:i32)
            }
          }
        }
        frame 288 {
          n1016 = Unbundle By Name(w2654) -> ("Interface.lvclass"=w2653:refnum<class "Interface.lvclass">)
          n1017 = call "Read Camera Setup.vi"("Interface in"=w2653) -> ("Camera Setup"=w2647:T4)  [unwired: 8 in, 2 out]
          n1018 = Unbundle By Name(w2647) -> ("AD_CHANNEL"=w2646:u32)
          n1019 = Number To Fractional String(number=w2646) -> (F-format string=w2648:string)  [unwired: 3 in]
          n1020 = Concatenate Strings("SET AD_CHANNEL " ("cmd"), w2648) -> (w2652:string)
          n1021 = call-dynamic "Write cmd.vi"("error in (no error)"=w2656, "cmd"=w2652, "Device in"=w2654) -> ("error out"=w2655:errorcluster, "Device out"=w2657:refnum<class "Channel.lvclass">)  [unwired: 7 in]
          n1022 = Increment(x=w2650) -> (x+1=w2651:i32)
        }
        frame 289 {
          n1023 = call-dynamic "Read resp.vi"("error in (no error)"=w2665, "Device in"=w2666) -> ("error out"=w2659:errorcluster, "resp"=w2664:string, "Device out"=w2660:refnum<class "Channel.lvclass">)  [unwired: 7 in]
          n1024 = Equal?(x=w2664, y="DONE") -> (x = y?=w2662:bool)
          n1025 = case shown="True" w2662 {
            tunnel: [w2667 w2668] -> w2661
            tunnel: w2658 -> [w2667 w2669]
            frame False {
            }
            frame True {
              n1026 = Increment(x=w2669) -> (x+1=w2668:i32)
            }
          }
        }
        frame 290 {
          n1027 = call-dynamic "Write cmd.vi"("error in (no error)"=w2675, "cmd"="GET AD_CHANNEL", "Device in"=w2673) -> ("error out"=w2674:errorcluster, "Device out"=w2676:refnum<class "Channel.lvclass">)  [unwired: 7 in]
          n1028 = Increment(x=w2671) -> (x+1=w2672:i32)
        }
        frame 291 {
          n1029 = call-dynamic "Read resp.vi"("error in (no error)"=w2687, "Device in"=w2688) -> ("error out"=w2685:errorcluster, "resp"=w2680:string, "Device out"=w2683:refnum<class "Channel.lvclass">)  [unwired: 7 in]
          n1030 = Fract/Exp String To Number(string=w2680) -> (number=w2678:dbl)  [unwired: 3 in, 1 out]
          n1031 = Unbundle By Name(w2683) -> ("Interface.lvclass"=w2682:refnum<class "Interface.lvclass">)
          n1032 = call "Read Camera Setup.vi"("Interface in"=w2682) -> ("Camera Setup"=w2681:T4)  [unwired: 8 in, 2 out]
          n1033 = Unbundle By Name(w2681) -> ("AD_CHANNEL"=w2677:u32)
          n1034 = Equal?(x=w2677, y=w2678) -> (x = y?=w2679:bool)
          n1035 = case shown="True" w2679 {
            tunnel: [w2689 w2690] -> w2686
            tunnel: w2684 -> [w2689 w2691]
            frame False {
            }
            frame True {
              n1036 = Increment(x=w2691) -> (x+1=w2690:i32)
            }
          }
        }
        frame 300 {
          # "suffix"
          n1037 = call-dynamic "Write Timer.vi"("error in (no error)"=w2697, "Timer"=u32 200, "State Machine in"=w2700) -> ("error out"=w2701:errorcluster, "State Machine out"=w2695:refnum<class "State Machine.lvclass">)  [unwired: 7 in]
          n1038 = call-dynamic "Write State Machine.vi"("error in (no error)"=w2701, "State Machine.lvclass"=w2695, "Device in"=w2698) -> ("error out"=w2696:errorcluster, "Device out"=w2694:refnum<class "Channel.lvclass">)  [unwired: 7 in]
          n1039 = Bundle By Name(cluster=w2694, "config"=TRUE) -> (w2693:refnum<class "Channel.lvclass">)
          n1040 = Unbundle By Name(w2693) -> ("Interface.lvclass"=w2707:refnum<class "Interface.lvclass">)
          n1041 = call-dynamic "Read Suffix.vi"("Interface in"=w2707) -> ("Suffix"=w2702:string)  [unwired: 8 in, 2 out]
          n1042 = Concatenate Strings("SET SUFFIX " ("cmd"), w2702) -> (w2706:string)
          n1043 = call-dynamic "Write cmd.vi"("error in (no error)"=w2696, "cmd"=w2706, "Device in"=w2693) -> ("error out"=w2708:errorcluster, "Device out"=w2709:refnum<class "Channel.lvclass">)  [unwired: 7 in]
          n1044 = Increment(x=w2704) -> (x+1=w2705:i32)
        }
        frame 301 {
          # "Compara o parametro enviado com\no parametro no Acquisition Configuration\nda msg de STATUS do ACS."
          # "Verifica timeout para ACS responder.\nSe estourar timeout é porque o ACS não \nrespondeu e este canal volta para o estado 0\npara não \"travar\" os outros canais no \nS4ACS_GUI:HandleObservation.vi."
          n1045 = call "Verify Timer.vi"("error in (no error)"=w2741, "State Machine in"=w2743) -> ("error out"=w2740:errorcluster, "timeout"=w2738:bool, "State Machine out"=w2742:refnum<class "State Machine.lvclass">)  [unwired: 7 in]
          n1046 = call-dynamic "Write State Machine.vi"("error in (no error)"=w2740, "State Machine.lvclass"=w2742, "Device in"=w2744) -> ("error out"=w2739:errorcluster, "Device out"=w2735:refnum<class "Channel.lvclass">)  [unwired: 7 in]
          n1047 = call-dynamic "Read resp.vi"("error in (no error)"=w2739, "Device in"=w2735) -> ("error out"=w2729:errorcluster, "resp"=w2713:string, "Device out"=w2734:refnum<class "Channel.lvclass">)  [unwired: 7 in]
          n1048 = Unbundle By Name(w2734) -> ("Interface.lvclass"=w2733:refnum<class "Interface.lvclass">)
          n1049 = call-dynamic "UpdateACQconf.vi"("error in (no error)"=w2729, "status"=w2713, "Interface in"=w2733) -> ("error out"=w2728:errorcluster, "ACQ conf rx"=w2731:T2, "Interface out"=w2732:refnum<class "Interface.lvclass">)  [unwired: 6 in]
          n1050 = Unbundle By Name(w2731) -> ("suffix"=w2730:string)
          n1051 = call-dynamic "Read Suffix.vi"("error in (no error)"=w2728, "Interface in"=w2732) -> ("error out"=w2712:errorcluster, "Suffix"=w2727:string, "Interface out"=w2715:refnum<class "Interface.lvclass">)  [unwired: 7 in]
          n1052 = Equal?(x=w2727, y=w2730) -> (x = y?=w2726:bool)
          n1053 = call-dynamic "UpdateS4GUI_JSON_string.vi"("error in (no error)"=w2712, "status"=w2713, "Interface in"=w2715) -> ("error out"=w2711:errorcluster, "S4GUI JSON string rx"=w2710:T5, "Interface out"=w2714:refnum<class "Interface.lvclass">)  [unwired: 6 in]
          n1054 = Unbundle By Name(w2710) -> ("OBSTYPE"=w2719:string, "OBJECT"=w2718:string)
          n1055 = call-dynamic "Read ObsType.vi"("error in (no error)"=w2711, "Interface in"=w2714) -> ("error out"=w2724:errorcluster, "ObsType"=w2721:string, "Interface out"=w2722:refnum<class "Interface.lvclass">)  [unwired: 7 in]
          n1056 = call-dynamic "Read Object.vi"("error in (no error)"=w2724, "Interface in"=w2722) -> ("error out"=w2723:errorcluster, "Object"=w2720:string)  [unwired: 7 in, 1 out]
          n1057 = Equal?(x=w2721, y=w2719) -> (x = y?=w2717:bool)
          n1058 = Equal?(x=w2720, y=w2718) -> (x = y?=w2716:bool)
          n1059 = disable-structure shown="Enabled" {
            disable-tunnel: w2726 -> [w2748 w2749]
            disable-tunnel: [w2747 w2749] -> w2725
            disable-tunnel: w2717 -> [w2746 _]
            disable-tunnel: w2716 -> [w2745 _]
            frame Enabled {
              n1060 = Compound Arithmetic op=AND(w2748, w2746, w2745) -> (w2747:bool)
            }
            frame Disabled {
            }
          }
          n1061 = case shown="True" w2738 {
            tunnel: [w2751 27] -> w2736
            tunnel: w2737 -> [w2752 _]
            tunnel: w2725 -> [w2750 _]
            frame False {
              n1062 = case shown="False" w2750 {
                tunnel: [w2753 w2754] -> w2751
                tunnel: w2752 -> [w2753 w2755]
                frame False {
                }
                frame True {
                  n1063 = Increment(x=w2755) -> (x+1=w2754:i32)
                }
              }
            }
            frame True {
              # "ERRO"
            }
          }
        }
        frame 302 {
          # "Não espera nada."
          # "2024-03-20:\nSó envia o SUFFIX por comando SET.\nO resto dos parametros estão na  \npublicação do STATUS do S4GUI.\nVai para 40 configurar o EXPOSE mode"
          n1064 = call "Verify Timer.vi"("error in (no error)"=w2765, "State Machine in"=w2766) -> ("error out"=w2762:errorcluster, "State Machine out"=w2763:refnum<class "State Machine.lvclass">)  [unwired: 7 in, 1 out]
          n1065 = call-dynamic "Write State Machine.vi"("error in (no error)"=w2762, "State Machine.lvclass"=w2763, "Device in"=w2764) -> ("error out"=w2761:errorcluster, "Device out"=w2760:refnum<class "Channel.lvclass">)  [unwired: 7 in]
          n1066 = case shown="True" TRUE {
            tunnel: [w2767 0 ("State")] -> w2759
            tunnel: w2758 -> [w2767 _]
            frame False {
            }
            frame True {
              (unwired) 40 ("State")
            }
          }
        }
        frame 312 {
          # "filter"
          n1067 = call-dynamic "Write Timer.vi"("error in (no error)"=w2774, "Timer"=u32 50, "State Machine in"=w2772) -> ("error out"=w2779:errorcluster, "State Machine out"=w2777:refnum<class "State Machine.lvclass">)  [unwired: 7 in]
          n1068 = call-dynamic "Write State Machine.vi"("error in (no error)"=w2779, "State Machine.lvclass"=w2777, "Device in"=w2776) -> ("error out"=w2769:errorcluster, "Device out"=w2775:refnum<class "Channel.lvclass">)  [unwired: 7 in]
          n1069 = Unbundle By Name(w2775) -> ("Filter"=w2771:u8)
          n1070 = case shown="0, Default" w2771 {
            tunnel: ["U" ("cmd") "B" ("cmd") "V" ("cmd") "R" ("cmd") "I" ("cmd") "CLEAR" ("cmd")] -> w2770
            frame 1 {
            }
            frame 2 {
            }
            frame 3 {
            }
            frame 4 {
            }
            frame 5 {
            }
            frame 0, Default {
            }
          }
          n1071 = Concatenate Strings("SET FILTER " ("cmd"), w2770) -> (w2782:string)
          n1072 = call-dynamic "Write cmd.vi"("error in (no error)"=w2769, "cmd"=w2782, "Device in"=w2775) -> ("error out"=w2783:errorcluster, "Device out"=w2784:refnum<class "Channel.lvclass">)  [unwired: 7 in]
          n1073 = Increment(x=w2780) -> (x+1=w2781:i32)
        }
        frame 313 {
          n1074 = call "Verify Timer.vi"("error in (no error)"=w2799, "State Machine in"=w2797) -> ("error out"=w2798:errorcluster, "timeout"=w2794:bool, "State Machine out"=w2801:refnum<class "State Machine.lvclass">)  [unwired: 7 in]
          n1075 = call-dynamic "Write State Machine.vi"("error in (no error)"=w2798, "State Machine.lvclass"=w2801, "Device in"=w2800) -> ("error out"=w2795:errorcluster, "Device out"=w2796:refnum<class "Channel.lvclass">)  [unwired: 7 in]
          n1076 = call-dynamic "Read resp.vi"("error in (no error)"=w2795, "Device in"=w2796) -> ("error out"=w2802:errorcluster, "resp"=w2805:string, "Device out"=w2803:refnum<class "Channel.lvclass">)  [unwired: 7 in]
          n1077 = Equal?(x=w2805, y="DONE") -> (x = y?=w2792:bool)
          n1078 = case shown="False" w2794 {
            tunnel: [w2807 0] -> w2791
            tunnel: w2793 -> [w2808 _]
            tunnel: w2792 -> [w2806 _]
            frame False {
              n1079 = case shown="True" w2806 {
                tunnel: w2808 -> [w2809 w2811]
                tunnel: [w2809 w2810] -> w2807
                frame False {
                }
                frame True {
                  n1080 = Increment(x=w2811) -> (x+1=w2810:i32)
                }
              }
            }
            frame True {
            }
          }
        }
        frame 314 {
          n1081 = call-dynamic "Write Timer.vi"("error in (no error)"=w2816, "Timer"=u32 50, "State Machine in"=w2815) -> ("error out"=w2821:errorcluster, "State Machine out"=w2819:refnum<class "State Machine.lvclass">)  [unwired: 7 in]
          n1082 = call-dynamic "Write State Machine.vi"("error in (no error)"=w2821, "State Machine.lvclass"=w2819, "Device in"=w2818) -> ("error out"=w2814:errorcluster, "Device out"=w2817:refnum<class "Channel.lvclass">)  [unwired: 7 in]
          n1083 = call-dynamic "Write cmd.vi"("error in (no error)"=w2814, "cmd"="SET CTRLINTE S4GUI", "Device in"=w2817) -> ("error out"=w2824:errorcluster, "Device out"=w2825:refnum<class "Channel.lvclass">)  [unwired: 7 in]
          n1084 = Increment(x=w2822) -> (x+1=w2823:i32)
        }
        frame 315 {
          n1085 = call "Verify Timer.vi"("error in (no error)"=w2834, "State Machine in"=w2832) -> ("error out"=w2833:errorcluster, "timeout"=w2829:bool, "State Machine out"=w2836:refnum<class "State Machine.lvclass">)  [unwired: 7 in]
          n1086 = call-dynamic "Write State Machine.vi"("error in (no error)"=w2833, "State Machine.lvclass"=w2836, "Device in"=w2835) -> ("error out"=w2830:errorcluster, "Device out"=w2831:refnum<class "Channel.lvclass">)  [unwired: 7 in]
          n1087 = call-dynamic "Read resp.vi"("error in (no error)"=w2830, "Device in"=w2831) -> ("error out"=w2837:errorcluster, "resp"=w2840:string, "Device out"=w2838:refnum<class "Channel.lvclass">)  [unwired: 7 in]
          n1088 = Equal?(x=w2840, y="DONE") -> (x = y?=w2827:bool)
          n1089 = case shown="False" w2829 {
            tunnel: [w2842 0] -> w2826
            tunnel: w2828 -> [w2843 _]
            tunnel: w2827 -> [w2841 _]
            frame False {
              n1090 = case shown="True" w2841 {
                tunnel: w2843 -> [w2844 w2846]
                tunnel: [w2844 w2845] -> w2842
                frame False {
                }
                frame True {
                  n1091 = Increment(x=w2846) -> (x+1=w2845:i32)
                }
              }
            }
            frame True {
            }
          }
        }
        frame 316 {
          # "Carrega timeout de 50 ciclos\npara resposta do ACS"
          n1092 = call-dynamic "Write Timer.vi"("error in (no error)"=w2856, "Timer"=u32 50, "State Machine in"=w2855) -> ("error out"=w2858:errorcluster, "State Machine out"=w2860:refnum<class "State Machine.lvclass">)  [unwired: 7 in]
          n1093 = call-dynamic "Write State Machine.vi"("error in (no error)"=w2858, "State Machine.lvclass"=w2860, "Device in"=w2857) -> ("error out"=w2850:errorcluster, "Device out"=w2849:refnum<class "Channel.lvclass">)  [unwired: 7 in]
          n1094 = Unbundle By Name(w2849) -> ("rotator"=w2848:dbl)
          n1095 = Number To Fractional String(number=w2848) -> (F-format string=w2852:string)  [unwired: 3 in]
          n1096 = Concatenate Strings("SET INSTROT " ("cmd"), w2852) -> (w2851:string)
          n1097 = call-dynamic "Write cmd.vi"("error in (no error)"=w2850, "cmd"=w2851, "Device in"=w2849) -> ("error out"=w2862:errorcluster, "Device out"=w2863:refnum<class "Channel.lvclass">)  [unwired: 7 in]
          n1098 = Increment(x=w2854) -> (x+1=w2861:i32)
        }
        frame 317 {
          n1099 = call "Verify Timer.vi"("error in (no error)"=w2868, "State Machine in"=w2869) -> ("error out"=w2873:errorcluster, "timeout"=w2865:bool, "State Machine out"=w2874:refnum<class "State Machine.lvclass">)  [unwired: 7 in]
          n1100 = call-dynamic "Write State Machine.vi"("error in (no error)"=w2873, "State Machine.lvclass"=w2874, "Device in"=w2872) -> ("error out"=w2870:errorcluster, "Device out"=w2871:refnum<class "Channel.lvclass">)  [unwired: 7 in]
          n1101 = call-dynamic "Read resp.vi"("error in (no error)"=w2870, "Device in"=w2871) -> ("error out"=w2875:errorcluster, "resp"=w2878:string, "Device out"=w2876:refnum<class "Channel.lvclass">)  [unwired: 7 in]
          n1102 = Equal?(x=w2878, y="DONE") -> (x = y?=w2864:bool)
          n1103 = case shown="False" w2865 {
            tunnel: [w2880 0] -> w2867
            tunnel: w2866 -> [w2881 _]
            tunnel: w2864 -> [w2879 _]
            frame False {
              n1104 = case shown="True" w2879 {
                tunnel: [w2882 w2883] -> w2880
                tunnel: w2881 -> [w2882 w2884]
                frame False {
                }
                frame True {
                  n1105 = Increment(x=w2884) -> (x+1=w2883:i32)
                }
              }
            }
            frame True {
            }
          }
        }
        frame 318 {
          # "Carrega timeout de 50 ciclos\npara resposta do ACS"
          n1106 = call-dynamic "Write Timer.vi"("error in (no error)"=w2893, "Timer"=u32 50, "State Machine in"=w2892) -> ("error out"=w2895:errorcluster, "State Machine out"=w2897:refnum<class "State Machine.lvclass">)  [unwired: 7 in]
          n1107 = call-dynamic "Write State Machine.vi"("error in (no error)"=w2895, "State Machine.lvclass"=w2897, "Device in"=w2894) -> ("error out"=w2888:errorcluster, "Device out"=w2887:refnum<class "Channel.lvclass">)  [unwired: 7 in]
          n1108 = Unbundle By Name(w2887) -> ("TCS mode"=w2886:string)
          n1109 = Concatenate Strings("SET TCSMODE " ("cmd"), w2886) -> (w2889:string)
          n1110 = call-dynamic "Write cmd.vi"("error in (no error)"=w2888, "cmd"=w2889, "Device in"=w2887) -> ("error out"=w2899:errorcluster, "Device out"=w2900:refnum<class "Channel.lvclass">)  [unwired: 7 in]
          n1111 = Increment(x=w2891) -> (x+1=w2898:i32)
        }
        frame 319 {
          n1112 = call "Verify Timer.vi"("error in (no error)"=w2905, "State Machine in"=w2906) -> ("error out"=w2910:errorcluster, "timeout"=w2902:bool, "State Machine out"=w2911:refnum<class "State Machine.lvclass">)  [unwired: 7 in]
          n1113 = call-dynamic "Write State Machine.vi"("error in (no error)"=w2910, "State Machine.lvclass"=w2911, "Device in"=w2909) -> ("error out"=w2907:errorcluster, "Device out"=w2908:refnum<class "Channel.lvclass">)  [unwired: 7 in]
          n1114 = call-dynamic "Read resp.vi"("error in (no error)"=w2907, "Device in"=w2908) -> ("error out"=w2912:errorcluster, "resp"=w2915:string, "Device out"=w2913:refnum<class "Channel.lvclass">)  [unwired: 7 in]
          n1115 = Equal?(x=w2915, y="DONE") -> (x = y?=w2901:bool)
          n1116 = case shown="False" w2902 {
            tunnel: [w2917 0] -> w2904
            tunnel: w2903 -> [w2918 _]
            tunnel: w2901 -> [w2916 _]
            frame False {
              n1117 = case shown="True" w2916 {
                tunnel: [w2919 w2920] -> w2917
                tunnel: w2918 -> [w2919 w2921]
                frame False {
                }
                frame True {
                  n1118 = Increment(x=w2921) -> (x+1=w2920:i32)
                }
              }
            }
            frame True {
            }
          }
        }
        frame 320 {
          # "Carrega timeout de 50 ciclos\npara resposta do ACS"
          n1119 = call-dynamic "Write Timer.vi"("error in (no error)"=w2930, "Timer"=u32 50, "State Machine in"=w2929) -> ("error out"=w2932:errorcluster, "State Machine out"=w2934:refnum<class "State Machine.lvclass">)  [unwired: 7 in]
          n1120 = call-dynamic "Write State Machine.vi"("error in (no error)"=w2932, "State Machine.lvclass"=w2934, "Device in"=w2931) -> ("error out"=w2925:errorcluster, "Device out"=w2924:refnum<class "Channel.lvclass">)  [unwired: 7 in]
          n1121 = Unbundle By Name(w2924) -> ("ICS mode"=w2923:string)
          n1122 = Concatenate Strings("SET ICSMODE " ("cmd"), w2923) -> (w2926:string)
          n1123 = call-dynamic "Write cmd.vi"("error in (no error)"=w2925, "cmd"=w2926, "Device in"=w2924) -> ("error out"=w2936:errorcluster, "Device out"=w2937:refnum<class "Channel.lvclass">)  [unwired: 7 in]
          n1124 = Increment(x=w2928) -> (x+1=w2935:i32)
        }
        frame 321 {
          n1125 = call "Verify Timer.vi"("error in (no error)"=w2942, "State Machine in"=w2943) -> ("error out"=w2947:errorcluster, "timeout"=w2941:bool, "State Machine out"=w2948:refnum<class "State Machine.lvclass">)  [unwired: 7 in]
          n1126 = call-dynamic "Write State Machine.vi"("error in (no error)"=w2947, "State Machine.lvclass"=w2948, "Device in"=w2946) -> ("error out"=w2944:errorcluster, "Device out"=w2945:refnum<class "Channel.lvclass">)  [unwired: 7 in]
          n1127 = call-dynamic "Read resp.vi"("error in (no error)"=w2944, "Device in"=w2945) -> ("error out"=w2949:errorcluster, "resp"=w2952:string, "Device out"=w2950:refnum<class "Channel.lvclass">)  [unwired: 7 in]
          n1128 = Equal?(x=w2952, y="DONE") -> (x = y?=w2939:bool)
          n1129 = case shown="False" w2941 {
            tunnel: [w2954 w2960] -> w2938
            tunnel: w2940 -> [w2955 _]
            tunnel: w2939 -> [w2953 _]
            frame False {
              n1130 = case shown="True" w2953 {
                tunnel: [w2956 w2957] -> w2954
                tunnel: w2955 -> [w2956 _]
                frame False {
                }
                frame True {
                  n1131 = disable-structure shown="Enabled" {
                    disable-tunnel: [0 ("State") 40] -> w2957
                    frame Disabled {
                    }
                    frame Enabled {
                      # "Configura\nExpMode"
                    }
                  }
                }
              }
            }
            frame True {
              n1132 = disable-structure shown="Enabled" {
                disable-tunnel: [0 40] -> w2960
                frame Enabled {
                }
                frame Disabled {
                  # "Configura\nExpMode"
                }
              }
            }
          }
        }
      }
      n1133 = call-dynamic "Read State Machine.vi"("error in (no error)"=w7, "Device in"=w14) -> ("error out"=w10:errorcluster, "State Machine.lvclass"=w13:refnum<class "State Machine.lvclass">, "Device out"=w12:refnum<class "Channel.lvclass">)  [unwired: 7 in]
      n1134 = call "Next State.vi"("error in (no error)"=w10, "New_State"=w8, "State Machine in"=w13) -> ("error out"=w9:errorcluster, "State Machine out"=w15:refnum<class "State Machine.lvclass">)  [unwired: 7 in]
      n1135 = call-dynamic "Write State Machine.vi"("error in (no error)"=w9, "State Machine.lvclass"=w15, "Device in"=w12) -> ("error out"=w6:errorcluster, "Device out"=w11:refnum<class "Channel.lvclass">)  [unwired: 7 in]
    }
    frame Error {
    }
  }
  "error out" <- w3
  "Channel out" <- w1
